vi "main.vi"() -> ()   [LabVIEW 2024]
doc: "Use this template to build a producer/consumer design pattern with events to produce queue items. Use this design pattern instead of the User Interface Event Handler pattern for user interfaces when you want to execute code asynchronously in response to an event without slowing the user interface responsiveness."
uses:
  code/controls/type.eng.settings.ctl
  code/controls/UiStepBuilder.ctl
  code/controls/type.step-builder.ctl
  code/controls/UiProcHeader.ctl
  code/controls/Ui.nrt.flow-panel.ctl
  code/controls/UiNutritionFlowElement.ctl
  code/controls/UiScheduleTimestamp.ctl
  code/controls/typeEnv.ctl
  code/controls/type.StepFunction.ctl
  code/controls/typeXyPoint.ctl
  code/controls/type.address.ctl
  code/controls/enum.io.type.ctl
  code/controls/enum.io.mode.ctl
  code/controls/IONode.ctl
  code/controls/type-io-map-do.ctl
  code/controls/type-io-map-di.ctl
  code/controls/type-io-map-ai.ctl
  code/controls/type-snapshot.ctl
  code/controls/enum-io-sort-type.ctl
  code/controls/wind-dir-view.ctl
  code/controls/windows-panel.ctl
  code/controls/irr-panel.ctl
  code/controls/pbr-func-def.ctl
  code/controls/eng-serial-log.ctl
  code/controls/cluster-com-log.ctl
  code/controls/state-engine.ctl
  code/controls/state-logger.ctl
  code/controls/enum.io-interface.ctl
  code/controls/enum-com-log.ctl
  code/controls/enum.report-filter.ctl
  code/controls/typePathSelector.ctl
  code/controls/ini-key.ctl
  code/controls/typeProcVarientName.ctl
  code/controls/UiNutritionPanel.ctl
  code/controls/enumVarCtrlIO.ctl
  code/controls/type.eng-call.proc-insert.ctl
  code/controls/type.eng.proc.isrunning.ctl
  code/controls/eng-call-do-by-name.ctl
  <vilib>/Utility/error.llb/DialogType.ctl
  <vilib>/Utility/miscctls.llb/LVPointTypeDef.ctl
  <vilib>/Utility/miscctls.llb/LVDateTimeRec.ctl
  code/controls/rio-rx-enum.ctl
  code/controls/type.eng.log-cluster.ctl
  code/controls/typeCmdPostStepFunc.ctl
  code/controls/typeEngineLogCluster.ctl
  code/VIs/Polymorphics/variantCtrlString.vi
  code/VIs/proc.util.validateParamExist.vi
  <vilib>/Utility/error.llb/Trim Whitespace.vi
  <vilib>/Utility/error.llb/Trim Whitespace One-Sided.vi
  code/globals/globals-engine.vi
  <vilib>/Utility/libraryn.llb/Create Directory Recursive.vi
  <vilib>/Utility/config.llb/Read Key (String).vi
  code/VIs/util.error.create.vi
  <vilib>/Utility/config.llb/Read Key (Double).vi
  <vilib>/Utility/config.llb/Read Key (I32).vi
  code/VIs/util-address-builder.vi
  code/VIs/util.DO.ToString.vi
  code/VIs/Polymorphics/io.command-builder.vi
  code/VIs/Polymorphics/io.command-builder.DO.vi
  code/VIs/Polymorphics/io.command-builder.AI.vi
  code/VIs/Polymorphics/io.command-builder.DI.vi
  <vilib>/Utility/config.llb/Write Key (String).vi
  <vilib>/Utility/config.llb/Write Key (Double).vi
  <vilib>/Utility/config.llb/Write Key (I32).vi
  code/controls/typeIniFileSection.ctl
  <vilib>/Utility/file.llb/Read Delimited Spreadsheet (DBL).vi
  <vilib>/Utility/config.llb/NI_LVConfig.lvlib
  <vilib>/Instr/_visa.llb/VISA Find Search Mode.ctl
  <vilib>/Utility/file.llb/Write Delimited Spreadsheet (DBL).vi
panel:
  out "clock 3":string="12:34:56"
  out "COM Size":i64 format="IOs: %d"
  out "COM FIFO":i32 format="QCom: %d"
  out "LOG FIFO 2":i32 format="QLog: %d"
  out "ENG FIFO 2":i32 format="QEng: %d"
  in  "Cluster":cluster{"MAIN":bool, "I/O":bool, "ADMIN":bool}
  out "DayNight":bool
  in  "ENG ms ctrl 28":i32=300 caption="Runtime Interval" format="Runtime:  %d [ms]"
  in  "ENG ms ctrl 15":i32=300 caption="Runtime Interval" format="Runtime:  %d [ms]"
  in  "ENG ms ctrl 14":i32=300 caption="Runtime Interval" format="Runtime:  %d [ms]"
  in  "ENG ms ctrl 13":i32=300 caption="Runtime Interval" format="Runtime:  %d [ms]"
  in  "ENG ms ctrl 12":i32=300 caption="Runtime Interval" format="Runtime:  %d [ms]"
  in  "ENG ms ctrl 11":i32=300 caption="Runtime Interval" format="Runtime:  %d [ms]"
  in  "ENG ms ctrl 10":i32=300 caption="Runtime Interval" format="Runtime:  %d [ms]"
  in  "ENG ms ctrl 9":i32=300 caption="Runtime Interval" format="Runtime:  %d [ms]"
  in  "ENG ms ctrl 8":i32=300 caption="Runtime Interval" format="Runtime:  %d [ms]"
  in  "Admin Panel":bool
  out "Waveform Chart":dbl(graph)
  out "User messages":string
  out "error out":errorcluster
  in  "Timer Reset?":bool
  out "userName":string="USER"
  out "projectName":string="NAME"
  in  "ENV":T1=enum."ENV.TEST.SINGLE-02"
  out "clock":string="12:34:56"
  in  "Enable Report":bool
  in  "Tab Control 2":T2(tab)
  in  "EngLogClear":bool
  out "Collected Reports":string
  out "Collected Reports 2":string
  in  "VISA REPORT":T4={"visa report"=[["Range", "High", "Low", "25", "FULL"], ["", "", "", "", ""], ["", "", "", "", ""], ["", "", "", "", ""], ["", "", "", "", ""], ["", "", "", "", ""], ["", "", "", "", ""], ["", "", "", "", ""], ["", "", "", "", ""]], "RIO Address"=0, "IOtype"=enum."AI", "VISA Report En"=FALSE, "Clear"=FALSE, "Only Errors?"=FALSE} {"RIO Address" min=-1 max=31 step=1 format="RIO: %02d"}
  out "SelectedPath":path
  out "case":T5
  in  "Clk Simulator":timestamp format="%<%x %.1X>T"
  in  "Simulate Clock Reset":bool
  out "Clock Simulation":bool
  in  "Time Addition":dbl
  out "AI":dbl[][](array[numeric]) format="%#.1f"
  in  "Calib?":bool
  out "Log":i32 format="%#_3p"
  out "Eng":i32 format="%#_3p"
  out "Event":i32 format="%#_3p"
  out "Com":i32 format="%.0p"
  out "Report General":T7(array[cluster]) {"clk" format="%#.1f"}
  in  "Log Clear":bool
  in  "Proc Name":string(combo)
  in  "DO Set by Addr":T9 {"ADDR" format="%04d"}
  in  "DO Set by Name":T10={"State"=FALSE, "Name"="Name...", "Timeout [s]"=8, "Send"=FALSE}
  in  "SerialPort":refnum<visa-resource-name>="COM12"
  in  "MenuRuntime":T11={"Run"=FALSE, "Step"=FALSE, "Load"=FALSE, "Status"=FALSE, "Unload"=FALSE, "Reload"=FALSE, "Stop"=FALSE, "ProcedureReload"=FALSE, "ProcedureStep"=FALSE, "ProcedureSelect"="set-dout", "ProcedureRun"=FALSE}
  out "Simulated":string[](array[string])
  in  "ProjectSettings":T12={"Project Name"="Yogiland", "Latitude"=0.0, "Longitude"=0.0, "TimeZone"=0, "userName"="Yogiland"} {"Longitude" format="%#.6g"; "Latitude" format="%#.6g"}
  out "RIO Snapshots":T13[](array[typedef]) {"Dports" format="%08x"}
  in  "Tab Main":enum32{"MAIN", "I/O", "ADMIN"}(tab)
  in  "Button":bool
  in  "Section":string(combo)
  in  "Tab NTR":T14(tab)
  in  "NTR Flowchart":T15={"WASH_IN"={"boolean"=FALSE, "Message"="25/150"}, "EC"={"boolean"=TRUE, "Message"="L Alarm"}, "PH"={"boolean"=TRUE, "Message"="Low"}, "ORP"={"boolean"=TRUE, "Message"="Range"}, "W_TEMP"={"boolean"=TRUE, "Message"="25"}, "W_LEVEL"={"boolean"=TRUE, "Message"="FULL"}, "ALFA1"={"boolean"=TRUE, "Message"="60/60"}, "BETA1"={"boolean"=TRUE, "Message"="25/60"}, "ALFA2"={"boolean"=FALSE, "Message"="0/0"}, "BETA2"={"boolean"=FALSE, "Message"="0/0"}, "ACID"={"boolean"=FALSE, "Message"="0/60"}, "BASE"={"boolean"=FALSE, "Message"="0/50"}, "WATER"={"boolean"=FALSE, "Message"="0/150"}, "WASH_OUT"={"boolean"=FALSE, "Message"="ss"}, "UNIT"={"boolean"=FALSE, "Message"="0"}, "ORPMIX"={"boolean"=FALSE, "Message"="0/150"}}
  out "ntr.status-table":string[][](table)=[["Range", "High", "Low", "25", "FULL"], ["", "", "", "", ""], ["", "", "", "", ""], ["", "", "", "", ""], ["", "", "", "", ""], ["", "", "", "", ""], ["", "", "", "", ""], ["", "", "", "", ""], ["", "", "", "", ""]]
  out "NTR Status":string="Nutrition Status: Processing Unit "
  in  "ntrGraphPeriod":T18 {"lastDays" format="Last %d Days"; "Time range"."Start" format="From: %<%d/%m/%y>T"; "Time range"."End" format="To: %<%d/%m/%y>T"}
  out "Nutrition Sensor Graph":cluster{"X":dbl[], "Y":dbl[]}(graph)
  out "EC 3":cluster{"X":dbl[], "Y":dbl[]}(graph)
  in  "ntrDosepumpSelect":string(combo)
  in  "ntrInputSelect":string(combo)
  in  "Irrigation status":string="Irrigation Status"
  out "Solar Elevation Graph":waveform(dbl)(graph)
  in  "UiProjectSettings":T19 {"Longitude" format="%#.6g"; "Latitude" format="%#.6g"}
  in  "GoToCam 2":bool
  in  "GoToCam":bool
  in  "Cluster 2":T20
  in  "camera":u16(ring) items=["Camera 1", "Camera 2"]
  in  "start":T17 caption="Open" format="%<%H:%M>T"
  out "last":T17 caption="Open" format="Last Harvest %<%H:%M:%S %d/%m/%y>T"
  in  "PRBmenu":cluster{"Harvest":bool, "SANI":bool}
  in  "PbrView 2":T21 {"Unit Storage"."col" scale=0.0..1.0; "Unit Storage"."?" scale=0.0..1.0; "Unit Storage"."?" scale=0.0..1.0; "Unit Column"."col" scale=0.0..1.0; "Unit Column"."?" scale=0.0..1.0; "Unit Column"."?" scale=0.0..1.0; "Digester"."Digester 2" scale=0.0..10.0; "Digester"."Digester 1" scale=0.0..10.0; "BIO Mass Tank" scale=0.0..100.0; "Harvest\n Tank" scale=0.0..100.0}
  in  "PBR Builder":T23(array[cluster])
  out "source":string
  in  "PBR_PLAY":cluster{"PLAY":bool, "PAUSE":bool, "STOP":bool}
  in  "PBR PROC":string(combo)
  in  "PBR":T24
  in  "Temperature Graph Panel":T25={"Time range"={"Start"=timestamp(0 s since 1904-01-01), "End"=timestamp(0 s since 1904-01-01)}, "lastDays"=3, "refresh"=FALSE} {"lastDays" min=1 max=99 step=1 format="%d Days"; "Time range"."Start" format="From: %<%d/%m/%y>T"; "Time range"."End" format="To: %<%d/%m/%y>T"}
  out "OutdoorStatus":T26
  out "indoorStatus":T27
  in  "Tab Control 3":T28(tab)
  out "Outdoor Tdry Graph":cluster{"X":dbl[], "Y":dbl[]}[](graph)
  out "RH":cluster{"X":dbl[], "Y":dbl[]}[](graph)
  out "UV Graph":cluster{"X":dbl[], "Y":dbl[]}(graph)
  in  "UVAccHistoryDays":i8=3
  out "UV_ACC":cluster{"X":dbl[], "Y":dbl[]}(graph)
  out "Waveform Chart 2":cluster{dbl, "UV Limit":dbl}(graph)
  in  "UvAccRefresh":bool
  out "UV Graph 2":cluster{"X":dbl[], "Y":dbl[]}(graph)
  out "Wind Dir Panel":T29
  out "UV Acc.":dbl format="%#_3p"
  in  "Tab Auxi":T30(tab)
  in  "IRR Params":T31={"Day Time"={"Sunset"=timestamp(0 s since 1904-01-01), "Sunrise"=timestamp(0 s since 1904-01-01)}, "timeLimits"={"Irrigation"=0.0, "Nut./Water"=0.0}, "Calculated Timing"={"Irrigation Timeout"=timestamp(0 s since 1904-01-01), "Nutrients Timeout"=timestamp(0 s since 1904-01-01)}, "Irr Dosing Time"={"Nutrients"=0, "Water"=0, "Wash"=0}, "UV Limit "=0.0, "Dose Table"=[{"Enable"=FALSE, "output"="IRR_SEC1"}, {"Enable"=FALSE, "output"="IRR_SEC2"}, {"Enable"=FALSE, "output"="IRR_SEC3"}, {"Enable"=FALSE, "output"="IRR_SEC4"}, {"Enable"=FALSE, "output"="IRR_SEC5"}, {"Enable"=FALSE, "output"="IRR_SEC6"}], "Last Iteration"=timestamp(0 s since 1904-01-01), "UV Reduction Status"=FALSE, "UV Reduction"=0} {"UV Reduction" max=99 step=1 format="%d [%%]"; "timeLimits"."Nut./Water" format="%02.2f [hr]"; "timeLimits"."Irrigation" format="%02.2f [hr]"; "Day Time"."Sunrise" format="%<%H:%M:%S>T"; "Day Time"."Sunset" format="%<%H:%M:%S>T"; "Calculated Timing"."Nutrients Timeout" format="%<%H:%M:%S>T"; "Calculated Timing"."Irrigation Timeout" format="%<%H:%M:%S>T"; "UV Limit" format="%#.1p [J/m2]"; "Irr Dosing Time"."Wash" format="%d [s]"; "Irr Dosing Time"."Water" format="%d [s]"; "Irr Dosing Time"."Nutrients" format="%d [s]"; "Last Iteration" format="%<%X %x>T"}
  in  "WinView":T32 {"EastSideView" scale=0.0..100.0; "WestSideView" scale=0.0..8.0; "EastPosition" max=12; "WestPosition" max=12}
  in  "AuxiliaryList":T33(array[cluster]) {"Period" format="Period [s]: %d"; "Pulse" format="Pulse [s]: %d"}
  out "Array 2":cluster{"name":string, "value":string}[](array[cluster])
  in  "NTR Panel":cluster{"CloseAll":bool}
  in  "RFS Enable Table":bool
  in  "RFS Enable Table":T34
  in  "RFS Cycles Set":bool
  in  "RFS Cycles":u16
  out "RFS Cycles":u16
  in  "RFS Cycles Get":bool
  out "RFS Status":string
  in  "RFS SetX1":bool
  in  "TableIndex":u8 max=7 step=1 format="Table: %d"
  in  "RFS SetX8":bool
  in  "RFS Delays":T35
  in  "RFS Address":u8 format="Address: %d"
  out "RFS Cycles Table":T36
  out "elements":cluster{"case":T5, "data":variant}[](array[cluster])
  in  "Tab IO":enum32{"Map", "Editor", "Calibration"}(tab)
  in  "Clear Virtuals":bool
  in  "IO Map Take Snapshot":bool caption="Take Snapshop"
  out "RIO List":cluster{"Address":u8, "Connected":bool}[](array[cluster]) {"Address" format="%02d"}
  in  "Show Undefined":bool
  out "IO Map AI Count":i32
  out "IO Map DI Count":i32
  out "IO Map DO Count":i32
  in  "IO Map DO":T37[](array[typedef]) caption="Digital Outputs" {"ADDR" format="%04d"}
  in  "IO Map AI":T39[](array[typedef]) caption="Analog Inputs" {"ADDR" format="%04d"}
  in  "IO Map DI":T40[](array[typedef]) caption="Digital Inputs" {"ADDR" format="%04d"}
  in  "IO Map Snapshot Enable":bool caption="Auto Snapshop Enable"
  in  "IO Search Map":T41={"By Name"="", "By Tag"="Tags...", "By Address"=0} caption="Search by Name | Tag | Address" {"By Address" min=-1 max=31 step=1 format="RIO: %02d"}
  in  "IO Search Map Refresh":bool
  in  "TimerSec":dbl=5.0 format="%#.1f"
  out "downcount[sec]":dbl format="%#.1g"
  in  "Simulators":cluster{"Input ":string, "Value":string}[](array[cluster])
  in  "IO Map VL":T42[](array[typedef]) caption="Virtual Channels" {"calibration"."Y" format="%#.3f"; "calibration"."X" format="%#.3f"; "ADDR" format="%04d"}
  out "IO Map VL Count":i32
  in  "IO Conf view":enum16{"Show All", "Search"}(ring)
  in  "IOconf Sort":T44
  in  "IO Search Conf":T45={"ADDR"=-1, "Label"="", "Type"=enum."Type", "Mode"=enum."Mode", "Tags"=""} {"ADDR" min=-1 max=99 format="RIO: %02d"}
  in  "IO Conf":T46(array[cluster]) {"calibration"."Y" format="%#.3f"; "calibration"."X" format="%#.3f"; "ADDR" format="%04d"}
  in  "IO List":cluster{"save":bool, "loadCsv":bool}
  in  "New Element":T42={"ADDR"=0, "Label"="Name", "Type"=enum."DI", "Mode"=enum."RIO", "Value"="Value", "Tags"="Tags", "calibration"=[]} {"calibration"."Y" format="%#.3f"; "calibration"."X" format="%#.3f"; "ADDR" format="%04d"}
  in  "IO Add New":bool
  out "size":i32 format="Count: %d"
  out "Value (Y)":dbl
  out "Raw (X)":dbl
  in  "IO calib save":bool
  in  "IO calib select":string(combo)
  in  "XyPairs":T43[](array[typedef]) {"Y" format="%#.3f"}
  out "error":errorcluster
  out "Chart":cluster{"unCalibrated":u16, "Value out":dbl}(graph)
  in  "Tab Control":enum32{"Settings", "Builder", "Snapshot"}(tab)
  out "App Started at":timestamp format="%<%x %.3X>T"
  out "Loaded":cluster{"Procedure":variant[]}[](array[cluster]) caption="Loaded Procedures"
  in  "ENG ms":i32=-1 caption="Interval"
  in  "Title Bar Visible":bool
  in  "ENG ms ctrl":i32=300 caption="Runtime Interval" format="Runtime:  %d [ms]"
  in  "EVENT ms":i32=100 format="%d [ms]"
  out "Type":u8 format="%.0x"
  out "Address":u8 format="%.0x"
  in  "read buffer":string
  out "Command Payload":string
  out "AI uncalib out":u16
  out "AI out":dbl
  out "Data Size":u8
  out "monitor":errorcluster[](array[cluster])
  out "record":errorcluster[](array[cluster])
  out "control":errorcluster[](array[cluster])
  in  "Template":T47
  in  "UiBuildProcHead":T48={"Procedure Name"="MyProcExample", "Running"=TRUE, "tags"="MyProcExample"}
  in  "Loaded Proc Path":string[](array[string])
  in  "UiBuildSteps":T49[](array[typedef])
  in  "File path":path
  out "UiBuildSteps 2":T49[](array[typedef])
  in  "Proc Select 2":string(combo)
  out "Serial Log Size":i32
  out "COM Snapshot":T51[](array[typedef])
  in  "Snapshot Size":i64=1000
  in  "COM":bool
  in  "filter":T52={"Status"=0, "Date"="", "Caller"="", "Type"="", "IOname"="", "Calib"="", "Uncalib"="", "Vsdt"="Vsdt", "StatusMsg"=""}
  out "Serial Record(s)":T53[](array[typedef]) {"IOnode"."calibration"."Y" format="%#.3f"; "IOnode"."calibration"."X" format="%#.3f"; "IOnode"."ADDR" format="%04d"}
  # "Outoor"
  # "Indoor"
  # "UV Accumulator"
  # "Nutrition"
  # "Nutrition History"
  # "Nursery"
  # "Camera Robot"
  # "PBR"
  # "- Fully Open"
  # "- Fully Close"
  # "W"
  # "E"
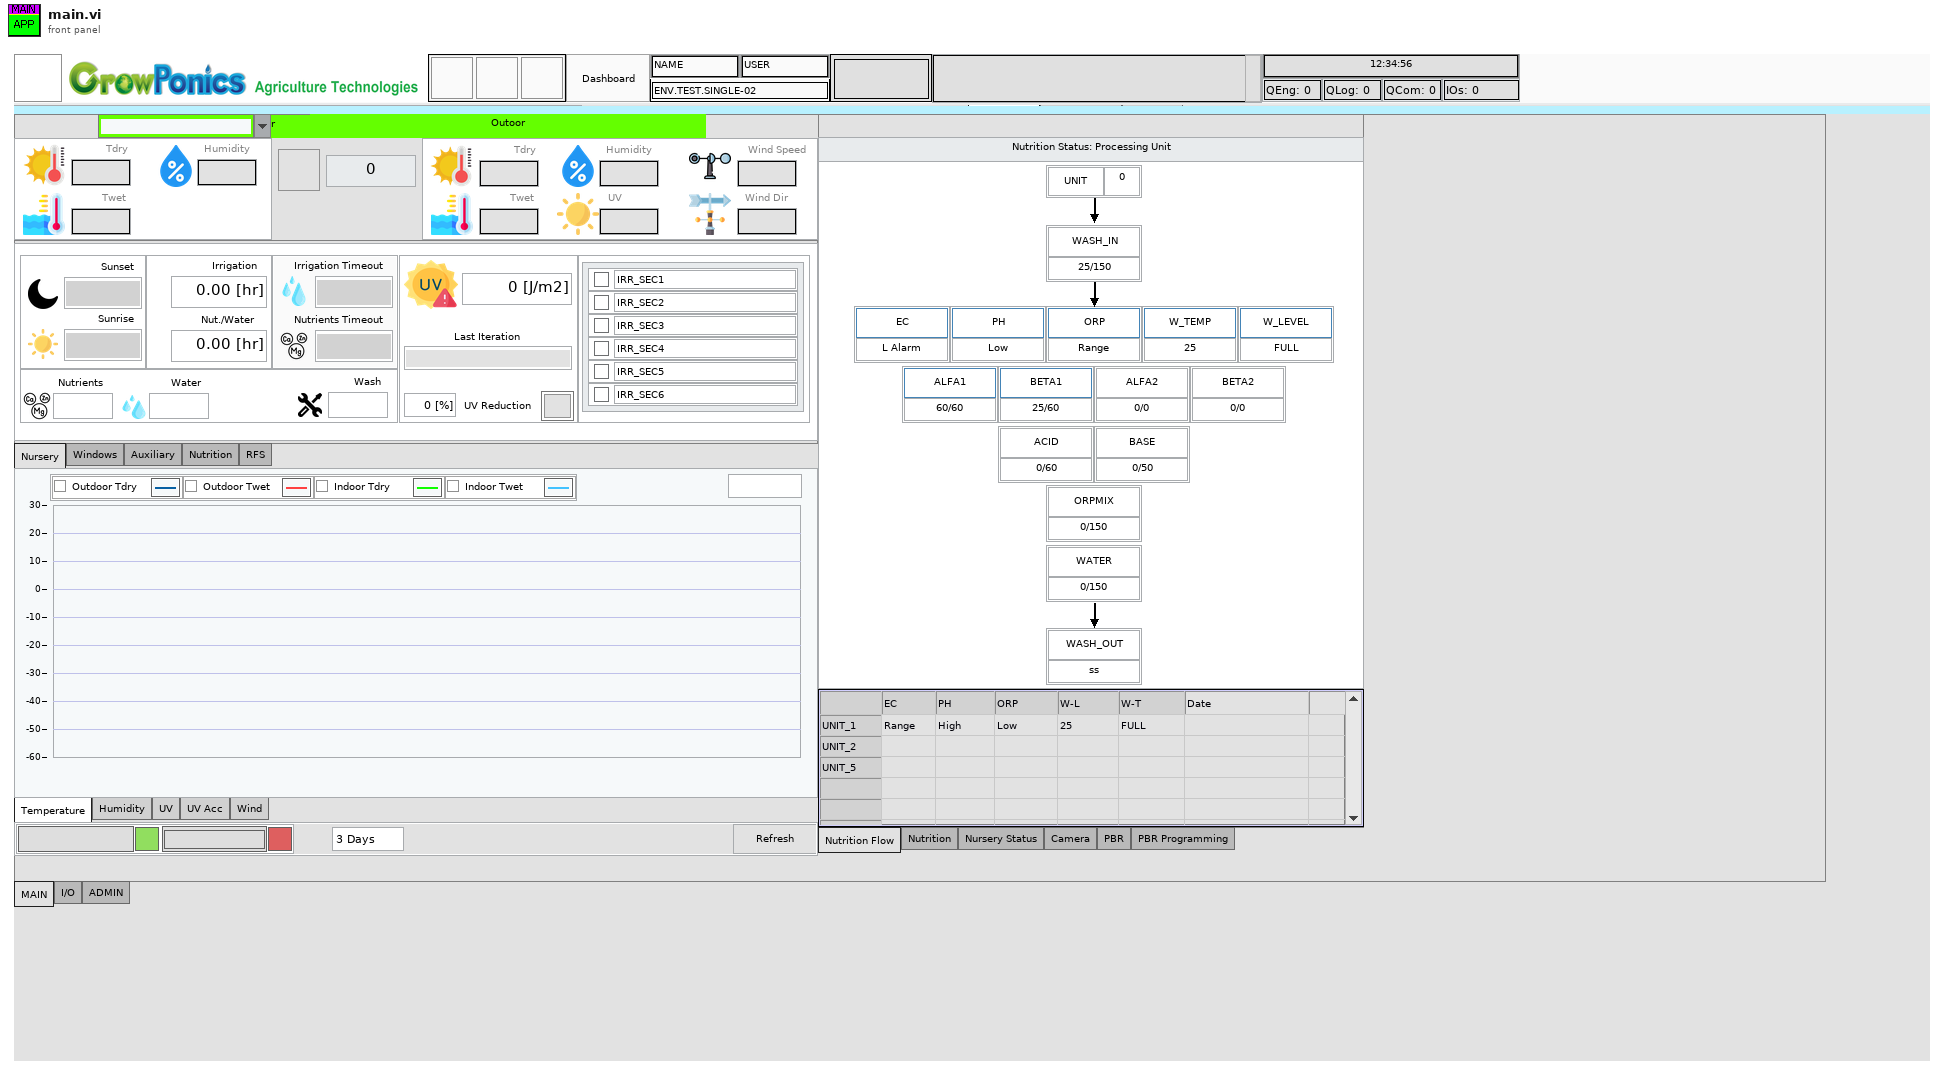
[diagram p1: front panel]
types:
  T1 = typedef "typeEnv.ctl" = enum16{"ENV.PRODUCTION", "ENV.TEST.NO-HW", "ENV.TEST.SINGLE-01", "ENV.TEST.SINGLE-02", "ENV.TEST.SINGLE-02 AI 0", "ENV.TEST.SINGLE-03"}
  T2 = enum32{"System Log", "Runtime Flow", "Iterations"}
  T3 = typedef "enum.io.type.ctl" = enum16{"Type", "DI", "DO", "AI", "AO", "VL", "BUF"}
  T4 = cluster{"visa report":string[][], "RIO Address":i32, "IOtype":T3, "VISA Report En":bool, "Clear":bool, "Only Errors?":bool}
  T5 = typedef "state-engine.ctl" = enum16{"ENG.NO-OP", "ENG.START", "ENG.STOP", "ENG.EXECUTE", "ENG.STATUS", "ENG.EXTERNAL-CALL", "ENG.INIT", "ENG.INIT.VARS", "ENG.INIT.SERIAL", "ENG.LOAD", "ENG.LOAD.SINGLE", "ENG.LOAD.MODULE", "ENG.LOAD.RELOAD", "ENG.LOAD.UNLOAD", "ENG.IO.LOAD", "ENG.IO.SAVE", "ENG.PROC.RELOAD-BY-NAME", "ENG.PROC.START", "ENG.PROC.STOP", "ENG.PROC.INSERT-STEPS", "ENG.PROC.ISRUNNING", "ENG.PROC.PRESET", "ENG.PROC.STATUS", "ENG.PRINT-USER-MSG", "ENG.RIO.SNAPSHOT", "ENG.RIO.AIN-SNAPSHOT-CALIB", "ENG.RIO.DOUT-BY-ADDR", "ENG.RIO.DOUT-BY-NAME", "ENG.RIO.RFS-DELAY-SET-X1", "ENG.RIO.RFS-DELAY-SET-X8", "ENG.RIO.RFS-CYCLES-SET", "ENG.RIO.RFS-CYCLES-GET", "ENG.RIO.RFS-ENABLE", "ENG.EXIT"}
  T6 = typedef "type.StepFunction.ctl" = enum16{"__NO-OP", "_DELAY_LOAD", "_DELAY_COMPARE", "_JUMP", "_COMPLETE", "_COMPARE", "_LOG_MESSAGE", "_LOG_LAST_REPORT", "_SCHEDULE", "_SCHED_DAILY", "CLK_COMPARE", "PROC_START", "PROC_STOP", "PROC_LOAD", "PROC_COMPLETION_CHECK", "PROC_COMPLETION_LOAD", "_IO_READ", "_IO_READ_MANY", "_IO_WRITE", "_IO_WRITE_BY_REG", "_IO_GET_OUTPUT", "_OCS_CHECK", "_OCS_RECORD", "_GET_RH", "_GET_ACC_UV", "_GET_WD", "_GET_WS", "_REC_DELETE", "_REC_MOVE", "_REC_COPY", "_IRR_CHECK", "UNIT_CHECK", "UNIT_SAMPLE", "UNIT_DOSE"}
  T7 = cluster{"ErrorFlag":bool, "idx":i32, "Step Name":string, "Step Function":T6, "Report":string, "clk":dbl, "Step Name 2":string}[]
  T8 = typedef "type.address.ctl" = u16
  T9 = cluster{"State":bool, "ADDR":T8, "Timeout [s]":u8, "Send":bool}
  T10 = cluster{"State":bool, "Name":string, "Timeout [s]":u8, "Send":bool}
  T11 = cluster{"Run":bool, "Step":bool, "Load":bool, "Status":bool, "Unload":bool, "Reload":bool, "Stop":bool, "ProcedureReload":bool, "ProcedureStep":bool, "ProcedureSelect":string, "ProcedureRun":bool}
  T12 = typedef "type.eng.settings.ctl" = cluster{"Project Name":string, "Latitude":dbl, "Longitude":dbl, "TimeZone":i32, "userName":string}
  T13 = typedef "type-snapshot.ctl" = cluster{"Address":u8, "DI":bool[], "status":errorcluster, "AI":dbl[], "Dports":u32, "AI RAW":dbl[]}
  T14 = enum32{"Nutrition Flow", "Nutrition", "Nursery Status", "Camera", "PBR", "PBR Programming"}
  T15 = typedef "Ui.nrt.flow-panel.ctl" = cluster{"WASH_IN":T16, "EC":T16, "PH":T16, "ORP":T16, "W_TEMP":T16, "W_LEVEL":T16, "ALFA1":T16, "BETA1":T16, "ALFA2":T16, "BETA2":T16, "ACID":T16, "BASE":T16, "WATER":T16, "WASH_OUT":T16, "UNIT":cluster{"boolean":bool, "Message":string}, "ORPMIX":T16}
  T16 = typedef "UiNutritionFlowElement.ctl" = cluster{"boolean":bool, "Message":string}
  T17 = typedef "UiScheduleTimestamp.ctl" = timestamp
  T18 = cluster{"Time range":cluster{"Start":T17, "End":T17}, "lastDays":dbl, "refresh":bool}
  T19 = cluster{"Latitude":dbl, "Longitude":dbl, "TimeZone":i32}
  T20 = cluster{"Next Button":bool, "Previous Button":bool, "Up Button":bool, "Down Button":bool, "Home":bool}
  T21 = cluster{"Unit Storage":cluster{dbl, dbl, "col":dbl}, "Unit Column":cluster{dbl, dbl, "col":dbl}, "Ui_TANKOUT":bool, "Column":dbl, "Ui MAIN\nUi_COLOUT\nUi_PUMP":bool, "Digester":cluster{"Digester 1":dbl, "Digester 2":dbl}, "DO 4":bool, "Flow Out DI":bool, "BIO Mass Tank":dbl, "DO Membrane":bool, "MEDIUM":bool, "WATER":bool, "Ui_TANKIN":bool, "Harvest\n Tank":dbl, "HARVEST":bool}
  T22 = typedef "pbr-func-def.ctl" = enum16{"DELAY SEC", "SENSE", "PROC START", "PROC WAIT", "SET OUTPUT", "FINISH"}
  T23 = cluster{"Operation":T22, "Param":string, "uid":string}[]
  T24 = cluster{"LOAD":bool, "SAVE":bool, "COMPILE":bool, "SAVEAS":bool}
  T25 = cluster{"Time range":cluster{"Start":T17, "End":T17}, "lastDays":i8, "refresh":bool}
  T26 = cluster{"Tdry":string, "Twet":string, "UV":string, "Humidity":string, "Wind Speed":string, "Wind Direction":string}
  T27 = cluster{"Tdry":string, "Twet":string, "Humidity":string}
  T28 = enum32{"Temperature", "Humidity", "UV", "UV Acc", "Wind"}
  T29 = typedef "wind-dir-view.ctl" = cluster{"SE":bool, "SW":bool, "NE":bool, "NW":bool, "W":bool, "E":bool, "S":bool, "N":bool}
  T30 = enum32{"Nursery", "Windows", "Auxiliary", "Nutrition", "RFS"}
  T31 = typedef "irr-panel.ctl" = cluster{"Day Time":cluster{"Sunset":timestamp, "Sunrise":timestamp}, "timeLimits":cluster{"Irrigation":dbl, "Nut./Water":dbl}, "Calculated Timing":cluster{"Irrigation Timeout":timestamp, "Nutrients Timeout":timestamp}, "Irr Dosing Time":cluster{"Nutrients":u16, "Water":u16, "Wash":u16}, "UV Limit ":dbl, "Dose Table":cluster{"Enable":bool, "output":string}[], "Last Iteration":timestamp, "UV Reduction Status":bool, "UV Reduction":u8}
  T32 = typedef "windows-panel.ctl" = cluster{"EastPosition":u16, "WestPosition":u16, "Wind Direction":string, "CloseAll":bool, "WestSideView":u16, "EastSideView":u16, "Wind Speed":string, "confs":cluster{"Full Open [sec]":u16, "Full Close [sec]":u16, "Stages":u16}}
  T33 = cluster{"Source":string, "SourceStatus":bool, "Dest":string, "DestStatus":bool, "Pulse":u16, "Period":u16, "Proc Name":string}[]
  T34 = cluster{"[0]":bool, "[1]":bool, "[2]":bool, "[3]":bool, "[4]":bool, "[5]":bool, "[6]":bool, "[7]":bool}
  T35 = cluster{"Delay Y":u8, "Delay X1":u8, "Delay X2":u8, "Delay CT":u8}
  T36 = cluster{"[0]":u16, "[1]":u16, "[2]":u16, "[3]":u16, "[4]":u16, "[5]":u16, "[6]":u16, "[7]":u16}
  T37 = typedef "type-io-map-do.ctl" = cluster{"ADDR":T8, "Label":string, "Mode":T38, "Value":string, "State":bool}
  T38 = typedef "enum.io.mode.ctl" = enum16{"Mode", "RIO", "SIM"}
  T39 = typedef "type-io-map-ai.ctl" = cluster{"ADDR":T8, "Label":string, "Mode":T38, "Value":string}
  T40 = typedef "type-io-map-di.ctl" = cluster{"ADDR":T8, "Label":string, "Mode":T38, "State":bool, "Value":string}
  T41 = cluster{"By Name":string, "By Tag":string, "By Address":i32}
  T42 = typedef "IONode.ctl" = cluster{"ADDR":T8, "Label":string, "Type":T3, "Mode":T38, "Value":string, "Tags":string, "calibration":T43[]}
  T43 = typedef "typeXyPoint.ctl" = cluster{"X":dbl, "Y":dbl}
  T44 = typedef "enum-io-sort-type.ctl" = enum16{"Sort By Address", "Sort By Name"}
  T45 = cluster{"ADDR":i8, "Label":string, "Type":T3, "Mode":T38, "Tags":string}
  T46 = cluster{"ADDR":T8, "Label":string, "Type":T3, "Mode":T38, "Value":string, "Tags":string, "calibration":T43[]}[]
  T47 = cluster{"templateSave":bool, "templateLoad":bool, "procedureLoad":bool, "procedureSaveAs":bool, "procedureSave":bool, "procedureReload":bool}
  T48 = typedef "UiProcHeader.ctl" = cluster{"Procedure Name":string, "Running":bool, "tags":string}
  T49 = typedef "UiStepBuilder.ctl" = cluster{"Step Function":T50, "ParamString":string, "Step Label":string}
  T50 = typedef "type.step-builder.ctl" = enum16{"NO_OPERATION", "DELAY-JUMP", "DELAY", "JUMP", "COMPLETE", "SCHEDULER", "IRR-CHECK", "UNIT-CHECK", "UNIT-SAMPLE", "UNIT-DOSE", "LOG-REPORT", "LOG-MESSAGE", "IO-READ", "IO-READ-MANY", "IO-WRITE", "IO-COMPARE-OUT", "IO-COMPARE-IN", "PROC-START", "PROC-STOP", "PROC-LOAD", "PROC-IS-COMPLETED", "RECORD-MOVE", "GET-RH", "GET-UV", "GET-WD", "GET-WS", "OCS-CHECK", "OCS-RECORD"}
  T51 = typedef "eng-serial-log.ctl" = cluster{"Status":u32, "Date":string, "Caller":string, "Type":string, "IOname":string, "Calib":string, "Uncalib":string, "Vsdt":string, "StatusMsg":string}
  T52 = cluster{"Status":u32, "Date":string, "Caller":string, "Type":string, "IOname":string, "Calib":string, "Uncalib":string, "Vsdt":string, "StatusMsg":string}
  T53 = typedef "cluster-com-log.ctl" = cluster{"Caller":string, "IOnode":T42, "error":errorcluster, "dports":bool[], "AIN (calib)":dbl, "AIN (raw)":u16, "Times Stamp":timestamp, "Record File Path":path, "Visa Data":string}
  T54 = typedef "enum-com-log.ctl" = enum16{"REC.NO_OP", "REC.INIT", "REC.EXIT", "REC.SERIAL", "REC.IO", "REC.FETCH", "REC.OPEN-FILE", "REC.REOPEN-FILE"}
  T55 = typedef "enum.io-interface.ctl" = enum16{"IO_VISA_WR-RD", "IO_VISA_OPEN", "IO_VISA_CLOSE", "IO_VISA_CLEAR"}
  T56 = typedef "state-logger.ctl" = enum16{"LOG.NO_OP", "LOG.INIT", "LOG.INIT.NTR-FLOW", "LOG.EXIT", "LOG.CATCH", "LOG.PARSE.OCS", "LOG.UPDATE.SELECTORS", "LOG.UPDATE.IRR", "LOG.SNAPSHOT.PROC", "LOG.SNAPSHOT"}
  T57 = enum32{"Invalid", "Standard", "Closed", "Hidden", "Minimized", "Maximized"}
  T58 = typedef "ini-key.ctl" = enum16{"INI.PROJECT_NAME", "INI.ENV", "INI.ENG.SERIAL", "INI.ENG.INTERVAL_MS", "INI.LOCAL.LONGITUDE", "INI.LOCAL.LATITUDE", "INI.LOCAL.TIMEZONE"}
  T59 = typedef "typePathSelector.ctl" = enum16{"DIR_PROCS", "DIR_CONFIG", "DIR_TEMPLATE", "DIR_IO_FILE", "DIR_RECORD", "DIR_LOG", "DIR_RUNTIME", "DIR_PRESET", "DIR_INI"}
  T60 = typedef "enum.report-filter.ctl" = enum16{"Read ALL", "Read Errors", "Collect", "ClearAll"}
  T61 = typedef "typeINIKey.ctl" = string
  T62 = typedef "typeIniFileSection.ctl" = string
  T63 = typedef "NI_LVConfig.lvlib/Config Data RefNum.ctl" = refnum<k1>
  T64 = typedef "UiNutritionPanel.ctl" = cluster{"Main":cluster{"Enable":bool, "WashTimes":cluster{"In":dbl, "Out":dbl}, "DailyActivityHours":cluster{"Begin Time":T17, "End Time":T17}[]}, "Water Dosing":cluster{"Water Dose":dbl, "Water Limit":dbl}, "EC Ranges":cluster{"H Alarm":dbl, "L Alarm":dbl, "Low":dbl}, "EC Dosing":cluster{"ALFA1 Dose":dbl, "ALFA1 Limit":dbl, "BETA1 Dose":dbl, "BETA1 Limit":dbl, "ALFA2 Dose":dbl, "ALFA2 Limit":dbl, "BETA2 Dose":dbl, "BETA2 Limit":dbl}, "PH Ranges":cluster{"H Alarm":dbl, "L Alarm":dbl, "High":dbl, "Low":dbl}, "PH Dosing":cluster{"ACID Dose":dbl, "ACID Limit":dbl, "BASE Dose":dbl, "BASE Limit":dbl}, "ORP Ranges":cluster{"H Alarm":dbl, "L Alarm":dbl, "Low":dbl}, "ORP Dosing":cluster{"MIX Dose":dbl, "MIX Limit":dbl}}
  T65 = enum16{"Always On", "Always Off", "Off While Running"}
  T66 = typedef "LVPointTypeDef.ctl" = cluster{"Horizontal":i16, "Vertical":i16}
  T67 = enum32{"Nutrition Flow", "Nutrition", "Nursery Status", "Camera", "PBR"}
  T68 = typedef "enumVarCtrlIO.ctl" = enum16{"IO Get By Key", "IO List Configs", "IO Add By Key", "IO Modify Value By Key", "IO Modify Calib By Key", "IO Modify ADDR By Key", "IO Modify Mode By Key", "IO Modify Type By Key", "IO Modify Name By Key", "IO Remove By Key", "IO Remove All"}
  T69 = cluster{"Device":i8, "Label":string, "Type":T3, "Mode":T38, "Tags":string}
  T70 = cluster{"State":bool, "Timeout":u16, "Name":string}
  T71 = enum8{"Enabled", "Disabled", "Disabled and Grayed Out"}
  T72 = cluster{"ADDR":u8, "Label":string, "Type":T3, "Mode":T38, "Tags":string}
  T73 = typedef "LVDateTimeRec.ctl" = cluster{"fractional second":dbl, "second":i32, "minute":i32, "hour":i32, "day of month":i32, "month":i32, "year":i32, "day of week":i32, "day of year":i32, "DST":i32}
  T74 = typedef "DialogType.ctl" = u16
  T75 = cluster{"ADDR":bool, "Label":bool, "Mode":bool, "Value":bool, "State":bool}[]
  T76 = cluster{"ADDR":bool, "Label":bool, "Mode":bool, "Value":bool, "State":bool}
  T77 = typedef "UiCompactReport.ctl" = cluster{"ErrorFlag":bool, "idx":i32, "Step Name":string, "Step Function":T6, "Report":string, "clk":dbl, "Proc":string}
  T78 = enum16{"Left Button", "Center Button", "Right Button", "Window Close"}
  T79 = typedef "rio-rx-enum.ctl" = u16
  T80 = enum32{"Bad", "Idle", "Run top level", "Running"}
  T81 = cluster{"Q-Log":refnum<queue>, "procQ":cluster{"data":variant, "Enum":T56}}
  T82 = typedef "type.eng.log-cluster.ctl" = cluster{"Procedure(post)":variant[], "Procedure(pre)":variant[], "Next State ":cluster{"CMD":T83, "data":variant}, "IsRunning":bool, "error in":errorcluster}
  T83 = typedef "typeCmdPostStepFunc.ctl" = enum16{"NEXT", "PREV", "JUMP", "STAY", "COMPLETE", "ENGCALL.PROC.START", "ENGCALL.PROC.STOP", "ENGCALL.PROC.COMPLETION-CHECK", "ENGCALL.PROC.INIT", "ERROR"}
  T84 = typedef "typeEngineLogCluster.ctl" = cluster{"Proc Name":string, "ProcPath":string, "Step Name":string, "Step Function":T6, "Step Index":i32, "Report":string, "clk":dbl, "error in":errorcluster, "Log Message":string, "Proc Module":string}
  T85 = typedef "typeProcVarientName.ctl" = enum16{"procNameID", "procModuleID", "procPath", "procIsRunning", "procIndex", "procModule", "procRegisterNumeric", "procRegisterString", "procReport", "procReportPrev", "procCLK", "procStepPointer", "procType"}
  T86 = typedef "wind-directions.ctl" = enum16{"N", "NE", "E", "SE", "S", "SW", "W", "NW"}
  T87 = cluster{"Irrigation Timeout":timestamp, "Fertiliztion Timeout":timestamp}
  T88 = enum16{"open", "replace", "create", "open or create", "replace or create", "replace or create with confirmation"}
  T89 = typedef "type.eng-call.proc-insert.ctl" = cluster{"ProcName":string, "instructions":variant[]}
  T90 = typedef "type.eng.proc.isrunning.ctl" = cluster{"callerProc":string, "procPointer":string}
  T91 = cluster{"operation":enum16{"START", "STOP"}, "procName":string}
  T92 = typedef "eng-call-do-by-name.ctl" = cluster{"State":bool, "Timeout":u16, "Name":string}
  T93 = cluster{"DataSize":u8, "Address":u8, "CMD":u8, "Table Index":u8, "Delay Y":u8, "Delay X1":u8, "Delay X2":u8, "Delay CT":u8}
  T94 = cluster{"DataSize":u8, "Address":u8, "CMD":u8, "Enable":u8}
  T95 = cluster{"DataSize":u8, "Address":u8, "CMD":u8, "Cycles":u16}
  T96 = cluster{cluster{"Procedure":variant[]}, "error":errorcluster}[]
  T97 = typedef "type.aux.ctl" = cluster{"Source":string, "SourceStatus":bool, "Dest":string, "DestStatus":bool, "Pulse":u16, "Period":u16, "Proc Name":string}
  T98 = typedef "VISA Find Search Mode.ctl" = u32
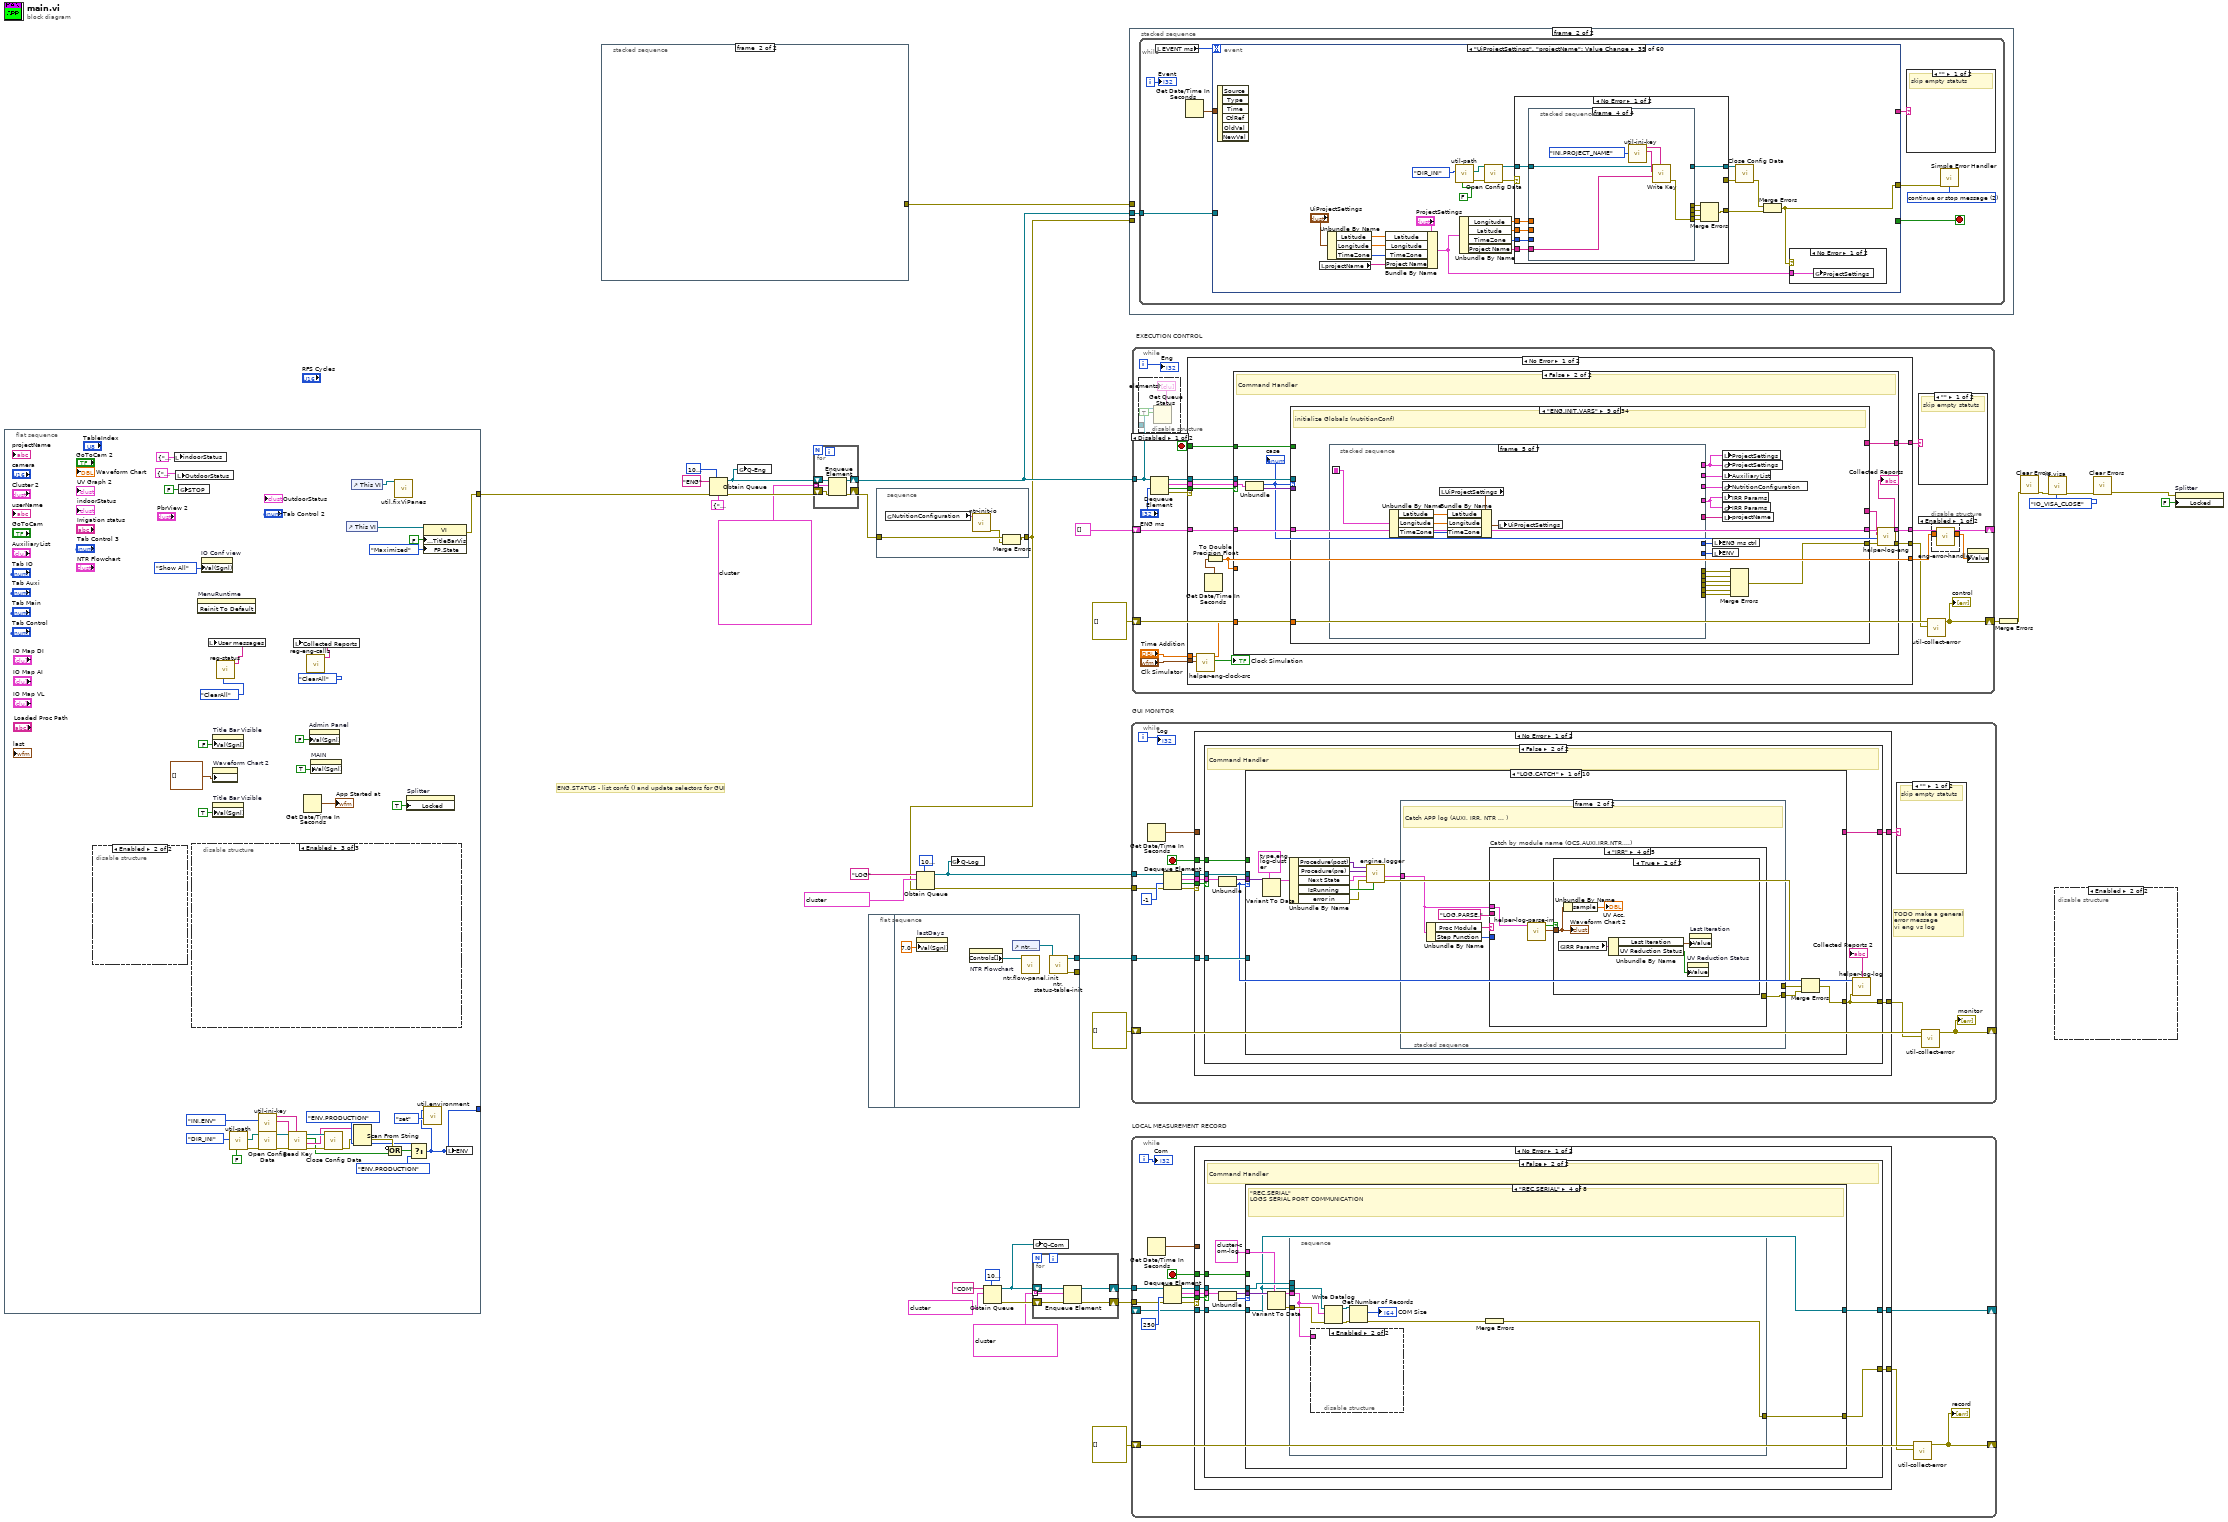
[diagram p0: block diagram]
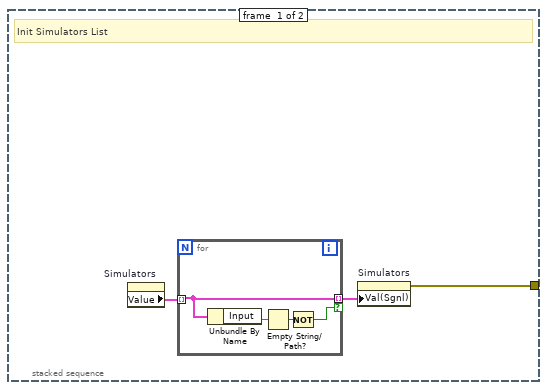
[diagram p2: hidden frame]
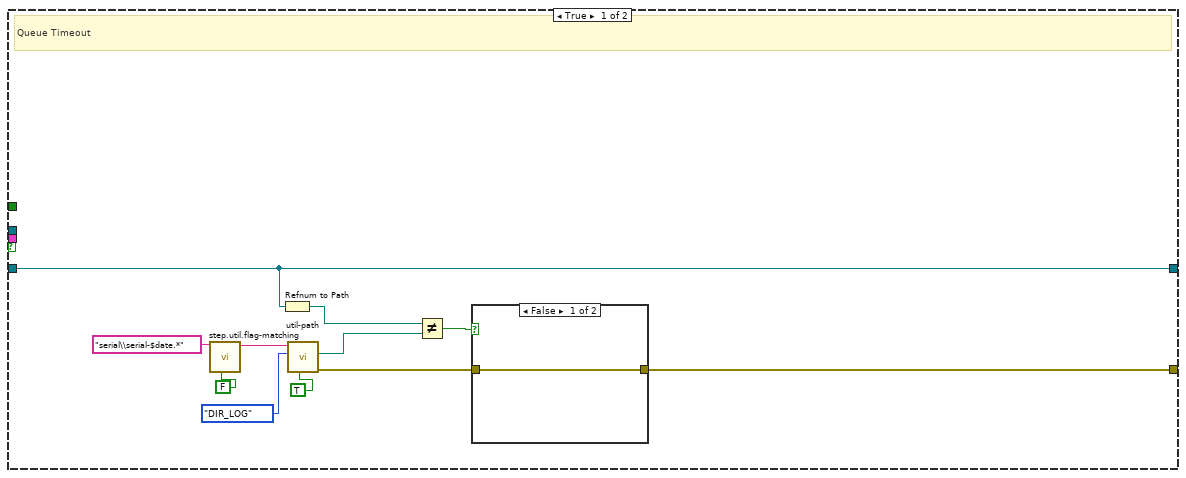
[diagram p3: hidden frame]
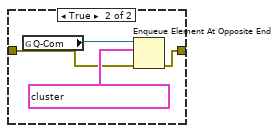
[diagram p4: hidden frame]
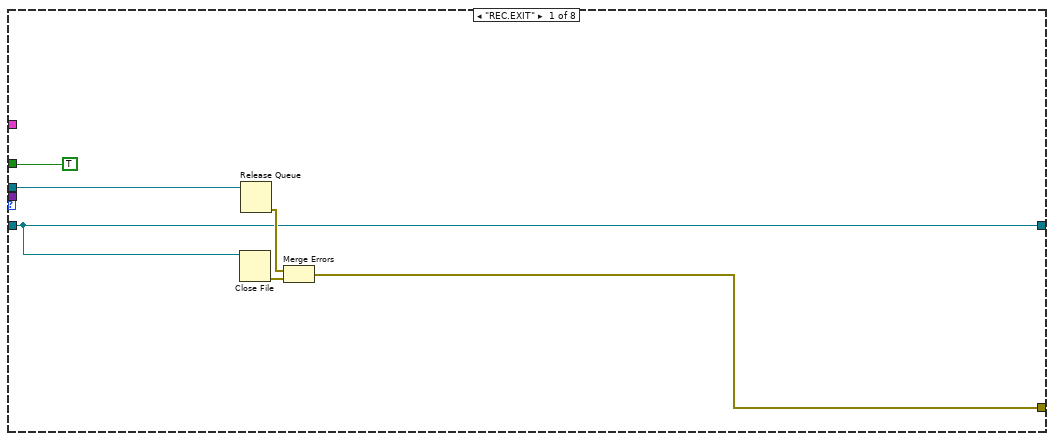
[diagram p5: hidden frame]
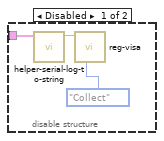
[diagram p8: hidden frame]
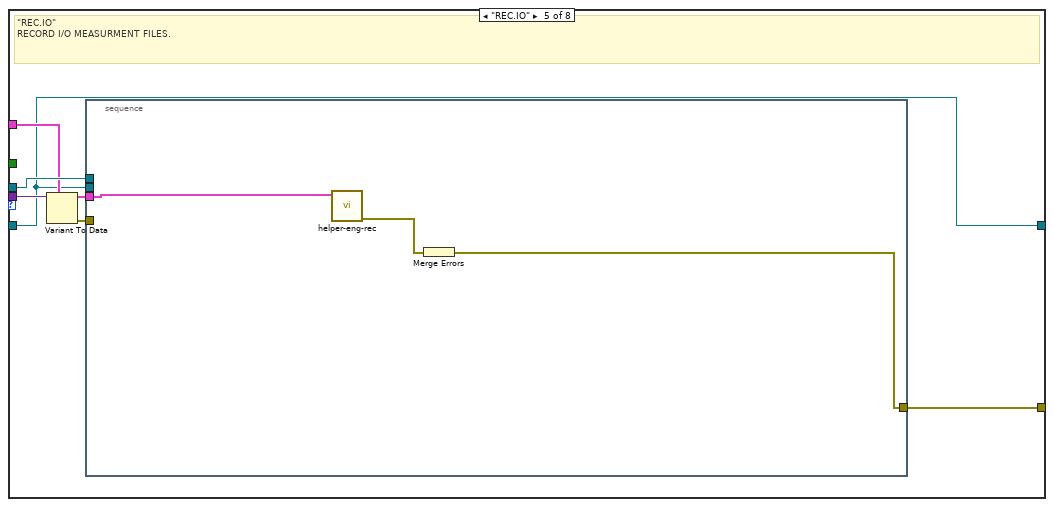
[diagram p9: hidden frame]
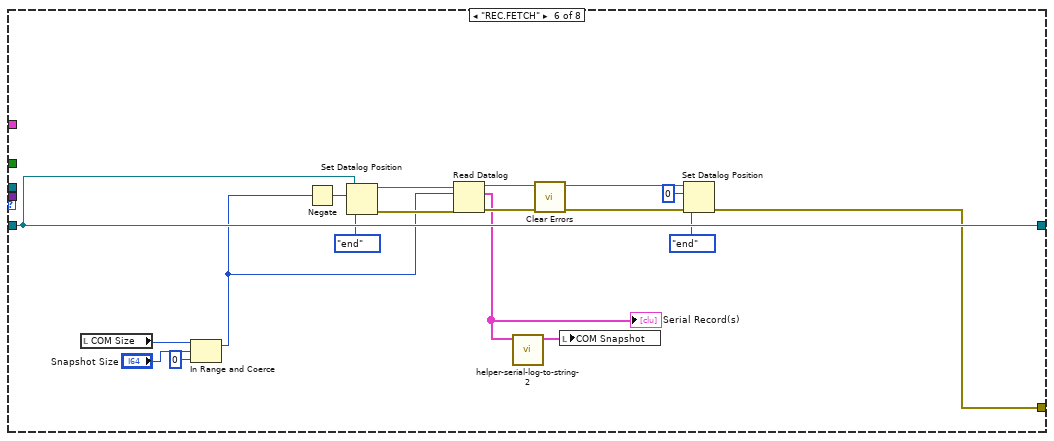
[diagram p10: hidden frame]
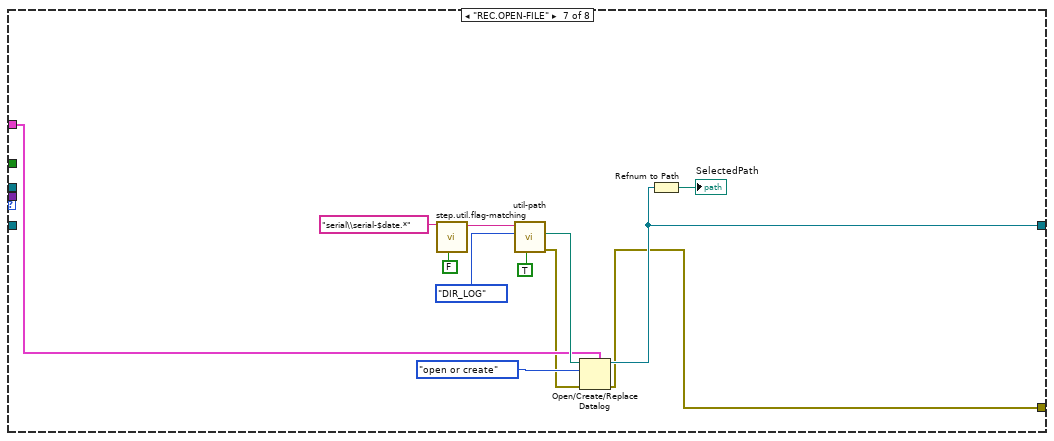
[diagram p11: hidden frame]
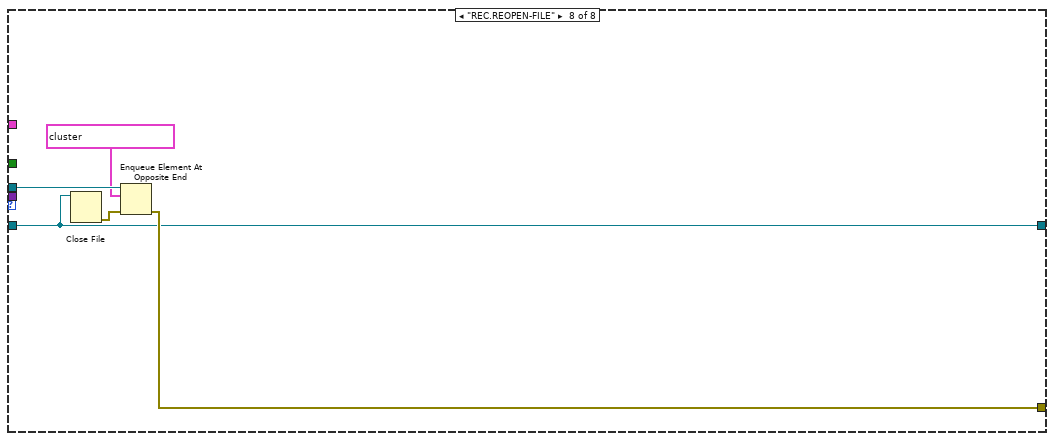
[diagram p12: hidden frame]
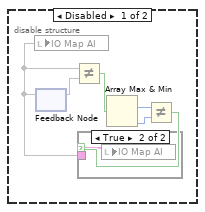
[diagram p14: hidden frame]
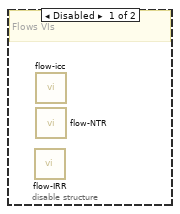
[diagram p16: hidden frame]
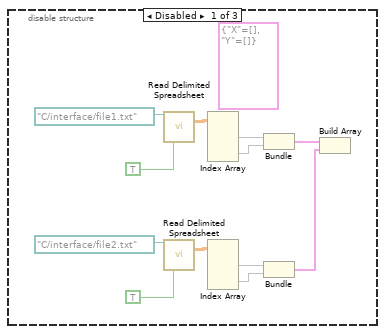
[diagram p17: hidden frame]
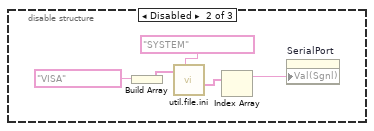
[diagram p18: hidden frame]
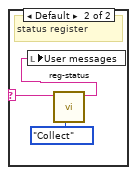
[diagram p19: hidden frame]
diagram:
  # "ENG.STATUS - list confs () and update selectors for GUI"
  n1 = flat-sequence {
    tunnel: [w50] -> _
    tunnel: [w37] -> w7
    frame #0 {
      n2 = disable-structure shown="Enabled" {
        frame Disabled {
          # "Flows VIs"
          n3 = call "flow-IRR.vi"() -> ()  [unwired: 10 in, 2 out]
          n4 = call "flow-icc.vi"() -> ()  [unwired: 11 in, 1 out]
          n5 = call "flow-NTR.vi"() -> ()  [unwired: 11 in, 1 out]
        }
        frame Enabled {
        }
      }
      n6 = local write "indoorStatus"(T27 {"Tdry"="", "Twet"="", "Humidity"=""} ("indoorStatus")) -> ()
      n7 = local write "OutdoorStatus"(T26 {"Tdry"="", "Twet"="", "UV"="", "Humidity"="", "Wind Speed"="", "Wind Direction"=""} ("OutdoorStatus")) -> ()
      n8 = global write "globals-engine.vi" "STOP"(FALSE ("STOP")) -> ()
      n9 = disable-structure shown="Enabled" {
        frame Disabled {
          (unwired) cluster{"X":dbl[], "Y":dbl[]} {"X"=[], "Y"=[]} ("cluster")
          n10 = call-poly <vilib>:"Read Delimited Spreadsheet.vi"("file path (dialog if empty)"=path "C:/interface/file1.txt", "transpose? (F)"=TRUE) -> ("all rows"=w85:dbl[][])  [unwired: 8 in, 5 out]
          n11 = call-poly <vilib>:"Read Delimited Spreadsheet.vi"("file path (dialog if empty)"=path "C:/interface/file2.txt", "transpose? (F)"=TRUE) -> ("all rows"=w82:dbl[][])  [unwired: 8 in, 5 out]
          n12 = Index Array(array=w85) -> (element #1=w80:dbl[], element #2=w79:dbl[])  [unwired: 4 in]
          n13 = Index Array(array=w82) -> (element #1=w83:dbl[], element #2=w78:dbl[])  [unwired: 4 in]
          n14 = Bundle("all rows"=w80, "all rows"=w79) -> (w84:cluster{"all rows":dbl[], "all rows":dbl[]})  [unwired: 1 in]
          n15 = Bundle("all rows"=w83, "all rows"=w78) -> (w81:cluster{"all rows":dbl[], "all rows":dbl[]})  [unwired: 1 in]
          n16 = Build Array(w84, w81) -> ()  [unwired: 1 out]
        }
        frame Disabled {
          n17 = Build Array(T61 "VISA" ("section")) -> (w94:T61[])
          n18 = call "util.file.ini.vi"("Section"=T62 "SYSTEM" ("section"), "keys"=w94) -> ("values"=w93:string[])  [unwired: 7 in, 2 out]
          n19 = Index Array(array=w93) -> (element=w92:string)  [unwired: 1 in]
          n20 = property on="SerialPort" class="VISAName"("Val(Sgnl)"=w92) -> ()  [unwired: 2 in, 2 out]
        }
        frame Enabled {
        }
      }
      n21 = invoke on="MenuRuntime" class="Clust (strict)" method="Reinit To Default"() -> ()  [unwired: 3 in, 3 out]
      n22 = property on="IO Conf view" class="Enum (strict)"("Val(Sgnl)"=enum16{"Show All", "Search"}."Show All" ("Value (Signaling)")) -> ()  [unwired: 2 in, 2 out]
      n23 = property on="Title Bar Visible" class="Bool (strict)"("Val(Sgnl)"=FALSE ("Value (Signaling)")) -> ()  [unwired: 2 in, 2 out]
      n24 = property on="Waveform Chart 2" class="WFChart (strict)"("History Data"=cluster{"result string":dbl, "UV Limit":dbl}[] []) -> ()  [unwired: 2 in, 2 out]
      n25 = property on="Title Bar Visible" class="Bool (strict)"("Val(Sgnl)"=TRUE ("Value (Signaling)")) -> ()  [unwired: 2 in, 2 out]
      n26 = call "reg-status.vi"("Operation(Read)"=enum.report-filter."ClearAll") -> ("Collected Reports"=w73:string)  [unwired: 9 in, 1 out]
      n27 = local write "User messages"(w73) -> ()
      n28 = call "util-path.vi"("Create Folders?(F)"=FALSE, "Selected Folder (PROCS)"=typePathSelector."DIR_INI" ("Selected Folder (PROCEDURE_DIR)")) -> ("error out"=w59:errorcluster, "SelectedPath"=w61:path)  [unwired: 5 in, 3 out]
      n29 = call "util-ini-key.vi"("key"=ini-key."INI.ENV" ("input 1")) -> ("key"=w65:string, "section"=w66:string)  [unwired: 9 in]
      n30 = call <vilib>:"Open Config Data.vi"("error in (no error)"=w59, "configuration file path"=w61) -> ("error out"=w60:errorcluster, "refnum"=w62:T63)  [unwired: 7 in, 1 out]
      n31 = call-poly <vilib>:"Read Key.vi"("section"=w66, "error in (no error)"=w60, "key"=w65, "refnum"=w62) -> ("error out"=w63:errorcluster, "value"=w57:string, "found?"=w56:bool, "refnum out"=w64:T63)  [unwired: 4 in]
      n32 = Get Date/Time In Seconds() -> (seconds since 1Jan1904=→"App Started at":timestamp)
      n33 = call "reg-eng-calls.vi"("Operation(Read)"=enum.report-filter."ClearAll") -> ("Collected Reports"=w71:string)  [unwired: 9 in, 1 out]
      n34 = local write "Collected Reports"(w71) -> ()
      n35 = property on="Admin Panel" class="Bool (strict)"("Val(Sgnl)"=FALSE ("Value (Signaling)")) -> ()  [unwired: 2 in, 2 out]
      n36 = property on="MAIN" class="Bool (strict)"("Val(Sgnl)"=TRUE ("Value (Signaling)")) -> ()  [unwired: 2 in, 2 out]
      n37 = call <vilib>:"Close Config Data.vi"("error in (no error)"=w63, "refnum"=w64) -> ("error out"=w51:errorcluster)  [unwired: 8 in, 1 out]
      n38 = control-ref of="This VI"() -> (w46:refnum<vi>)
      n39 = control-ref of="This VI"() -> (w75:refnum<vi>)
      n40 = Scan From String(input string=w57, error in=w51, default 1=typeEnv."ENV.PRODUCTION" ("ENV in")) -> (error out=w55:errorcluster, output 1=w53:T1)  [unwired: 2 in, 2 out]
      n41 = Compound Arithmetic op=OR(invert w55, w56) -> (w54:bool)
      n42 = call "util.fixViPanes.vi"("VI in"=w75) -> ()  [unwired: 11 in]
      n43 = property on="Splitter" class="Splitter"("Locked"=TRUE ("Splitter Position Locked")) -> ()  [unwired: 2 in, 2 out]
      n44 = Select(t=w53, s=w54, f=typeEnv."ENV.PRODUCTION") -> (s? t:f=w50:T1)
      n45 = property class="VI"(reference=w46, "Front Panel.TitleBarVis"=FALSE ("Front Panel Window:Title Bar Visible"), "FP.State"=T57."Maximized" ("Front Panel Window:State")) -> (error out=w37:errorcluster)  [unwired: 1 in, 1 out]
      n46 = call "util.environment.vi"("Operation (Get)"=enum16{"get", "set"}."set", "ENV in"=w50) -> ()  [unwired: 8 in, 2 out]
      n47 = local write "ENV"(w50) -> ()
    }
  }
  n48 = stacked-sequence {
    tunnel: [w97 _] -> w18
    frame #0 {
      # "Init Simulators List"
      n49 = property on="Simulators" class="Arr (strict)"() -> ("Value"=w96:cluster{"Input ":string, "Value":string}[])  [unwired: 2 in, 2 out]
      n50 = for {
        tunnel: w96 -> [w101] mode=indexing
        tunnel: [w101] -> w95 mode=indexing if=w98
        n51 = Unbundle By Name(w101) -> ("Input"=w100:string)
        n52 = Empty String/Path?(string/path=w100) -> (empty?=w99:bool)
        n53 = Not(x=w99) -> (.not. x?=w98:bool)
      }
      n54 = property on="Simulators" class="Arr (strict)"("Val(Sgnl)"=w95) -> (error out=w97:errorcluster)  [unwired: 2 in, 1 out]
    }
    frame #1 {
    }
  }
  n55 = Obtain Queue(max queue size (-1, unlimited)=1000000, name (unnamed)="ENG", element data type=cluster{"case":T5, "data":variant} {"case"=enum."ENG.NO-OP", "data"=variant} ("procQ"), error in (no error)=w7) -> (queue out=w32:refnum<queue>, error out=w36:errorcluster)  [unwired: 1 in, 1 out]
  n56 = global write "globals-engine.vi" "Q-Eng"(w32) -> ()
  n57 = for {
    tunnel: cluster{"cmd":T5, "data":variant}[] [{"cmd"=enum."ENG.STOP", "data"=variant}, {"cmd"=enum."ENG.INIT", "data"=variant}, {"cmd"=enum."ENG.IO.LOAD", "data"=variant}, {"cmd"=enum."ENG.LOAD", "data"=variant}, {"cmd"=enum."ENG.STATUS", "data"=variant}, {"cmd"=enum."ENG.START", "data"=variant}] ("typedefElement") -> [w102] mode=indexing
    shift-right: [w103] -> w2
    shift-left: w36 -> [w105]
    shift-right: [w104] -> w20
    shift-left: w32 -> [w106]
    n58 = Enqueue Element(queue=w106, element=w102, error in (no error)=w105) -> (queue out=w104:refnum<queue>, error out=w103:errorcluster)  [unwired: 1 in, 1 out]
  }
  n59 = flat-sequence {
    tunnel: [w110] -> _
    tunnel: [w109] -> w25
    frame #0 {
    }
    frame #1 {
      n60 = property on="lastDays" class="DigNum (strict)"("Val(Sgnl)"=7.0 ("Value (Signaling)")) -> ()  [unwired: 2 in, 2 out]
      n61 = property on="NTR Flowchart" class="Clust (strict)"() -> ("Controls[]"=w108:refnum<vi>[])  [unwired: 2 in, 2 out]
      n62 = control-ref of="ntr.status-table"() -> (w111:refnum<vi>)
      n63 = call "ntr.flow-panel.init.vi"("Controls in"=w108) -> ()  [unwired: 8 in, 3 out]
      n64 = call "ntr.status-table-init.vi"("Table in"=w111) -> ("error out"=w110:errorcluster, "Table out"=w109:refnum<vi>)  [unwired: 9 in]
    }
  }
  n65 = stacked-sequence {
    tunnel: [w113] -> w1
    tunnel: w2 -> [w114]
    frame #0 {
      n66 = global read "globals-engine.vi" "NutritionConfiguration"() -> (w115:T64[])
      n67 = call "ntr-init-io.vi"("NutritionConfiguration"=w115) -> ("error out"=w112:errorcluster)  [unwired: 10 in]
      n68 = Merge Errors(w114, w112) -> (w113:errorcluster)
    }
  }
  n69 = Obtain Queue(max queue size (-1, unlimited)=1000000, name (unnamed)="LOG", element data type=cluster{"data":variant, "Enum":T56} {"data"=variant, "Enum"=enum."LOG.NO_OP"} ("procQ"), error in (no error)=w1) -> (queue out=w21:refnum<queue>, error out=w24:errorcluster)  [unwired: 1 in, 1 out]
  n70 = global write "globals-engine.vi" "Q-Log"(w21) -> ()
  n71 = Obtain Queue(max queue size (-1, unlimited)=1000000, name (unnamed)="COM", element data type=cluster{"data":variant, "Enum":T54} {"data"=variant, "Enum"=enum."REC.NO_OP"} ("procQ")) -> (queue out=w8:refnum<queue>, error out=w14:errorcluster)  [unwired: 2 in, 1 out]
  n72 = for {
    tunnel: cluster{"data":variant, "Enum":T54}[] [{"data"=variant, "Enum"=enum."REC.OPEN-FILE"}] ("procQ") -> [w120] mode=indexing
    shift-right: [w118] -> w10
    shift-left: w8 -> [w119]
    shift-right: [w117] -> w9
    shift-left: w14 -> [w116]
    n73 = Enqueue Element(queue=w119, element=w120, error in (no error)=w116) -> (queue out=w118:refnum<queue>, error out=w117:errorcluster)  [unwired: 1 in, 1 out]
  }
  n74 = global write "globals-engine.vi" "Q-Com"(w8) -> ()
  n75 = stacked-sequence {
    tunnel: w20 -> [_ w123]
    tunnel: w1 -> [_ _]
    tunnel: w18 -> [_ _]
    frame #0 {
      n76 = To Time Stamp(1:0) -> (0:w121:timestamp)
      n77 = property on="start" class="AbsTime (strict)"("Value"=w121) -> ()  [unwired: 2 in, 2 out]
    }
    frame #1 {
      n78 = while {
        tunnel: w123 -> [w131]
        i -> [w128]
        stop <- w129 stop-if-true
        w127 = T74 2 items=["no dialog", "OK message", "continue or stop message", "OK message + warnings", "continue/stop + warnings"] ("type of dialog (OK msg:1)")
        n79 = local read "EVENT ms"() -> (w125:i32)
        n80 = Get Date/Time In Seconds() -> (seconds since 1Jan1904=w124:timestamp)
        n81 = event shown="[38] \"UiProjectSettings\", \"projectName\": Value Change" {
          selector: _ -> [_ _ _ _ _ _ _ _ _ _ _ _ _ _ _ _ _ _ _ _ _ _ _ _ _ _ _ _ _ _ _ _ _ _ _ _ _ _ _ _ _ _ _ _ _ _ _ _ _ _ _ _ _ _ _ _ _ _ _ _]
          dyn-events: _ -> [_ _ _ _ _ _ _ _ _ _ _ _ _ _ _ _ _ _ _ _ _ _ _ _ _ _ _ _ _ _ _ _ _ _ _ _ _ _ _ _ _ _ _ _ _ _ _ _ _ _ _ _ _ _ _ _ _ _ _ _]
          timeout: w125 -> [_ _ _ _ _ _ _ _ _ _ _ _ _ _ _ _ _ _ _ _ _ _ _ _ _ _ _ _ _ _ _ _ _ _ _ _ _ _ _ _ _ _ _ _ _ _ _ _ _ _ _ _ _ _ _ _ _ _ _ _]
          tunnel: w131 -> [_ _ _ _ _ _ _ _ _ _ _ _ _ _ w286 _ _ w309 _ _ _ _ _ _ _ _ _ w536 _ _ _ _ _ _ _ _ _ _ _ _ _ _ _ _ _ _ _ _ _ _ _ w1170 _ _ _ _ _ _ _ _]
          tunnel: [_ _ w147 _ w173 w177 w206 _ _ _ _ _ w263 w273 w278 _ w294 w308 w328 _ _ _ _ _ _ _ w431 _ w540 _ w567 _ _ _ w577 w663 w708 w726 w734 _ _ w936 _ _ w947 _ w990 w1036 _ _ w1147 w1169 w1319 w1404 w1411 w1414 w1417 w1420 w1423 w1426] -> w130
          tunnel: [_ _ _ _ _ _ _ _ _ _ _ _ _ _ _ _ _ _ _ _ _ _ _ _ _ _ _ w539 _ _ _ _ _ _ _ _ _ _ _ _ _ _ _ _ _ _ _ _ _ _ _ _ _ _ _ _ _ _ _ _] -> w129
          tunnel: [_ _ _ _ _ _ _ _ _ _ _ _ _ _ _ _ w297 _ _ _ _ _ _ _ _ _ _ _ _ _ _ _ _ _ _ _ _ _ _ _ _ _ _ _ _ _ _ _ _ _ _ _ _ _ _ _ _ _ _ _] -> w126
          tunnel: w124 -> [_ _ _ _ _ _ _ _ _ _ _ _ _ _ _ _ _ _ _ _ _ _ _ _ _ _ _ _ _ _ _ _ _ _ _ _ w706 _ _ _ _ _ _ _ _ _ _ _ _ _ _ _ w1318 _ _ _ _ _ _ _]
          event "Admin Panel": Value Change {
            n82 = event-data() -> ("NewVal"=w140:bool)  [unwired: 1 in]
            n83 = Select(t=310 ("Splitter Position"), s=w140, f=52 ("Splitter Position")) -> (s? t:f=w141:i32)
            n84 = property on="Splitter" class="Splitter"("Position"=w141) -> ()  [unwired: 2 in, 2 out]
            n85 = Select(t=T65."Always On" ("Vertical Scrollbar Visibility"), s="Admin Panel", f=T65."Always Off" ("Vertical Scrollbar Visibility")) -> (s? t:f=w135:T65)
            n86 = property on="VISA Report En" class="Bool (strict)"("Value"="Admin Panel") -> ()  [unwired: 2 in, 2 out]
            n87 = property on="Pane 2" class="Pane"("VertScrollbarVisibility"=w135) -> ()  [unwired: 2 in, 2 out]
            n88 = property on="Pane 2" class="Pane"("Origin"=T66 {"Horizontal"=0, "Vertical"=0}) -> ()  [unwired: 2 in, 2 out]
          }
          event "Button": Value Change {
            n89 = event-data() -> ()  [unwired: 1 in, 1 out]
            n90 = local write "Tab Control 3"(T28."UV" ("Tab Control 3")) -> ()
            n91 = local write "Tab Auxi"(enum32{"Nursery", "Windows", "Auxiliary"}."Nursery" ("Tab Auxi")) -> ()
            n92 = local write "Tab NTR"(T67."Nursery Status" ("Tab NTR")) -> ()
          }
          event "Clear Virtuals": Value Change {
            n93 = event-data() -> ()  [unwired: 1 in, 1 out]
            n94 = disable-structure shown="Enabled" {
              disable-tunnel: [w148 _] -> w147
              frame Enabled {
                n95 = call "variantCtrlIo.vi"("menu (Get Param)"=enumVarCtrlIO."IO List Configs") -> ("IO Configs List"=w150:T42[])  [unwired: 6 in, 4 out]
                n96 = call "util-io-filter.vi"("IO Search Conf"=T69 {"Device"=-1, "Label"="", "Type"=enum."VL", "Mode"=enum."Mode", "Tags"=""} ("IO Search Conf 2"), "IO Configs List"=w150) -> ("Search Results"=w149:T42[])  [unwired: 9 in]
                n97 = for {
                  tunnel: w149 -> [w156] mode=indexing
                  tunnel: [w153] -> w148
                  n98 = Bundle By Name(cluster=w156, "Value"="") -> (w155:T42)
                  n99 = call "variantCtrlIo.vi"("menu (Get Param)"=enumVarCtrlIO."IO Modify Value By Key", "IOnode in"=w155) -> ("error out"=w153:errorcluster)  [unwired: 5 in, 4 out]
                }
              }
              frame Disabled {
              }
            }
          }
          event "Cluster.MAIN", "Cluster.I/O", "Cluster.ADMIN": Value Change {
            n100 = event-data() -> ("CtlRef"=w160:refnum<vi>)  [unwired: 1 in]
            n101 = property class="Bool (strict)"(reference=w160) -> ("Label.Text"=w158:string)  [unwired: 1 in, 2 out]
            n102 = property on="Tab Main" class="TabCtl (strict)"() -> ("Pages"=w162:refnum<vi>[])  [unwired: 2 in, 2 out]
            n103 = property on="Cluster" class="Clust (strict)"() -> ("Controls[]"=w159:refnum<vi>[])  [unwired: 2 in, 2 out]
            n104 = for {
              tunnel: w162 -> [w172] mode=indexing
              tunnel: w158 -> [w170]
              tunnel: [w169] -> w161 if=w168
              i -> [w169]
              n105 = property class="Page"(reference=w172) -> ("PageLabel"=w171:string)  [unwired: 1 in, 2 out]
              n106 = Equal?(x=w171, y=w170) -> (x = y?=w168:bool)
            }
            n107 = for {
              tunnel: w159 -> [w167] mode=indexing
              tunnel: w158 -> [w165]
              n108 = property class="Ctl"(reference=w167) -> (reference out=w164:refnum<vi>, "Label.Text"=w166:string)  [unwired: 1 in, 1 out]
              n109 = Equal?(x=w166, y=w165) -> (x = y?=w163:bool)
              n110 = property class="Ctl"(reference=w164, "Value"=w163) -> ()  [unwired: 1 in, 2 out]
            }
            n111 = local write "Tab Main"(w161) -> ()
          }
          event "COM": Value Change {
            n112 = event-data() -> ()  [unwired: 1 in, 1 out]
            n113 = global read "globals-engine.vi" "Q-Com"() -> (w175:refnum<queue>)
            n114 = Enqueue Element At Opposite End(queue=w175, element=cluster{"data":variant, "Enum":T54} {"data"=variant, "Enum"=enum."REC.FETCH"}) -> (error out=w173:errorcluster)  [unwired: 2 in, 2 out]
          }
          event "DO Set by Addr.Send": Value Change {
            (unwired) TRUE ("Timer Enable")
            n115 = event-data() -> ()  [unwired: 1 in, 6 out]
            n116 = property on="Send" class="Bool (strict)"("Value"=FALSE ("State")) -> ()  [unwired: 2 in, 2 out]
            n117 = Unbundle By Name("DO Set by Addr") -> ("State"=w185:bool, "ADDR"=w180:T8, "Timeout [s]"=w184:u8)
            n118 = Bundle By Name(cluster=cluster{"State":bool, "ADDR":T8, "Timeout":u8} {"State"=FALSE, "ADDR"=8, "Timeout"=8} ("digitalPort"), "State"=w185, "ADDR"=w180, "Timeout"=w184) -> (w183:cluster{"State":bool, "ADDR":T8, "Timeout":u8})
            n119 = global read "globals-engine.vi" "Q-Eng"() -> (w176:refnum<queue>)
            n120 = Bundle By Name(cluster=cluster{"case":T5, "data":variant} {"case"=enum."ENG.RIO.DOUT-BY-ADDR", "data"=variant} ("element"), "data"=w183) -> (w187:cluster{"case":T5, "data":variant})
            n121 = Enqueue Element At Opposite End(queue=w176, element=w187) -> (queue out=w179:refnum<queue>, error out=w178:errorcluster)  [unwired: 2 in, 1 out]
            n122 = disable-structure shown="Enabled" {
              disable-tunnel: w180 -> [w194 w197 _]
              disable-tunnel: w179 -> [w191 _ _]
              disable-tunnel: w178 -> [w190 w200 w201]
              disable-tunnel: [w189 w200 w201] -> w177
              frame Disabled {
                n123 = call "util-address-parser.vi"("ADDR 2"=w194) -> ("Address"=w193:u8)  [unwired: 9 in, 1 out]
                n124 = Build Array(w193) -> (w192:u8[])
                n125 = Bundle By Name(cluster=cluster{"case":T5, "data":variant} {"case"=enum."ENG.RIO.SNAPSHOT", "data"=variant} ("element"), "data"=w192) -> (w196:cluster{"case":T5, "data":variant})
                n126 = Enqueue Element(queue=w191, element=w196, error in (no error)=w190) -> (error out=w189:errorcluster)  [unwired: 1 in, 2 out]
              }
              frame Disabled {
                n127 = call "util-address-parser.vi"("ADDR 2"=w197) -> ("Address"=w198:u8)  [unwired: 9 in, 1 out]
                n128 = Format Into String(format string="Event Set DO by address %02d", w198) -> ()  [unwired: 2 in, 2 out]
              }
              frame Enabled {
              }
            }
          }
          event "DO Set by Name.Send": Value Change {
            (unwired) TRUE ("Timer Enable")
            n129 = event-data() -> ()  [unwired: 1 in, 2 out]
            n130 = property on="Send" class="Bool (strict)"("Value"=FALSE ("State")) -> ()  [unwired: 2 in, 2 out]
            n131 = Unbundle By Name("DO Set by Name") -> ("State"=w213:bool, "Name"=w205:string, "Timeout [s]"=w212:u8)
            n132 = Bundle By Name(cluster=T70 {"State"=FALSE, "Timeout"=0, "Name"=""} ("Cluster"), "State"=w213, "Name"=w205, "Timeout"=w212) -> (w211:T70)
            n133 = call "variantCtrlIo.vi"("menu (Get Param)"=enumVarCtrlIO."IO Get By Key", "Key (use IOnode Label if empty )"=w205) -> ("IOnode out"=w204:T42)  [unwired: 5 in, 4 out]
            n134 = Unbundle By Name(w204) -> ("ADDR"=w202:T8)
            n135 = global read "globals-engine.vi" "Q-Eng"() -> (w209:refnum<queue>)
            n136 = Bundle By Name(cluster=cluster{"case":T5, "data":variant} {"case"=enum."ENG.RIO.DOUT-BY-NAME", "data"=variant} ("element"), "data"=w211) -> (w216:cluster{"case":T5, "data":variant})
            n137 = Enqueue Element At Opposite End(queue=w209, element=w216) -> (queue out=w208:refnum<queue>, error out=w207:errorcluster)  [unwired: 2 in, 1 out]
            n138 = disable-structure shown="Enabled" {
              disable-tunnel: w208 -> [w222 _]
              disable-tunnel: w207 -> [w221 w227]
              disable-tunnel: [w220 w227] -> w206
              disable-tunnel: _ -> [w219 _]
              disable-tunnel: w202 -> [w218 _]
              frame Disabled {
                n139 = call "util-address-parser.vi"("ADDR 2"=w218) -> ("Address"=w224:u8)  [unwired: 9 in, 1 out]
                n140 = Build Array(w224) -> (w223:u8[])
                n141 = Bundle By Name(cluster=cluster{"case":T5, "data":variant} {"case"=enum."ENG.RIO.SNAPSHOT", "data"=variant} ("element"), "data"=w223) -> (w226:cluster{"case":T5, "data":variant})
                n142 = Enqueue Element(queue=w222, element=w226, error in (no error)=w221) -> (error out=w220:errorcluster)  [unwired: 1 in, 2 out]
              }
              frame Enabled {
              }
            }
          }
          event "ENG ms ctrl": Value Change {
            n143 = event-data() -> ()  [unwired: 1 in, 1 out]
          }
          event Value Change {
            n144 = event-data() -> ("NewVal"=w228:T1)  [unwired: 1 in]
            n145 = call "util.environment.vi"("Operation (Get)"=enum16{"get", "set"}."set" ("Operation"), "ENV in"=w228) -> ("error out"=w232:errorcluster)  [unwired: 8 in, 1 out]
            n146 = disable-structure shown="Disabled" {
              disable-tunnel: w228 -> [w247 _]
              frame Disabled {
                # "display tab pages if debugging"
                n147 = Not Equal?(x=typeEnv."ENV.PRODUCTION", y=w247) -> (x != y?=w245:bool)
                n148 = property on="Tab Main" class="TabCtl (strict)"("Tabs Visible?"=w245) -> ()  [unwired: 2 in, 2 out]
              }
              frame Enabled {
              }
            }
            n149 = Format Into String(w228) -> (resulting string=w233:string)  [unwired: 3 in, 1 out]
            n150 = call "util-ini-key.vi"("key"=ini-key."INI.ENV" ("input 1")) -> ("key"=w229:string, "section"=w230:string)  [unwired: 9 in]
            n151 = call "util-path.vi"("Create Folders?(F)"=FALSE, "error in"=w232, "Selected Folder (PROCS)"=typePathSelector."DIR_INI" ("Selected Folder (PROCEDURE_DIR)")) -> ("error out"=w242:errorcluster, "SelectedPath"=w240:path)  [unwired: 4 in, 3 out]
            n152 = call <vilib>:"Open Config Data.vi"("error in (no error)"=w242, "configuration file path"=w240) -> ("error out"=w241:errorcluster, "refnum"=w239:T63)  [unwired: 7 in, 1 out]
            n153 = call-poly <vilib>:"Write Key.vi"("write raw string? (F)"=TRUE, "section"=w230, "error in (no error)"=w241, "value"=w233, "key"=w229, "refnum"=w239) -> ("error out"=w238:errorcluster, "refnum out"=w237:T63)  [unwired: 3 in, 1 out]
            n154 = call <vilib>:"Close Config Data.vi"("error in (no error)"=w238, "refnum"=w237) -> ("error out"=→"error out":errorcluster)  [unwired: 8 in, 1 out]
          }
          event "EVENT ms": Value Change {
            n155 = event-data() -> ()  [unwired: 1 in, 1 out]
          }
          event "File path": Value Change {
            n156 = event-data() -> ("NewVal"=w248:path)  [unwired: 1 in]
            n157 = call "util.file.vars.file-operations.vi"("selected path"=w248) -> ("error out"=w252:errorcluster, "Procedure"=w251:variant[])  [unwired: 8 in, 1 out]
            n158 = call "build.proc.parse.vi"("error"=w252, "Array in"=w251) -> ("Flow Steps"=w249:T49[], "Proc Head"=w250:T48)  [unwired: 7 in, 1 out]
            n159 = local write "UiBuildSteps"(w249) -> ()
            n160 = local write "UiBuildProcHead"(w250) -> ()
          }
          event "filter": Value Change {
            n161 = event-data() -> ()  [unwired: 1 in, 1 out]
            n162 = local read "Serial Record(s)"() -> (w256:T53[])
            n163 = call "helper-serial-log-to-string-2.vi"("filter"="filter", "Array in"=w256) -> ("Array out"=w253:T51[])  [unwired: 9 in]
            "COM Snapshot" <- w253
            n164 = Array Size(array=w253) -> (size(s)=→"Serial Log Size":i32)
            n165 = local write "COM Snapshot"(w253) -> ()
          }
          event "IO Add New": Value Change {
            n166 = event-data() -> ()  [unwired: 1 in, 1 out]
            n167 = Bundle By Name(cluster="New Element", "Mode"=enum.io.mode."RIO") -> (w259:T42)
            n168 = call "variantCtrlIo.vi"("menu (Get Param)"=enumVarCtrlIO."IO Add By Key", "IOnode in"=w259) -> ("error out"=w258:errorcluster)  [unwired: 5 in, 4 out]
            n169 = local write "New Element"(T42 {"ADDR"=0, "Label"="", "Type"=enum."Type", "Mode"=enum."RIO", "Value"="", "Tags"="", "calibration"=[]} ("New Element")) -> ()
            n170 = global read "globals-engine.vi" "Q-Log"() -> (w264:refnum<queue>)
            n171 = Enqueue Element(queue=w264, element=cluster{"data":variant, "Enum":T56} {"data"=variant, "Enum"=enum."LOG.UPDATE.SELECTORS"}, error in (no error)=w258) -> (error out=w263:errorcluster)  [unwired: 1 in, 2 out]
          }
          event "IO calib save": Value Change {
            n172 = event-data() -> ()  [unwired: 1 in, 1 out]
            n173 = local read "IO calib select"() -> (w275:string)
            n174 = call "variantCtrlIo.vi"("menu (Get Param)"=enumVarCtrlIO."IO Get By Key", "Key (use IOnode Label if empty )"=w275) -> ("error out"=w267:errorcluster, "IOnode out"=w274:T42)  [unwired: 5 in, 3 out]
            n175 = local write "IO calib save"(FALSE ("calib save")) -> ()
            n176 = in-place {
              n177 = in-place-cluster #1(w274) -> ()  [unwired: 1 out]
              n178 = in-place-cluster #1("calibration"="XyPairs") -> (w270:T42)
            }
            n179 = global read "globals-engine.vi" "Q-Eng"() -> (w266:refnum<queue>)
            n180 = call "variantCtrlIo.vi"("menu (Get Param)"=enumVarCtrlIO."IO Modify Calib By Key", "error in"=w267, "IOnode in"=w270) -> ("error out"=w268:errorcluster)  [unwired: 4 in, 4 out]
            n181 = Enqueue Element(queue=w266, element=cluster{"cmd":T5, "data":variant} {"cmd"=enum."ENG.IO.SAVE", "data"=variant} ("typedefElement"), error in (no error)=w268) -> (error out=w273:errorcluster)  [unwired: 1 in, 2 out]
          }
          event "IO calib select": Value Change {
            n182 = event-data() -> ("NewVal"=w282:string)  [unwired: 1 in]
            n183 = call "variantCtrlIo.vi"("menu (Get Param)"=enumVarCtrlIO."IO Get By Key", "Key (use IOnode Label if empty )"=w282) -> ("error out"=w279:errorcluster, "IOnode out"=w281:T42)  [unwired: 5 in, 3 out]
            n184 = property on="Chart" class="WFChart (strict)"("History Data"=cluster{"X":dbl, "Y":dbl}[] []) -> ()  [unwired: 2 in, 2 out]
            n185 = Unbundle By Name(w281) -> ("calibration"=w280:T43[])
            n186 = local write "XyPairs"(w280) -> ()
            n187 = Enqueue Element(queue=w286, element=cluster{"cmd":T5, "data":variant} {"cmd"=enum."ENG.RIO.AIN-SNAPSHOT-CALIB", "data"=variant} ("typedefElement"), error in (no error)=w279) -> (error out=w285:errorcluster)  [unwired: 1 in, 2 out]
            n188 = call <vilib>:"Clear Errors.vi"("error in (no error)"=w285) -> ("error out"=w278:errorcluster)  [unwired: 5 in, 1 out]
          }
          event "IO Conf view": Value Change {
            n189 = event-data() -> ("NewVal"=w290:enum16{"Show All", "Search"})  [unwired: 1 in]
            n190 = case shown="\"Show All\"" w290 {
              tunnel: [T71."Disabled and Grayed Out" ("Disabled") T71."Enabled" ("Disabled")] -> w289
              frame "Show All" {
              }
              frame "Search" {
              }
            }
            n191 = property on="IO Search Conf" class="Clust (strict)"("DisabledEnum"=w289, "Value"=T45 {"ADDR"=-1, "Label"="", "Type"=enum."Type", "Mode"=enum."Mode", "Tags"=""} ("IO Search Conf")) -> ()  [unwired: 2 in, 2 out]
          }
          event "IO Conf": Value Change {
            # "IO Conf not allows adding (or removing) elements using right-click menu. new elements added by seperate ui object and the IO conf only allow to edit elements and delete by renaming to empty name"
            n192 = event-data() -> ("OldVal"=w301:T46, "NewVal"=w300:T46)  [unwired: 1 in]
            n193 = call "helper-io-edit.vi"("NewVal"=w300, "OldVal"=w301) -> ("error out"=w295:errorcluster, "IO changed?"=w296:bool)  [unwired: 7 in, 1 out]
            n194 = Select(t="Edit I/O Configuration" ("string"), s=w296, f="") -> (s? t:f=w297:string)
            n195 = case shown="True" w296 {
              tunnel: w295 -> [w302 w304]
              tunnel: [w302 w303] -> w294
              frame False {
              }
              frame True {
                n196 = global read "globals-engine.vi" "Q-Eng"() -> (w306:refnum<queue>)
                n197 = Enqueue Element(queue=w306, element=cluster{"cmd":T5, "data":variant} {"cmd"=enum."ENG.STATUS", "data"=variant} ("typedefElement"), error in (no error)=w304) -> (error out=w303:errorcluster)  [unwired: 1 in, 2 out]
              }
            }
            n198 = local read "IO Search Conf"() -> (w293:T45)
            n199 = property on="IO Search Conf" class="Clust (strict)"("Val(Sgnl)"=w293) -> ()  [unwired: 2 in, 2 out]
          }
          event "IO List.save", "IO List.loadCsv": Value Change {
            n200 = event-data() -> ("CtlRef"=w311:refnum<vi>)  [unwired: 1 in]
            n201 = property class="Bool (strict)"(reference=w311) -> ("Label.Text"=w310:string)  [unwired: 1 in, 2 out]
            n202 = local write "IO List"(cluster{"save":bool, "loadCsv":bool} {"save"=FALSE, "loadCsv"=FALSE} ("StorageMenu")) -> ()
            n203 = case shown="\"save\"" w310 {
              tunnel: [w313 w319 errorcluster {"status"=TRUE, "code"=-564498, "source"="Case Error for UiMenuIoBuilder"} ("error out")] -> w308
              tunnel: w309 -> [w314 w316 _]
              frame "save" {
                # "save to IO directory"
                n204 = Enqueue Element At Opposite End(queue=w314, element=cluster{"cmd":T5, "data":variant} {"cmd"=enum."ENG.IO.SAVE", "data"=variant} ("typedefElement")) -> (error out=w313:errorcluster)  [unwired: 2 in, 2 out]
              }
              frame "loadCsv" {
                n205 = call "util-io-csv-load.vi"("file path (dialog if empty)"=path "") -> ("error out"=w317:errorcluster, "Array"=w318:T42[])  [unwired: 9 in]
                n206 = case shown="No Error" w317 {
                  selector: w317 -> [_ w326]
                  tunnel: [w325 w326] -> w319
                  tunnel: w318 -> [w320 _]
                  tunnel: w316 -> [w324 _]
                  frame No Error {
                    n207 = Bundle By Name(cluster=cluster{"cmd":T5, "data":variant} {"cmd"=enum."ENG.IO.LOAD", "data"=variant} ("typedefElement"), "data"=w320, "cmd"=state-engine."ENG.IO.LOAD") -> (w322:cluster{"cmd":T5, "data":variant})
                    n208 = Enqueue Element(queue=w324, element=w322) -> (error out=w325:errorcluster)  [unwired: 2 in, 2 out]
                  }
                  frame Error {
                  }
                }
              }
              frame Default {
              }
            }
          }
          event "IO Map DO": Value Change {
            n209 = event-data() -> ("OldVal"=w330:T37[], "NewVal"=w336:T37[])  [unwired: 1 in]
            n210 = Not Equal?(x=w330, y=w336) -> (x != y?=w338:T75)
            n211 = Array Max & Min(array=w338) -> (max index (indices)=w331:i32)  [unwired: 3 out]
            n212 = Index Array(array=w338, index=w331) -> (element=w337:T76)
            n213 = Index Array(array=w336, index=w331) -> (element=w335:T37)
            n214 = Unbundle By Name(w335) -> ("ADDR"=w329:T8, "Label"=w334:string, "State"=w333:bool)
            n215 = Unbundle By Name(w337) -> ("State"=w332:bool)
            n216 = case shown="True" w332 {
              tunnel: w334 -> [_ w340]
              tunnel: w333 -> [_ w344]
              tunnel: w329 -> [_ w343]
              tunnel: [_ w339] -> w328
              frame False {
              }
              frame True {
                n217 = property on="Timeout [s]" class="DigNum (strict)"() -> ("Value"=w341:u8)  [unwired: 2 in, 2 out]
                n218 = call "helper-do-active-verif.vi"("name"=w340, "Value"=w341, "State"=w344, "ADDR"=w343) -> ("digitalPort"=w345:cluster{"State":bool, "ADDR":T8, "Timeout":u8}, "T button?"=w342:bool)  [unwired: 6 in]
                n219 = case shown="True" w342 {
                  tunnel: w345 -> [w349 _]
                  tunnel: [w346 _] -> w339
                  frame True {
                    w348 = cluster{"cmd":T5, "data":variant} {"cmd"=enum."ENG.RIO.SNAPSHOT", "data"=variant}  # snapshot all
                    n220 = global read "globals-engine.vi" "Q-Eng"() -> (w351:refnum<queue>)
                    n221 = Bundle By Name(cluster=cluster{"case":T5, "data":variant} {"case"=enum."ENG.RIO.DOUT-BY-ADDR", "data"=variant} ("element"), "data"=w349) -> (w352:cluster{"case":T5, "data":variant})
                    n222 = Enqueue Element At Opposite End(queue=w351, element=w352) -> (queue out=w347:refnum<queue>)  [unwired: 2 in, 2 out]
                    n223 = Enqueue Element(queue=w347, element=w348) -> (error out=w346:errorcluster)  [unwired: 2 in, 2 out]
                  }
                  frame False {
                    w354 = cluster{"cmd":T5, "data":variant} {"cmd"=enum."ENG.RIO.SNAPSHOT", "data"=variant}  # snapshot all
                    n224 = global read "globals-engine.vi" "Q-Eng"() -> (w353:refnum<queue>)
                    n225 = Enqueue Element(queue=w353, element=w354) -> ()  [unwired: 2 in, 3 out]
                  }
                }
              }
            }
          }
          event "IO Map Take Snapshot": Value Change {
            w355 = cluster{"cmd":T5, "data":variant} {"cmd"=enum."ENG.RIO.SNAPSHOT", "data"=variant}  # snapshot all
            n226 = event-data() -> ()  [unwired: 1 in, 1 out]
            n227 = local write "IO Map Take Snapshot"(FALSE ("IO Map Take Snapshot")) -> ()
            n228 = global read "globals-engine.vi" "Q-Eng"() -> (w357:refnum<queue>)
            n229 = property on="State" class="Bool (strict)"("DisabledEnum"=T71."Disabled" ("Disabled")) -> ()  [unwired: 2 in, 2 out]
            n230 = Enqueue Element(queue=w357, element=w355) -> ()  [unwired: 2 in, 3 out]
          }
          event "IO Search Conf": Value Change {
            n231 = event-data() -> ()  [unwired: 1 in, 6 out]
            n232 = call "variantCtrlIo.vi"("menu (Get Param)"=enumVarCtrlIO."IO List Configs") -> ("IO Configs List"=w365:T42[])  [unwired: 6 in, 4 out]
            n233 = call "util-io-filter.vi"("IO Search Conf"="IO Search Conf", "IO Configs List"=w365) -> ("Search Results"=w362:T42[])  [unwired: 9 in]
            n234 = local read "IOconf Sort"() -> (w360:T44)
            n235 = call "util-io-sort.vi"(10:w360, "IO Configs List"=w362) -> ("Result"=w361:T42[])  [unwired: 9 in]
            n236 = Array Size(array=w361) -> (size(s)=→"size":i32)
            n237 = local write "IO Conf"(w361) -> ()
          }
          event "IO Search Map Refresh": Value Change {
            n238 = event-data() -> ()  [unwired: 1 in, 1 out]
            n239 = local write "IO Search Map Refresh"(FALSE ("IO Search Refresh")) -> ()
            n240 = property on="IO Search Map" class="Clust (strict)"("Val(Sgnl)"=T41 {"By Name"="", "By Tag"="", "By Address"=-1} ("Value (Signaling)")) -> ()  [unwired: 2 in, 2 out]
          }
          event "IO Search Map": Value Change {
            n241 = event-data() -> ()  [unwired: 1 in, 1 out]
            n242 = Unbundle By Name("IO Search Map") -> ("By Address"=w375:i32, "By Name"=w385:string, "By Tag"=w384:string)
            n243 = call "variantCtrlIo.vi"("menu (Get Param)"=enumVarCtrlIO."IO List Configs") -> ("IO Configs List"=w377:T42[])  [unwired: 6 in, 4 out]
            n244 = call "util-address-range.vi"("ADDR"=w375) -> ("x .and. y?"=w370:bool)  [unwired: 10 in]
            n245 = Select(t=T71."Enabled" ("Disabled"), s=w370, f=T71."Disabled and Grayed Out" ("Disabled")) -> (s? t:f=w371:T71)
            n246 = case shown="False" w370 {
              selector: w370 -> [w408 _]
              tunnel: [w408 w409] -> w369
              frame False {
              }
              frame True {
                n247 = local read "Show Undefined"() -> (w409:bool)
              }
            }
            n248 = And(x=w370, y=w369) -> (x .and. y?=w374:bool)
            n249 = case shown="False" w374 {
              tunnel: w377 -> [w410 w413]
              tunnel: [w410 w412] -> w376
              tunnel: w375 -> [_ w411]
              frame False {
              }
              frame True {
                n250 = call "helper-snapshot-list.vi"("ADDR"=w411, "IOnodes in"=w413) -> ("IOcon snapshot list out"=w412:T42[])  [unwired: 9 in]
              }
            }
            n251 = property on="Show Undefined" class="Bool (strict)"("DisabledEnum"=w371) -> ()  [unwired: 2 in, 2 out]
            n252 = Bundle By Name(cluster=T72 {"ADDR"=0, "Label"="", "Type"=enum."Type", "Mode"=enum."Mode", "Tags"=""} ("IO Search Conf"), "ADDR"=w375, "Label"=w385, "Tags"=w384) -> (w383:T72)
            n253 = call "util-io-filter.vi"("IO Search Conf"=w383, "IO Configs List"=w376) -> ("Search Results"=w368:T42[])  [unwired: 9 in]
            n254 = call "helper-io-set-tables.vi"("IOnodes"=w368) -> ("VL"=w379:T42[], "IO Map AI"=w380:T39[], "IO Map DO"=w381:T37[], "IO Map DI"=w382:T40[])  [unwired: 7 in]
            n255 = disable-structure shown="Enabled" {
              disable-tunnel: w382 -> [w403 w407]
              disable-tunnel: w381 -> [w402 w406]
              disable-tunnel: w380 -> [w401 w405]
              disable-tunnel: w379 -> [w400 w404]
              disable-tunnel: u32[] [0] ("Index Values") -> [w399 _]
              frame Disabled {
                n256 = property on="IO Map DI" class="Arr (strict)"("Value"=w403, "Index Values"=w399) -> ()  [unwired: 2 in, 2 out]
                n257 = property on="IO Map DO" class="Arr (strict)"("Value"=w402, "Index Values"=w399) -> ()  [unwired: 2 in, 2 out]
                n258 = property on="IO Map AI" class="Arr (strict)"("Value"=w401, "Index Values"=w399) -> ()  [unwired: 2 in, 2 out]
                n259 = property on="IO Map VL" class="Arr (strict)"("Value"=w400, "Index Values"=w399) -> ()  [unwired: 2 in, 2 out]
              }
              frame Enabled {
                n260 = property on="IO Map DI" class="Arr (strict)"("Value"=w407) -> ()  [unwired: 2 in, 2 out]
                n261 = property on="IO Map DO" class="Arr (strict)"("Value"=w406) -> ()  [unwired: 2 in, 2 out]
                n262 = property on="IO Map AI" class="Arr (strict)"("Value"=w405) -> ()  [unwired: 2 in, 2 out]
                n263 = property on="IO Map VL" class="Arr (strict)"("Value"=w404) -> ()  [unwired: 2 in, 2 out]
              }
            }
            n264 = flat-sequence {
              tunnel: w382 -> [w398]
              tunnel: w381 -> [w396]
              tunnel: w380 -> [w392]
              tunnel: w379 -> [w391]
              frame #0 {
                w389 = cluster{"cmd":T5, "data":variant} {"cmd"=enum."ENG.RIO.SNAPSHOT", "data"=variant}  # snapshot all
                n265 = Array Size(array=w396) -> (size(s)=→"IO Map DO Count":i32)
                n266 = Array Size(array=w391) -> (size(s)=→"IO Map VL Count":i32)
                n267 = Array Size(array=w392) -> (size(s)=→"IO Map AI Count":i32)
                n268 = Array Size(array=w398) -> (size(s)=→"IO Map DI Count":i32)
                n269 = global read "globals-engine.vi" "Q-Eng"() -> (w390:refnum<queue>)
                n270 = Enqueue Element(queue=w390, element=w389) -> ()  [unwired: 2 in, 3 out]
              }
            }
          }
          event Value Change {
            n271 = event-data() -> ()  [unwired: 1 in, 1 out]
            n272 = local read "IO Search Conf"() -> (w414:T45)
            n273 = property on="IO Search Conf" class="Clust (strict)"("Val(Sgnl)"=w414) -> ()  [unwired: 2 in, 2 out]
          }
          event Value Change {
            n274 = event-data() -> ()  [unwired: 1 in, 1 out]
            n275 = disable-structure shown="Enabled" {
              disable-tunnel: "IRR Params" -> [w416]
              frame Enabled {
                n276 = global write "globals-engine.vi" "IRR Params"(w416) -> ()
                n277 = To Variant(anything=w416) -> (Variant=w424:variant)
                n278 = Build Array(w424) -> (w423:variant[])
                n279 = call "util.file.vars.vi"("Operation(Read)"=enum16{"Read File", "Write File"}."Write File", "Directory (DIR_PROC)"=typePathSelector."DIR_CONFIG" ("Directory (PROCEDURE_DIR)"), "Proc Name(open dialog if empty)"="IRR_CONF" ("Proc Name"), "Vars[] in"=w423) -> ("error out"=w422:errorcluster)  [unwired: 3 in, 4 out]
                n280 = case shown="No Error" w422 {
                  selector: w422 -> [_ w426]
                  tunnel: [_ w426] -> w421
                  frame No Error {
                  }
                  frame Error {
                  }
                }
                n281 = global read "globals-engine.vi" "Q-Log"() -> (w425:refnum<queue>)
                n282 = Enqueue Element(queue=w425, element=cluster{"data":variant, "Enum":T56} {"data"=variant, "Enum"=enum."LOG.UPDATE.IRR"} ("procQ"), error in (no error)=w421) -> ()  [unwired: 1 in, 3 out]
              }
            }
          }
          event "Log Clear": Value Change {
            n283 = event-data() -> ()  [unwired: 1 in, 1 out]
            n284 = call "reg-log-general.vi"("Operation(Read)"=enum.report-filter."ClearAll") -> ("compact report"=w429:T77[])  [unwired: 8 in, 2 out]
            n285 = local write "Report General"(w429) -> ()
            n286 = local write "Proc Name"("" ("Proc Name")) -> ()
          }
          event "MenuRuntime.Run", "MenuRuntime.Step", "MenuRuntime.Load", "MenuRuntime.Status", "MenuRuntime.ProcedureRun", "MenuRuntime.ProcedureStep", "MenuRuntime.ProcedureReload", "MenuRuntime.Unload", "MenuRuntime.Reload": Value Change {
            n287 = event-data() -> ("CtlRef"=w436:refnum<vi>)  [unwired: 1 in]
            n288 = property class="Bool (strict)"(reference=w436) -> (reference out=w435:refnum<vi>, "Value"=w434:bool, "Label.Text"=w432:string)  [unwired: 1 in, 1 out]
            n289 = global read "globals-engine.vi" "Q-Eng"() -> (w430:refnum<queue>)
            n290 = case shown="\"Step\"" w432 {
              tunnel: w430 -> [w439 w441 w444 w485 w496 w505 w510 _ w517 w520 w525 _]
              tunnel: w434 -> [_ _ _ _ _ w506 _ w515 _ w521 _ _]
              tunnel: [_ _ _ _ _ w506 _ w515 _ w521 _ FALSE] -> w433
              tunnel: [w438 w440 w443 w486 w497 w504 w509 w514 w516 w519 w524 errorcluster {"status"=TRUE, "code"=-1, "source"="Missing menu in UiRuntimeMenu"} ("error out")] -> w431
              frame "Init" {
                n291 = Enqueue Element(queue=w439, element=cluster{"cmd":T5, "data":variant} {"cmd"=enum."ENG.INIT", "data"=variant} ("typedefElement")) -> (error out=w438:errorcluster)  [unwired: 2 in, 2 out]
              }
              frame "InitGlobals" {
                n292 = Enqueue Element(queue=w441, element=cluster{"cmd":T5, "data":variant} {"cmd"=enum."ENG.INIT.VARS", "data"=variant} ("typedefElement")) -> (error out=w440:errorcluster)  [unwired: 2 in, 2 out]
              }
              frame "Load" {
                # "LOAD FOR PRODUCTION"
                n293 = call <vilib>:"Three Button Dialog.vi"("Right Button Text (\"Cancel\")"="All" ("Left Button Text (\"Yes\")"), "Center Button Text (\"No\")"="Folder" ("Left Button Text (\"Yes\")"), "Left Button Text (\"Yes\")"="File" ("Left Button Text (\"Yes\")"), "message"="Load ...") -> ("Which Button?"=w449:T78)  [unwired: 7 in]
                n294 = case shown="\"Left Button\"" w449 {
                  tunnel: w444 -> [_ w453 w466 w479]
                  tunnel: [_ w452 w465 w478] -> w443
                  frame "Window Close", Default {
                  }
                  frame "Left Button" {
                    w450 = 43  # canceled?
                    # "Load Single"
                    n295 = call "util.file.vars.path-parser.vi"("allowDialogs?(False)"=TRUE) -> ("error out"=w455:errorcluster, "cancelled"=w456:bool, "selected path"=w457:path)  [unwired: 8 in]
                    n296 = call <vilib>:"Clear Errors.vi"("error in (no error)"=w455, "specific error code to clear (0: all)"=w450) -> ("error out"=w451:errorcluster)  [unwired: 4 in, 1 out]
                    n297 = case shown="False" w456 {
                      tunnel: w457 -> [w463 _]
                      tunnel: w453 -> [w462 _]
                      tunnel: [w459 w464] -> w452
                      tunnel: w451 -> [w458 w464]
                      frame False {
                        n298 = Bundle By Name(cluster=cluster{"cmd":T5, "data":variant} {"cmd"=enum."ENG.LOAD.SINGLE", "data"=variant} ("typedefElement"), "data"=w463) -> (w461:cluster{"cmd":T5, "data":variant})
                        n299 = Enqueue Element(queue=w462, element=w461, error in (no error)=w458) -> (error out=w459:errorcluster)  [unwired: 1 in, 2 out]
                      }
                      frame True {
                      }
                    }
                  }
                  frame "Center Button" {
                    # "Load Module"
                    n300 = call "util.file.vars.path-parser.vi"("allowDialogs?(False)"=TRUE) -> ("error out"=w468:errorcluster, "cancelled"=w469:bool, "selected path"=w470:path)  [unwired: 8 in]
                    n301 = case shown="False" w469 {
                      tunnel: w470 -> [w476 _]
                      tunnel: w466 -> [w475 _]
                      tunnel: [w472 w477] -> w465
                      tunnel: w468 -> [w471 w477]
                      frame False {
                        n302 = Bundle By Name(cluster=cluster{"cmd":T5, "data":variant} {"cmd"=enum."ENG.LOAD.MODULE", "data"=variant} ("typedefElement"), "data"=w476) -> (w474:cluster{"cmd":T5, "data":variant})
                        n303 = Enqueue Element(queue=w475, element=w474, error in (no error)=w471) -> (error out=w472:errorcluster)  [unwired: 1 in, 2 out]
                      }
                      frame True {
                      }
                    }
                  }
                  frame "Right Button" {
                    # "Load All"
                    n304 = Enqueue Element(queue=w479, element=cluster{"cmd":T5, "data":variant} {"cmd"=enum."ENG.LOAD", "data"=variant} ("typedefElement")) -> (error out=w478:errorcluster)  [unwired: 2 in, 2 out]
                  }
                }
              }
              frame "ProcedureRun" {
                # "\"ProcedureRun\", \"Run\" \nset timeout interval to call eng execution periodically"
                n305 = property on="ProcedureSelect" class="CmbBox"() -> ("Value"=w483:string)  [unwired: 2 in, 2 out]
                n306 = Format Into String(format string="Run %s?", w483) -> (resulting string=w482:string)  [unwired: 2 in, 1 out]
                n307 = Two Button Dialog(message=w482) -> (T button?=w481:bool)  [unwired: 2 in]
                n308 = case shown="True" w481 {
                  tunnel: [_ w489] -> w486
                  tunnel: w485 -> [_ w488]
                  tunnel: w483 -> [_ w487]
                  frame False {
                  }
                  frame True {
                    n309 = Bundle By Name(cluster=cluster{"cmd":T5, "data":variant} {"cmd"=enum."ENG.PROC.START", "data"=variant} ("typedefElement"), "data"=w487) -> (w491:cluster{"cmd":T5, "data":variant})
                    n310 = Enqueue Element(queue=w488, element=w491) -> (error out=w489:errorcluster)  [unwired: 2 in, 2 out]
                  }
                }
              }
              frame "ProcedureLoad" {
                # "\"ProcedureRun\", \"Run\" \nset timeout interval to call eng execution periodically"
                n311 = property on="ProcedureSelect" class="CmbBox"() -> ("Value"=w494:string)  [unwired: 2 in, 2 out]
                n312 = Format Into String(format string="Reload %s?", w494) -> (resulting string=w493:string)  [unwired: 2 in, 1 out]
                n313 = Two Button Dialog(message=w493) -> (T button?=w492:bool)  [unwired: 2 in]
                n314 = case shown="True" w492 {
                  tunnel: [_ w500] -> w497
                  tunnel: w496 -> [_ w499]
                  tunnel: w494 -> [_ w498]
                  frame False {
                  }
                  frame True {
                    n315 = Bundle By Name(cluster=cluster{"cmd":T5, "data":variant} {"cmd"=enum."ENG.PROC.RELOAD-BY-NAME", "data"=variant} ("typedefElement"), "data"=w498) -> (w502:cluster{"cmd":T5, "data":variant})
                    n316 = Enqueue Element(queue=w499, element=w502) -> (error out=w500:errorcluster)  [unwired: 2 in, 2 out]
                  }
                }
              }
              frame "ProcedureStep" {
                n317 = property on="ProcedureSelect" class="CmbBox"() -> ("Value"=w503:string)  [unwired: 2 in, 2 out]
                n318 = call "eng-call-execute.vi"("Proc Name to Execute (empty: Execute All)"=w503, "Queue in"=w505) -> ("error out"=w504:errorcluster)  [unwired: 9 in]
              }
              frame "Reload" {
                n319 = Two Button Dialog(message="Reload All Procedures?") -> (T button?=w507:bool)  [unwired: 2 in]
                n320 = case shown="True" w507 {
                  tunnel: w510 -> [_ w513]
                  tunnel: [_ w512] -> w509
                  frame False {
                  }
                  frame True {
                    n321 = Enqueue Element(queue=w513, element=cluster{"cmd":T5, "data":variant} {"cmd"=enum."ENG.LOAD.RELOAD", "data"=variant} ("typedefElement")) -> (error out=w512:errorcluster)  [unwired: 2 in, 2 out]
                  }
                }
              }
              frame "Run" {
                # "\"ProcedureRun\", \"Run\" \nset timeout interval to call eng execution periodically"
                n322 = call "eng-call-start.vi"("Start(T)/Stop(F)"=w515) -> ("error out"=w514:errorcluster)  [unwired: 10 in]
              }
              frame "Status" {
                n323 = Enqueue Element(queue=w517, element=cluster{"cmd":T5, "data":variant} {"cmd"=enum."ENG.STATUS", "data"=variant} ("typedefElement")) -> (error out=w516:errorcluster)  [unwired: 2 in, 2 out]
              }
              frame "Step" {
                # "\"Step\" \ncall eng execution (once)"
                n324 = call "eng-call-execute.vi"("Queue in"=w520) -> ("error out"=w519:errorcluster)  [unwired: 10 in]
              }
              frame "Unload" {
                n325 = Two Button Dialog(message="Unload All Procedures?") -> (T button?=w522:bool)  [unwired: 2 in]
                n326 = case shown="True" w522 {
                  tunnel: w525 -> [_ w528]
                  tunnel: [_ w527] -> w524
                  frame False {
                  }
                  frame True {
                    n327 = for {
                      tunnel: w528 -> [w531]
                      tunnel: [w530] -> w527
                      tunnel: cluster{"cmd":T5, "data":variant}[] [{"cmd"=enum."ENG.LOAD.UNLOAD", "data"=variant}, {"cmd"=enum."ENG.STATUS", "data"=variant}] ("typedefElement") -> [w529] mode=indexing
                      n328 = Enqueue Element(queue=w531, element=w529) -> (error out=w530:errorcluster)  [unwired: 2 in, 2 out]
                    }
                  }
                }
              }
              frame Default {
              }
            }
            n329 = property class="Bool (strict)"(reference=w435, "Value"=w433) -> ()  [unwired: 1 in, 2 out]
          }
          event "MenuRuntime.Stop": Value Change {
            n330 = event-data() -> ("NewVal"=w539:bool)  [unwired: 1 in]
            n331 = Bundle By Name(cluster=cluster{"cmd":T5, "data":variant} {"cmd"=enum."ENG.EXIT", "data"=variant} ("typedefElement"), "data"=variant) -> (w537:cluster{"cmd":T5, "data":variant})
            n332 = global write "globals-engine.vi" "STOP"(TRUE ("STOP")) -> ()
            n333 = Enqueue Element At Opposite End(queue=w536, element=w537) -> ()  [unwired: 2 in, 3 out]
          }
          event "NTR Panel.CloseAll": Value Change {
            n334 = event-data() -> ("CtlRef"=w543:refnum<vi>)  [unwired: 1 in]
            n335 = property class="Bool (strict)"(reference=w543) -> ("Label.Text"=w542:string, "BoolText.Text"=w541:string)  [unwired: 1 in, 2 out]
            n336 = case shown="\"CloseAll\"" w542 {
              tunnel: w541 -> [_ w548]
              tunnel: [_ w544] -> w540
              frame "False", Default {
              }
              frame "CloseAll" {
                n337 = Concatenate Strings(w548, "?" ("string")) -> (w547:string)
                n338 = Two Button Dialog(message=w547) -> (T button?=w545:bool)  [unwired: 2 in]
                n339 = case shown="True" w545 {
                  tunnel: [_ w549] -> w544
                  frame False {
                  }
                  frame True {
                    n340 = global read "globals-engine.vi" "NutritionConfiguration"() -> (w550:T64[])
                    n341 = call "ntr-init-io.vi"("NutritionConfiguration"=w550) -> ("error out"=w549:errorcluster)  [unwired: 10 in]
                  }
                }
              }
            }
          }
          event "ntrGraphPeriod.lastDays": Value Change {
            n342 = event-data() -> ("NewVal"=w553:dbl)  [unwired: 1 in]
            n343 = Get Date/Time In Seconds() -> (seconds since 1Jan1904=w561:timestamp)
            n344 = invoke on="End" class="AbsTime (strict)" method="Reinit To Default"() -> (error out=w562:errorcluster)  [unwired: 3 in, 2 out]
            n345 = expression code="x*24*60*60"(w553) -> (w552:dbl)
            n346 = Subtract(x=w561, y=w552) -> (x-y=w554:timestamp)
            n347 = Seconds To Date/Time(time stamp (now)=w554) -> (date time rec=w558:T73)  [unwired: 1 in]
            n348 = Unbundle By Name(w558) -> ("year"=w557:i32, "month"=w556:i32, "day of month"=w555:i32)
            n349 = Bundle By Name(cluster=T73 {"fractional second"=0.0, "second"=0, "minute"=0, "hour"=0, "day of month"=0, "month"=0, "year"=0, "day of week"=0, "day of year"=0, "DST"=0} ("date time rec"), "year"=w557, "month"=w556, "day of month"=w555) -> (w559:T73)
            n350 = Date/Time To Seconds(2:w559) -> (0:w551:timestamp)  [unwired: 1 in]
            n351 = property on="Start" class="AbsTime (strict)"(error in=w562, "Val(Sgnl)"=w551) -> ()  [unwired: 1 in, 2 out]
          }
          event "ntrGraphPeriod.refresh": Value Change {
            n352 = event-data() -> ()  [unwired: 1 in, 3 out]
            n353 = property on="refresh" class="Bool (strict)"("Value"=FALSE) -> ()  [unwired: 2 in, 2 out]
            n354 = property on="ntrDosepumpSelect" class="CmbBox"() -> ("Value"=w565:string)  [unwired: 2 in, 2 out]
            n355 = property on="ntrInputSelect" class="CmbBox"() -> ("Value"=w563:string)  [unwired: 2 in, 2 out]
            n356 = call "util.ntr.dose-path.vi"("ntrGraphPeriod"="ntrGraphPeriod", "Dosepump"=w563) -> ("error out"=w567:errorcluster, "Graph"=→"Nutrition Sensor Graph":cluster{"X":dbl[], "Y":dbl[]})  [unwired: 7 in, 1 out]
            n357 = call "util.ntr.dose-path.vi"("ntrGraphPeriod"="ntrGraphPeriod", "Dosepump"=w565) -> ("Graph"=→"EC 3":cluster{"X":dbl[], "Y":dbl[]})  [unwired: 7 in, 2 out]
          }
          event "ntrInputSelect", "ntrGraphPeriod.Time range", "ntrDosepumpSelect": Value Change {
            n358 = event-data() -> ()  [unwired: 1 in, 1 out]
            n359 = property on="refresh" class="Bool (strict)"("Val(Sgnl)"=TRUE ("Value (Signaling)")) -> ()  [unwired: 2 in, 2 out]
          }
          event "PBR Builder": Value Change {
            n360 = event-data() -> ()  [unwired: 1 in, 1 out]
            n361 = property on="COMPILE" class="Bool (strict)"("Val(Sgnl)"=TRUE ("Value (Signaling)")) -> ()  [unwired: 2 in, 2 out]
          }
          event "PBR PROC": Value Change {
            n362 = event-data() -> ()  [unwired: 1 in, 1 out]
            n363 = property on="LOAD" class="Bool (strict)"("Val(Sgnl)"=TRUE ("Value (Signaling)")) -> ()  [unwired: 2 in, 2 out]
          }
          event "PBR.COMPILE", "PBR.SAVE", "PBR.LOAD", "PBR.SAVEAS": Value Change {
            # "templateSave (save as text file)\ntemplateLoad (load from text file)\nprocedureSave(build flow and save as varient file)\nprocedureLoad(load from varient file and parse to flow)"
            n364 = event-data() -> ("CtlRef"=w578:refnum<vi>)  [unwired: 1 in]
            n365 = property class="Bool (strict)"(reference=w578, "Value"=FALSE) -> ("Label.Text"=w580:string)  [unwired: 1 in, 2 out]
            n366 = local read "PBR PROC"() -> (w573:string)
            n367 = feedback #2() -> (w574:variant[])  [unwired: 1 in]
            n368 = case shown="\"SAVE\"" w580 {
              tunnel: [_ w601 w623 w642] -> w579
              tunnel: [w590 w595 w617 w637] -> w575
              tunnel: w574 -> [_ w595 w617 w636]
              tunnel: w573 -> [_ w599 _ w638]
              frame "COMPILE", Default {
                # "(2)"
                # "(1)"
                # "(1)  Build PBR_BUILDER to FLOW  \n(2)  Build FLOW to procedure (2.1) Save procedure (DIR_PROC)"
                n369 = local read "PBR Builder"() -> (w583:T23)
                n370 = call "pbr-builder.vi"("PBR FLOW in"=w583) -> ("s? t:f"=w586:errorcluster, "FLOW out"=w581:T49[])  [unwired: 8 in, 1 out]
                n371 = call "build.proc.vi"("error in"=w586, "Flow"=w581, "Proc Head"=T48 {"Procedure Name"="", "Running"=FALSE, "tags"=""}) -> ("error out"=w589:errorcluster, "Instructions"=w590:variant[])  [unwired: 7 in]
                n372 = Select(t=u32 16711680 ("Text.Text Colors:Text Color"), s=w589, f=u32 0 ("Text.Text Colors:Text Color")) -> (s? t:f=w592:u32)
                n373 = Select(t=w589, s=w589, f=errorcluster {"status"=FALSE, "code"=0, "source"="Compiled Successfully"} ("error constant")) -> (s? t:f=w587:errorcluster)
                n374 = call <vilib>:"Space Constant.vi"() -> ()  [unwired: 1 out]
                n375 = property on="source" class="Str"("Text.TextColor"=w592) -> ()  [unwired: 2 in, 2 out]
                n376 = Get Date/Time String(want seconds? (F)=TRUE) -> ()  [unwired: 2 in, 2 out]
                n377 = Unbundle By Name(w587) -> ("source"=w585:string)
                n378 = Concatenate Strings(w585) -> (→"source":string)
              }
              frame "SAVE" {
                # "(3)  Save PBR_BUILDER as CONFIG"
                n379 = Format Into String(format string="Save %s?", w599) -> (resulting string=w597:string)  [unwired: 2 in, 1 out]
                n380 = global read "globals-engine.vi" "Q-Eng"() -> (w596:refnum<queue>)
                n381 = Two Button Dialog(message=w597) -> (T button?=w600:bool)  [unwired: 2 in]
                n382 = case shown="True" w600 {
                  tunnel: [_ w607] -> w601
                  tunnel: w599 -> [_ w604]
                  tunnel: w595 -> [_ w611]
                  tunnel: w596 -> [_ w606]
                  frame False {
                  }
                  frame True {
                    n383 = call "util.file.vars.vi"("Operation(Read)"=enum16{"Read File", "Write File"}."Write File", "Proc Name(open dialog if empty)"=w604, "Vars[] in"=w611) -> ("error out"=w610:errorcluster)  [unwired: 4 in, 4 out]
                    n384 = Bundle By Name(cluster=cluster{"cmd":T5, "data":variant} {"cmd"=enum."ENG.PROC.STOP", "data"=variant} ("typedefElement"), "data"=w604) -> (w602:cluster{"cmd":T5, "data":variant})
                    n385 = Bundle By Name(cluster=cluster{"cmd":T5, "data":variant} {"cmd"=enum."ENG.PROC.RELOAD-BY-NAME", "data"=variant} ("typedefElement"), "data"=w604) -> (w609:cluster{"cmd":T5, "data":variant})
                    n386 = Build Array(w602, w609) -> (w603:cluster{"cmd":T5, "data":variant}[])
                    n387 = for {
                      tunnel: w606 -> [w614]
                      tunnel: w603 -> [w613] mode=indexing
                      shift-right: [w615] -> w607
                      shift-left: w610 -> [w616]
                      n388 = Enqueue Element(queue=w614, element=w613, error in (no error)=w616) -> (error out=w615:errorcluster)  [unwired: 1 in, 2 out]
                    }
                    n389 = invoke on="PBR_PLAY" class="Clust (strict)" method="Reinit To Default"() -> ()  [unwired: 3 in, 3 out]
                  }
                }
              }
              frame "SAVEAS" {
                n390 = call "ui-form-text-line.vi"("User Prompt in"="Insert Procedure Name (ie. HARVEST1)") -> ("Cancelled?"=w621:bool, "text out"=w620:string)  [unwired: 9 in]
                n391 = Concatenate Strings("PBR\\" ("string"), w620) -> (w618:string)
                n392 = case shown="False" w621 {
                  tunnel: [w624 _] -> w623
                  tunnel: w618 -> [w631 _]
                  tunnel: w617 -> [w634 _]
                  frame False {
                    n393 = call "util.file.vars.vi"("Operation(Read)"=enum16{"Read File", "Write File"}."Write File", "Proc Name(open dialog if empty)"=w631, "Vars[] in"=w634) -> ("error out"=w630:errorcluster, "File path"=w626:path)  [unwired: 4 in, 3 out]
                    n394 = call "pbr-get-procs-names.vi"("error in"=w630) -> ("error out"=w632:errorcluster, "Array"=w633:string[])  [unwired: 9 in]
                    n395 = global read "globals-engine.vi" "Q-Eng"() -> (w627:refnum<queue>)
                    n396 = property on="PBR PROC" class="CmbBox"(error in=w632, "Strings[]"=w633, "Value"=w631) -> (error out=w625:errorcluster)  [unwired: 1 in, 1 out]
                    n397 = Bundle By Name(cluster=cluster{"cmd":T5, "data":variant} {"cmd"=enum."ENG.LOAD.SINGLE", "data"=variant} ("typedefElement"), "data"=w626) -> (w629:cluster{"cmd":T5, "data":variant})
                    n398 = Enqueue Element(queue=w627, element=w629, error in (no error)=w625) -> (error out=w624:errorcluster)  [unwired: 1 in, 2 out]
                  }
                  frame True {
                  }
                }
              }
              frame "LOAD" {
                n399 = local read "PBR Builder"() -> (w640:T23)
                n400 = Empty Array?(array=w640) -> (empty?=w639:bool)
                n401 = case shown="False" w639 {
                  selector: w639 -> [_ w647]
                  tunnel: [w646 w647] -> w641
                  tunnel: w638 -> [w643 _]
                  frame False {
                    n402 = Format Into String(format string="Load %s?", w643) -> (resulting string=w644:string)  [unwired: 2 in, 1 out]
                    n403 = Two Button Dialog(message=w644) -> (T button?=w646:bool)  [unwired: 2 in]
                  }
                  frame True {
                  }
                }
                n404 = case shown="True" w641 {
                  tunnel: [_ w651] -> w642
                  tunnel: w638 -> [_ w650]
                  tunnel: [w648 w649] -> w637
                  tunnel: w636 -> [w648 _]
                  frame False {
                    # "Cancelled"
                  }
                  frame True {
                    # "Continue"
                    n405 = call "util.file.vars.vi"("Operation(Read)"=enum16{"Read File", "Write File"}."Read File", "Directory (DIR_PROC)"=typePathSelector."DIR_PROCS", "Proc Name(open dialog if empty)"=w650) -> ("error out"=w654:errorcluster, "Vars[] out"=w649:variant[])  [unwired: 4 in, 3 out]
                    n406 = call "build.proc.parse.vi"("error"=w654, "Array in"=w649) -> ("error out"=w652:errorcluster, "Flow Steps"=w656:T49[])  [unwired: 7 in, 1 out]
                    n407 = call "pbr-builder.vi"("FLOW in"=w656) -> ("PBR FLOW OUT"=w655:T23)  [unwired: 8 in, 2 out]
                    n408 = local write "PBR Builder"(w655) -> ()
                    n409 = invoke on="PBR_PLAY" class="Clust (strict)" method="Reinit To Default"() -> ()  [unwired: 3 in, 3 out]
                    n410 = property on="COMPILE" class="Bool (strict)"(error in=w652, "Val(Sgnl)"=TRUE ("Value (Signaling)")) -> (error out=w651:errorcluster)  [unwired: 1 in, 1 out]
                  }
                }
              }
            }
            n411 = feedback-in #2(w575) -> ()
            n412 = call <vilib>:"Clear Errors.vi"("error in (no error)"=w579) -> ("error out"=w577:errorcluster)  [unwired: 5 in, 1 out]
          }
          event "PBR_PLAY.PLAY", "PBR_PLAY.PAUSE", "PBR_PLAY.STOP": Value Change {
            n413 = event-data() -> ("CtlRef"=w665:refnum<vi>)  [unwired: 1 in]
            n414 = property class="Bool (strict)"(reference=w665) -> (reference out=w662:refnum<vi>, "Label.Text"=w664:string, "Value"=w660:bool)  [unwired: 1 in, 1 out]
            n415 = case shown="True" w660 {
              tunnel: w664 -> [_ w671]
              tunnel: [_ w670] -> w663
              tunnel: [TRUE ("T button?") w668] -> w661
              frame False {
              }
              frame True {
                n416 = global read "globals-engine.vi" "Q-Eng"() -> (w669:refnum<queue>)
                n417 = local read "PBR PROC"() -> (w667:string)
                n418 = case shown="\"STOP\"" w671 {
                  tunnel: [_ w677 w688 w699] -> w670
                  tunnel: w667 -> [_ w673 w684 w695]
                  tunnel: w669 -> [_ w676 w687 w698]
                  tunnel: [_ w675 w686 w697] -> w668
                  frame "False", Default {
                  }
                  frame "PLAY" {
                    n419 = Format Into String(format string="Start %s?", w673) -> (resulting string=w672:string)  [unwired: 2 in, 1 out]
                    n420 = Two Button Dialog(message=w672) -> (T button?=w675:bool)  [unwired: 2 in]
                    n421 = case shown="True" w675 {
                      tunnel: [_ w681] -> w677
                      tunnel: w673 -> [_ w678]
                      tunnel: w676 -> [_ w679]
                      frame False {
                      }
                      frame True {
                        n422 = Bundle By Name(cluster=cluster{"cmd":T5, "data":variant} {"cmd"=enum."ENG.PROC.START", "data"=variant} ("typedefElement"), "data"=w678) -> (w682:cluster{"cmd":T5, "data":variant})
                        n423 = Enqueue Element(queue=w679, element=w682) -> (error out=w681:errorcluster)  [unwired: 2 in, 2 out]
                      }
                    }
                  }
                  frame "PAUSE" {
                    n424 = Format Into String(format string="Pause %s?", w684) -> (resulting string=w683:string)  [unwired: 2 in, 1 out]
                    n425 = Two Button Dialog(message=w683) -> (T button?=w686:bool)  [unwired: 2 in]
                    n426 = case shown="True" w686 {
                      tunnel: [_ w692] -> w688
                      tunnel: w684 -> [_ w690]
                      tunnel: w687 -> [_ w689]
                      frame False {
                      }
                      frame True {
                        n427 = Bundle By Name(cluster=cluster{"cmd":T5, "data":variant} {"cmd"=enum."ENG.PROC.STOP", "data"=variant} ("typedefElement"), "data"=w690) -> (w693:cluster{"cmd":T5, "data":variant})
                        n428 = Enqueue Element(queue=w689, element=w693) -> (error out=w692:errorcluster)  [unwired: 2 in, 2 out]
                      }
                    }
                  }
                  frame "STOP" {
                    n429 = Format Into String(format string="Stop %s?", w695) -> (resulting string=w694:string)  [unwired: 2 in, 1 out]
                    n430 = Two Button Dialog(message=w694) -> (T button?=w697:bool)  [unwired: 2 in]
                    n431 = case shown="True" w697 {
                      tunnel: [_ w703] -> w699
                      tunnel: w695 -> [_ w701]
                      tunnel: w698 -> [_ w700]
                      frame False {
                      }
                      frame True {
                        n432 = Bundle By Name(cluster=cluster{"cmd":T5, "data":variant} {"cmd"=enum."ENG.PROC.RELOAD-BY-NAME", "data"=variant} ("typedefElement"), "data"=w701) -> (w704:cluster{"cmd":T5, "data":variant})
                        n433 = Enqueue Element(queue=w700, element=w704) -> (error out=w703:errorcluster)  [unwired: 2 in, 2 out]
                      }
                    }
                  }
                }
              }
            }
            n434 = case shown="True" w661 {
              selector: w661 -> [_ w705]
              tunnel: [_ w705] -> w659
              frame False {
              }
              frame True {
                n435 = invoke on="PBR_PLAY" class="Clust (strict)" method="Reinit To Default"() -> ()  [unwired: 3 in, 3 out]
              }
            }
            n436 = property class="Bool (strict)"(reference=w662, "Value"=w659) -> ()  [unwired: 1 in, 2 out]
          }
          event "PRBmenu.Harvest", "PRBmenu.SANI": Value Change {
            n437 = event-data() -> ("CtlRef"=w710:refnum<vi>)  [unwired: 1 in]
            n438 = property class="Bool (strict)"(reference=w710, "Value"=FALSE) -> ("Label.Text"=w709:string)  [unwired: 1 in, 2 out]
            n439 = case shown="\"False\", Default" w709 {
              tunnel: [_ w714 w720] -> w708
              tunnel: w706 -> [_ w711 _]
              frame "False", Default {
              }
              frame "Harvest" {
                n440 = local write "last"(w711) -> ()
                n441 = global read "globals-engine.vi" "Q-Eng"() -> (w717:refnum<queue>)
                n442 = Bundle By Name(cluster=cluster{"case":T5, "data":variant} {"case"=enum."ENG.PROC.START", "data"=variant} ("element"), "case"=state-engine."ENG.PROC.START", "data"="PBR\\HARVEST1") -> (w715:cluster{"case":T5, "data":variant})
                n443 = Enqueue Element(queue=w717, element=w715) -> (error out=w714:errorcluster)  [unwired: 2 in, 2 out]
              }
              frame "SANI" {
                n444 = global read "globals-engine.vi" "Q-Eng"() -> (w723:refnum<queue>)
                n445 = Bundle By Name(cluster=cluster{"case":T5, "data":variant} {"case"=enum."ENG.PROC.START", "data"=variant} ("element"), "case"=state-engine."ENG.PROC.START", "data"="PBR\\SANI") -> (w721:cluster{"case":T5, "data":variant})
                n446 = Enqueue Element(queue=w723, element=w721) -> (error out=w720:errorcluster)  [unwired: 2 in, 2 out]
              }
            }
          }
          event "Proc Select 2": Value Change {
            n447 = event-data() -> ()  [unwired: 1 in, 1 out]
            n448 = global read "globals-engine.vi" "Q-Eng"() -> (w725:refnum<queue>)
            n449 = Enqueue Element(queue=w725, element=cluster{"case":T5, "data":variant} {"case"=enum."ENG.PROC.STATUS", "data"=variant}) -> (error out=w726:errorcluster)  [unwired: 2 in, 2 out]
          }
          event "UiProjectSettings", "projectName": Value Change {
            n450 = event-data() -> ()  [unwired: 1 in, 6 out]
            n451 = local read "projectName"() -> (w727:string)
            n452 = Unbundle By Name("UiProjectSettings") -> ("Latitude"=w730:dbl, "Longitude"=w729:dbl, "TimeZone"=w728:i32)
            n453 = Bundle By Name(cluster="ProjectSettings", "Latitude"=w730, "Longitude"=w729, "TimeZone"=w728, "Project Name"=w727) -> (w731:T12)
            n454 = call "util-path.vi"("Create Folders?(F)"=FALSE, "Selected Folder (PROCS)"=typePathSelector."DIR_INI" ("Selected Folder (PROCEDURE_DIR)")) -> ("error out"=w747:errorcluster, "SelectedPath"=w748:path)  [unwired: 5 in, 3 out]
            n455 = Unbundle By Name(w731) -> ("Longitude"=w741:dbl, "Latitude"=w740:dbl, "TimeZone"=w739:i32, "Project Name"=w738:string)
            n456 = call <vilib>:"Open Config Data.vi"("error in (no error)"=w747, "configuration file path"=w748) -> ("error out"=w737:errorcluster, "refnum"=w744:T63)  [unwired: 7 in, 1 out]
            n457 = case shown="No Error" w737 {
              selector: w737 -> [_ w907]
              tunnel: w744 -> [w760 w906]
              tunnel: [_ w907] -> w743
              tunnel: [w759 w906] -> w742
              tunnel: w741 -> [w755 _]
              tunnel: w740 -> [w754 _]
              tunnel: w739 -> [w753 _]
              tunnel: w738 -> [w752 _]
              tunnel: [w750 _] -> w736
              frame No Error {
                n458 = stacked-sequence {
                  tunnel: [_ w800 _ _] -> w757
                  tunnel: w760 -> [w764 w799 w836 w872]
                  tunnel: [w763 _ _ _] -> w758
                  tunnel: [w762 _ _ _] -> w759
                  tunnel: [_ _ w835 _] -> w756
                  tunnel: w755 -> [w761 _ _ _]
                  tunnel: w754 -> [_ w798 _ _]
                  tunnel: w753 -> [_ _ w834 _]
                  tunnel: w752 -> [_ _ _ w871]
                  tunnel: [_ _ _ w870] -> w751
                  frame #0 {
                    w772 = 500  # timeout ms default
                    w787 = 500  # timeout ms default
                    n459 = call "util-path.vi"("Create Folders?(F)"=FALSE, "Selected Folder (PROCS)"=typePathSelector."DIR_INI" ("Selected Folder (PROCEDURE_DIR)")) -> ("error out"=w797:errorcluster, "SelectedPath"=w795:path)  [unwired: 5 in, 3 out]
                    n460 = call <vilib>:"Open Config Data.vi"("error in (no error)"=w797, "configuration file path"=w795) -> ("error out"=w796:errorcluster, "refnum"=w794:T63)  [unwired: 7 in, 1 out]
                    n461 = call "util-ini-key.vi"("key"=ini-key."INI.ENG.INTERVAL_MS" ("input 1")) -> ("key"=w791:string, "section"=w783:string)  [unwired: 9 in]
                    n462 = call-poly <vilib>:"Read Key.vi"("section"=w783, "error in (no error)"=w796, "key"=w791, "refnum"=w794) -> ("error out"=w793:errorcluster, "value"=w784:i32, "found?"=w786:bool, "refnum out"=w792:T63)  [unwired: 4 in]
                    n463 = call <vilib>:"Close Config Data.vi"("error in (no error)"=w793, "refnum"=w792) -> ()  [unwired: 8 in, 2 out]
                    n464 = call "util-path.vi"("Create Folders?(F)"=FALSE, "Selected Folder (PROCS)"=typePathSelector."DIR_INI" ("Selected Folder (PROCEDURE_DIR)")) -> ("error out"=w782:errorcluster, "SelectedPath"=w780:path)  [unwired: 5 in, 3 out]
                    n465 = Select(t=w784, s=w786, f=w787) -> (s? t:f=w785:i32)
                    n466 = call <vilib>:"Open Config Data.vi"("error in (no error)"=w782, "configuration file path"=w780) -> ("error out"=w781:errorcluster, "refnum"=w779:T63)  [unwired: 7 in, 1 out]
                    n467 = call "util-ini-key.vi"("key"=ini-key."INI.ENG.INTERVAL_MS" ("input 1")) -> ("key"=w776:string, "section"=w768:string)  [unwired: 9 in]
                    n468 = local write "ENG ms ctrl 9"(w785) -> ()
                    n469 = call "util-ini-key.vi"("key"=ini-key."INI.LOCAL.LONGITUDE" ("input 1")) -> ("key"=w767:string, "section"=w765:string)  [unwired: 9 in]
                    n470 = call-poly <vilib>:"Read Key.vi"("section"=w768, "error in (no error)"=w781, "key"=w776, "refnum"=w779) -> ("error out"=w778:errorcluster, "value"=w769:i32, "found?"=w771:bool, "refnum out"=w777:T63)  [unwired: 4 in]
                    n471 = call-poly <vilib>:"Write Key.vi"("section"=w765, "value"=w761, "key"=w767, "refnum"=w764) -> ("error out"=w763:errorcluster, "refnum out"=w762:T63)  [unwired: 5 in, 1 out]
                    n472 = call <vilib>:"Close Config Data.vi"("error in (no error)"=w778, "refnum"=w777) -> ()  [unwired: 8 in, 2 out]
                    n473 = Select(t=w769, s=w771, f=w772) -> (s? t:f=w770:i32)
                    n474 = local write "ENG ms ctrl 8"(w770) -> ()
                  }
                  frame #1 {
                    w808 = 500  # timeout ms default
                    w823 = 500  # timeout ms default
                    n475 = call "util-path.vi"("Create Folders?(F)"=FALSE, "Selected Folder (PROCS)"=typePathSelector."DIR_INI" ("Selected Folder (PROCEDURE_DIR)")) -> ("error out"=w833:errorcluster, "SelectedPath"=w831:path)  [unwired: 5 in, 3 out]
                    n476 = call <vilib>:"Open Config Data.vi"("error in (no error)"=w833, "configuration file path"=w831) -> ("error out"=w832:errorcluster, "refnum"=w830:T63)  [unwired: 7 in, 1 out]
                    n477 = call "util-ini-key.vi"("key"=ini-key."INI.ENG.INTERVAL_MS" ("input 1")) -> ("key"=w827:string, "section"=w819:string)  [unwired: 9 in]
                    n478 = call-poly <vilib>:"Read Key.vi"("section"=w819, "error in (no error)"=w832, "key"=w827, "refnum"=w830) -> ("error out"=w829:errorcluster, "value"=w820:i32, "found?"=w822:bool, "refnum out"=w828:T63)  [unwired: 4 in]
                    n479 = call <vilib>:"Close Config Data.vi"("error in (no error)"=w829, "refnum"=w828) -> ()  [unwired: 8 in, 2 out]
                    n480 = call "util-path.vi"("Create Folders?(F)"=FALSE, "Selected Folder (PROCS)"=typePathSelector."DIR_INI" ("Selected Folder (PROCEDURE_DIR)")) -> ("error out"=w818:errorcluster, "SelectedPath"=w816:path)  [unwired: 5 in, 3 out]
                    n481 = Select(t=w820, s=w822, f=w823) -> (s? t:f=w821:i32)
                    n482 = call <vilib>:"Open Config Data.vi"("error in (no error)"=w818, "configuration file path"=w816) -> ("error out"=w817:errorcluster, "refnum"=w815:T63)  [unwired: 7 in, 1 out]
                    n483 = call "util-ini-key.vi"("key"=ini-key."INI.ENG.INTERVAL_MS" ("input 1")) -> ("key"=w812:string, "section"=w804:string)  [unwired: 9 in]
                    n484 = call "util-ini-key.vi"("key"=ini-key."INI.LOCAL.LATITUDE" ("input 1")) -> ("key"=w803:string, "section"=w801:string)  [unwired: 9 in]
                    n485 = local write "ENG ms ctrl 11"(w821) -> ()
                    n486 = call-poly <vilib>:"Read Key.vi"("section"=w804, "error in (no error)"=w817, "key"=w812, "refnum"=w815) -> ("error out"=w814:errorcluster, "value"=w805:i32, "found?"=w807:bool, "refnum out"=w813:T63)  [unwired: 4 in]
                    n487 = call-poly <vilib>:"Write Key.vi"("section"=w801, "value"=w798, "key"=w803, "refnum"=w799) -> ("error out"=w800:errorcluster)  [unwired: 5 in, 2 out]
                    n488 = call <vilib>:"Close Config Data.vi"("error in (no error)"=w814, "refnum"=w813) -> ()  [unwired: 8 in, 2 out]
                    n489 = Select(t=w805, s=w807, f=w808) -> (s? t:f=w806:i32)
                    n490 = local write "ENG ms ctrl 10"(w806) -> ()
                  }
                  frame #2 {
                    w844 = 500  # timeout ms default
                    w859 = 500  # timeout ms default
                    n491 = call "util-path.vi"("Create Folders?(F)"=FALSE, "Selected Folder (PROCS)"=typePathSelector."DIR_INI" ("Selected Folder (PROCEDURE_DIR)")) -> ("error out"=w869:errorcluster, "SelectedPath"=w867:path)  [unwired: 5 in, 3 out]
                    n492 = call <vilib>:"Open Config Data.vi"("error in (no error)"=w869, "configuration file path"=w867) -> ("error out"=w868:errorcluster, "refnum"=w866:T63)  [unwired: 7 in, 1 out]
                    n493 = call "util-ini-key.vi"("key"=ini-key."INI.ENG.INTERVAL_MS" ("input 1")) -> ("key"=w863:string, "section"=w855:string)  [unwired: 9 in]
                    n494 = call-poly <vilib>:"Read Key.vi"("section"=w855, "error in (no error)"=w868, "key"=w863, "refnum"=w866) -> ("error out"=w865:errorcluster, "value"=w856:i32, "found?"=w858:bool, "refnum out"=w864:T63)  [unwired: 4 in]
                    n495 = call <vilib>:"Close Config Data.vi"("error in (no error)"=w865, "refnum"=w864) -> ()  [unwired: 8 in, 2 out]
                    n496 = call "util-path.vi"("Create Folders?(F)"=FALSE, "Selected Folder (PROCS)"=typePathSelector."DIR_INI" ("Selected Folder (PROCEDURE_DIR)")) -> ("error out"=w854:errorcluster, "SelectedPath"=w852:path)  [unwired: 5 in, 3 out]
                    n497 = Select(t=w856, s=w858, f=w859) -> (s? t:f=w857:i32)
                    n498 = call <vilib>:"Open Config Data.vi"("error in (no error)"=w854, "configuration file path"=w852) -> ("error out"=w853:errorcluster, "refnum"=w851:T63)  [unwired: 7 in, 1 out]
                    n499 = call "util-ini-key.vi"("key"=ini-key."INI.ENG.INTERVAL_MS" ("input 1")) -> ("key"=w848:string, "section"=w840:string)  [unwired: 9 in]
                    n500 = local write "ENG ms ctrl 13"(w857) -> ()
                    n501 = call "util-ini-key.vi"("key"=ini-key."INI.LOCAL.TIMEZONE" ("input 1")) -> ("key"=w839:string, "section"=w837:string)  [unwired: 9 in]
                    n502 = call-poly <vilib>:"Read Key.vi"("section"=w840, "error in (no error)"=w853, "key"=w848, "refnum"=w851) -> ("error out"=w850:errorcluster, "value"=w841:i32, "found?"=w843:bool, "refnum out"=w849:T63)  [unwired: 4 in]
                    n503 = call-poly <vilib>:"Write Key.vi"("section"=w837, "value"=w834, "key"=w839, "refnum"=w836) -> ("error out"=w835:errorcluster)  [unwired: 5 in, 2 out]
                    n504 = call <vilib>:"Close Config Data.vi"("error in (no error)"=w850, "refnum"=w849) -> ()  [unwired: 8 in, 2 out]
                    n505 = Select(t=w841, s=w843, f=w844) -> (s? t:f=w842:i32)
                    n506 = local write "ENG ms ctrl 12"(w842) -> ()
                  }
                  frame #3 {
                    w880 = 500  # timeout ms default
                    w895 = 500  # timeout ms default
                    n507 = call "util-path.vi"("Create Folders?(F)"=FALSE, "Selected Folder (PROCS)"=typePathSelector."DIR_INI" ("Selected Folder (PROCEDURE_DIR)")) -> ("error out"=w905:errorcluster, "SelectedPath"=w903:path)  [unwired: 5 in, 3 out]
                    n508 = call <vilib>:"Open Config Data.vi"("error in (no error)"=w905, "configuration file path"=w903) -> ("error out"=w904:errorcluster, "refnum"=w902:T63)  [unwired: 7 in, 1 out]
                    n509 = call "util-ini-key.vi"("key"=ini-key."INI.ENG.INTERVAL_MS" ("input 1")) -> ("key"=w899:string, "section"=w891:string)  [unwired: 9 in]
                    n510 = call-poly <vilib>:"Read Key.vi"("section"=w891, "error in (no error)"=w904, "key"=w899, "refnum"=w902) -> ("error out"=w901:errorcluster, "value"=w892:i32, "found?"=w894:bool, "refnum out"=w900:T63)  [unwired: 4 in]
                    n511 = call <vilib>:"Close Config Data.vi"("error in (no error)"=w901, "refnum"=w900) -> ()  [unwired: 8 in, 2 out]
                    n512 = call "util-path.vi"("Create Folders?(F)"=FALSE, "Selected Folder (PROCS)"=typePathSelector."DIR_INI" ("Selected Folder (PROCEDURE_DIR)")) -> ("error out"=w890:errorcluster, "SelectedPath"=w888:path)  [unwired: 5 in, 3 out]
                    n513 = Select(t=w892, s=w894, f=w895) -> (s? t:f=w893:i32)
                    n514 = call <vilib>:"Open Config Data.vi"("error in (no error)"=w890, "configuration file path"=w888) -> ("error out"=w889:errorcluster, "refnum"=w887:T63)  [unwired: 7 in, 1 out]
                    n515 = call "util-ini-key.vi"("key"=ini-key."INI.ENG.INTERVAL_MS" ("input 1")) -> ("key"=w884:string, "section"=w876:string)  [unwired: 9 in]
                    n516 = local write "ENG ms ctrl 15"(w893) -> ()
                    n517 = call "util-ini-key.vi"("key"=ini-key."INI.PROJECT_NAME" ("input 1")) -> ("key"=w875:string, "section"=w873:string)  [unwired: 9 in]
                    n518 = call-poly <vilib>:"Read Key.vi"("section"=w876, "error in (no error)"=w889, "key"=w884, "refnum"=w887) -> ("error out"=w886:errorcluster, "value"=w877:i32, "found?"=w879:bool, "refnum out"=w885:T63)  [unwired: 4 in]
                    n519 = call-poly <vilib>:"Write Key.vi"("section"=w873, "value"=w871, "key"=w875, "refnum"=w872) -> ("error out"=w870:errorcluster)  [unwired: 5 in, 2 out]
                    n520 = call <vilib>:"Close Config Data.vi"("error in (no error)"=w886, "refnum"=w885) -> ()  [unwired: 8 in, 2 out]
                    n521 = Select(t=w877, s=w879, f=w880) -> (s? t:f=w878:i32)
                    n522 = local write "ENG ms ctrl 14"(w878) -> ()
                  }
                }
                n523 = Merge Errors(w758, w757, w756, w751) -> (w750:errorcluster)
              }
              frame Error {
              }
            }
            n524 = call <vilib>:"Close Config Data.vi"("error in (no error)"=w743, "refnum"=w742) -> ("error out"=w735:errorcluster)  [unwired: 8 in, 1 out]
            n525 = Merge Errors(w735, w736) -> (w734:errorcluster)
            n526 = case shown="No Error" w734 {
              tunnel: w731 -> [w749 _]
              frame No Error {
                n527 = global write "globals-engine.vi" "ProjectSettings"(w749) -> ()
              }
              frame Error {
              }
            }
          }
          event "read buffer": Value Change {
            w911 = T79 4 items=["(0) RxStart", "(1) XOR", "(2) DataSize", "(3) Address", "(4) Type"] ("Enum")
            w912 = T79 3 items=["(0) RxStart", "(1) XOR", "(2) DataSize", "(3) Address", "(4) Type"] ("Enum")
            w913 = T79 2 items=["(0) RxStart", "(1) XOR", "(2) DataSize", "(3) Address", "(4) Type"] ("Enum")
            w908 = T42 {"ADDR"=0, "Label"="Name", "Type"=enum."DI", "Mode"=enum."RIO", "Value"="Value", "Tags"="Tags", "calibration"=[]} ("IoConf in")
            n528 = event-data() -> ()  [unwired: 1 in, 1 out]
            n529 = Unbundle By Name(w908) -> ("Type"=w921:T3)
            n530 = String To Byte Array(string="read buffer") -> (unsigned byte array=w915:u8[])
            n531 = call "io.responseValidator.vi"("ResponsToValidate in"="read buffer", "IoConf in 2"=w908) -> ("error out"=w919:errorcluster, "Data out"=w920:string)  [unwired: 8 in]
            "Command Payload" <- w920
            n532 = Index Array(array=w915, index #1=w913, index #2=w912, index #3=w911) -> (element #1=→"Data Size":u8, element #2=→"Address":u8, element #3=→"Type":u8)  [unwired: 3 in, 3 out]
            n533 = case "parse response" shown="\"DI\"" w921 {
              tunnel: w920 -> [_ w924 w934]
              tunnel: [w922 w928 w933] -> _
              tunnel: [_ w927 w932] -> w918
              tunnel: w908 -> [_ w923 w931]
              tunnel: [_ _ w930] -> w917
              tunnel: [_ w926 _] -> _
              tunnel: w919 -> [w922 w925 w929]
              frame Default {
              }
              frame "DI" {
                n534 = call "io.command-parser.DI.vi"("error in (no error)"=w925, "Reponse in"=w924, "IoConf out"=w923) -> ("error out"=w928:errorcluster, "dports"=w926:bool[], "DI out"=w927:dbl)  [unwired: 6 in]
              }
              frame "AI" {
                # "Parse Analog In responses,  (1) filter min/max and \n(2) average the rest"
                n535 = call "io.command-parser.AI.vi"("error in"=w929, "Reponse in"=w934, "IoConf in"=w931) -> ("error out"=w933:errorcluster, "AI uncalib out"=w930:u16, "AI out"=w932:dbl)  [unwired: 6 in]
              }
            }
            "AI out" <- w918
            "AI uncalib out" <- w917
          }
          event "Section": Value Change {
            n536 = event-data() -> ()  [unwired: 1 in, 1 out]
            n537 = local write "indoorStatus"(T27 {"Tdry"="", "Twet"="", "Humidity"=""} ("OutdoorStatus 3")) -> ()
          }
          event "SerialPort": Value Change {
            n538 = event-data() -> ("OldVal"=w938:refnum<visa-resource-name>, "NewVal"=w937:refnum<visa-resource-name>)  [unwired: 1 in]
            n539 = call "util-serial-init.vi"("NewVal"=w937, "Port"=w938) -> ("error out"=w936:errorcluster)  [unwired: 9 in]
          }
          event "Show Undefined": Value Change {
            w939 = "" ("By Tag")
            n540 = event-data() -> ()  [unwired: 1 in, 1 out]
            n541 = local read "IO Search Map"() -> (w941:T41)
            n542 = Bundle By Name(cluster=w941, "By Name"=w939, "By Tag"=w939) -> (w940:T41)
            n543 = property on="IO Search Map" class="Clust (strict)"("Val(Sgnl)"=w940) -> ()  [unwired: 2 in, 2 out]
            n544 = disable-structure shown="Disabled" {
              frame Disabled {
                n545 = local read "IO Search Conf"() -> (w942:T45)
                n546 = property on="IO Search Conf" class="Clust (strict)"("Val(Sgnl)"=w942) -> ()  [unwired: 2 in, 2 out]
              }
              frame Enabled {
              }
            }
          }
          event "Simulate Clock Reset": Value Change {
            n547 = event-data() -> ()  [unwired: 1 in, 1 out]
            n548 = local write "Clk Simulator"(timestamp(0 s since 1904-01-01) ("Time Stamp")) -> ()
          }
          event "Simulators": Value Change {
            n549 = event-data() -> ("OldVal"=w945:cluster{"Input ":string, "Value":string}[], "NewVal"=w944:cluster{"Input ":string, "Value":string}[])  [unwired: 1 in, 1 out]
            n550 = Not Equal?(x=w945, y=w944) -> (x != y?=w946:cluster{"Input ":bool, "Value":bool}[])
            n551 = disable-structure shown="Enabled" {
              disable-tunnel: w946 -> [w954 _]
              disable-tunnel: w944 -> [w949 _]
              frame Disabled {
                n552 = Array Max & Min(array=w954) -> (max index (indices)=w953:i32)  [unwired: 3 out]
                n553 = Index Array(array=w954, index=w953) -> ()  [unwired: 1 out]
                n554 = Index Array(array=w949, index=w953) -> (element=w951:cluster{"Input ":string, "Value":string})
                n555 = Unbundle By Name(w951) -> ("Input"=w950:string)  [unwired: 1 out]
                n556 = call "variantCtrlIo.vi"("isRequired (T)"=FALSE, "menu (Get Param)"=enumVarCtrlIO."IO Get By Key" ("menu (get)"), "Key (use IOnode Label if empty )"=w950) -> ()  [unwired: 4 in, 5 out]
              }
              frame Enabled {
              }
            }
            n557 = for {
              tunnel: [w956] -> w947 if=w955
              tunnel: w944 -> [w959] mode=indexing
              n558 = Unbundle By Name(w959) -> ("Input"=w957:string, "Value"=w958:string)
              n559 = case shown="Default" w957 {
                selector: w957 -> [_ w964]
                tunnel: [_ w962] -> w956
                tunnel: w958 -> [_ w966]
                frame "" {
                  # "empty input when input is cleared - ignore it"
                }
                frame Default {
                  # "Access HW if Empty"
                  # "validate input name is not empty"
                  n560 = call "variantCtrlIo.vi"("menu (Get Param)"=enumVarCtrlIO."IO Get By Key", "Key (use IOnode Label if empty )"=w964) -> ("error out"=w973:errorcluster, "IOnode out"=w970:T42)  [unwired: 5 in, 3 out]
                  n561 = Empty String/Path?(string/path=w966) -> (empty?=w971:bool)
                  n562 = Select(t=enum.io.mode."RIO", s=w971, f=enum.io.mode."SIM" ("Mode")) -> (s? t:f=w972:T38)
                  n563 = Bundle By Name(cluster=w970, "Value"=w966, "Mode"=w972) -> (w960:T42)
                  n564 = call "variantCtrlIo.vi"("menu (Get Param)"=enumVarCtrlIO."IO Modify Value By Key" ("menu (get)"), "error in"=w973, "IOnode in"=w960) -> ("error out"=w963:errorcluster)  [unwired: 4 in, 4 out]
                  n565 = call "variantCtrlIo.vi"("menu (Get Param)"=enumVarCtrlIO."IO Modify Mode By Key" ("menu (get)"), "error in"=w963, "IOnode in"=w960) -> ("error out"=w962:errorcluster)  [unwired: 4 in, 4 out]
                }
              }
              n566 = Unbundle By Name(w956) -> ("status"=w955:bool)
            }
          }
          event "Tab NTR": Value Change {
            n567 = event-data() -> ()  [unwired: 1 in, 1 out]
            n568 = case shown="\"Nutrition\"" "Tab NTR" {
              frame "Nutrition Flow", Default {
              }
              frame "Nutrition" {
                n569 = call "util.ntr.dose-aux.vi"() -> ("DO Dose pumps"=w979:string[])  [unwired: 7 in, 4 out]
                n570 = call "util-path.vi"("Selected Folder (PROCS)"=typePathSelector."DIR_RECORD", "append path (ie. folder\\filename.*)"="NTR\\NUTRITION" ("append path (ie. folder\\filename.*)")) -> ("SelectedPath"=w976:path)  [unwired: 5 in, 4 out]
                n571 = List Folder(path=w976) -> (folder names=w975:string[])  [unwired: 3 in, 3 out]
                n572 = Index Array(array=w975) -> (element=w980:string)  [unwired: 1 in]
                n573 = property on="ntrInputSelect" class="CmbBox"("Strings[]"=w975, "Value"=w980) -> ()  [unwired: 2 in, 2 out]
                n574 = Index Array(array=w979) -> (element=w981:string)  [unwired: 1 in]
                n575 = property on="ntrDosepumpSelect" class="CmbBox"("Strings[]"=w979, "Value"=w981) -> ()  [unwired: 2 in, 2 out]
              }
            }
          }
          event "Temperature Graph Panel": Value Change {
            n576 = event-data() -> ("NewVal"=w994:T25)  [unwired: 1 in]
            n577 = local read "Section"() -> (w988:string)
            n578 = property on="refresh" class="Bool (strict)"("Value"=FALSE) -> ()  [unwired: 2 in, 2 out]
            n579 = Unbundle By Name(w994) -> ("lastDays"=w983:i8)
            n580 = stacked-sequence {
              tunnel: w994 -> [_ _ _ _ _]
              tunnel: [w998 _ _ _ _] -> w993
              tunnel: [w996 _ _ _ _] -> w992
              tunnel: [_ _ w1015 _ _] -> w984
              tunnel: [_ w1001 _ _ _] -> w991
              tunnel: [_ _ w1011 _ _] -> w989
              tunnel: w988 -> [_ _ w1010 w1027 _]
              tunnel: [_ _ _ w1026 _] -> w982
              tunnel: [_ _ _ w1025 _] -> w987
              tunnel: w983 -> [w995 w999 w1009 w1021 _]
              frame #0 {
                n581 = call "helper-build-graph.vi"("filename.*"="_H0_UV_*.rec", "lastDays"=w995) -> ("error out"=w998:errorcluster, "Multiple Plots (X Array and Y Array)"=w996:cluster{"X":dbl[], "Y":dbl[]})  [unwired: 7 in, 1 out]
              }
              frame #1 {
                w1000 = "_H0" ("string")
                n582 = Concatenate Strings(w1000, "_TDRY_*.rec" ("filename.*")) -> (w1005:string)
                n583 = Concatenate Strings(w1000, "_TWET_*.rec" ("filename.*")) -> (w1004:string)
                n584 = call "helper-build-graph.vi"("filename.*"=w1005, "lastDays"=w999) -> ("Multiple Plots (X Array and Y Array)"=w1007:cluster{"X":dbl[], "Y":dbl[]})  [unwired: 7 in, 2 out]
                n585 = call "helper-build-graph.vi"("filename.*"=w1004, "lastDays"=w999) -> ("Multiple Plots (X Array and Y Array)"=w1002:cluster{"X":dbl[], "Y":dbl[]})  [unwired: 7 in, 2 out]
                n586 = Build Array(w1007, w1002) -> (w1001:cluster{"X":dbl[], "Y":dbl[]}[])
              }
              frame #2 {
                w1008 = "_" ("string")
                n587 = Concatenate Strings(w1008, w1010, "_TDRY_*.rec" ("filename.*")) -> (w1018:string)
                n588 = Concatenate Strings(w1008, w1010, "_TWET_*.rec" ("filename.*")) -> (w1017:string)
                n589 = call "helper-build-graph.vi"("filename.*"=w1018, "lastDays"=w1009) -> ("error out"=w1013:errorcluster, "Multiple Plots (X Array and Y Array)"=w1020:cluster{"X":dbl[], "Y":dbl[]})  [unwired: 7 in, 1 out]
                n590 = call "helper-build-graph.vi"("filename.*"=w1017, "lastDays"=w1009) -> ("error out"=w1012:errorcluster, "Multiple Plots (X Array and Y Array)"=w1014:cluster{"X":dbl[], "Y":dbl[]})  [unwired: 7 in, 1 out]
                n591 = Build Array(w1020, w1014) -> (w1015:cluster{"X":dbl[], "Y":dbl[]}[])
                n592 = Merge Errors(w1013, w1012) -> (w1011:errorcluster)
              }
              frame #3 {
                n593 = Concatenate Strings("_" ("string"), w1027, "_RH_*.rec" ("filename.*")) -> (w1029:string)
                n594 = call "helper-build-graph.vi"("filename.*"="_H0_RH_*.rec", "lastDays"=w1021) -> ("error out"=w1031:errorcluster, "Multiple Plots (X Array and Y Array)"=w1032:cluster{"X":dbl[], "Y":dbl[]})  [unwired: 7 in, 1 out]
                n595 = call "helper-build-graph.vi"("filename.*"=w1029, "lastDays"=w1021) -> ("error out"=w1023:errorcluster, "Multiple Plots (X Array and Y Array)"=w1022:cluster{"X":dbl[], "Y":dbl[]})  [unwired: 7 in, 1 out]
                n596 = Build Array(w1032, w1022) -> (w1025:cluster{"X":dbl[], "Y":dbl[]}[])
                n597 = Merge Errors(w1031, w1023) -> (w1026:errorcluster)
              }
              frame #4 {
              }
            }
            "RH" <- w987
            "UV Graph" <- w992
            n598 = Build Array (concatenate)(w991, w984) -> (→"Outdoor Tdry Graph":cluster{"X":dbl[], "Y":dbl[]}[])
            n599 = Merge Errors(w993, w989, w982) -> (w990:errorcluster)
          }
          event "Template.templateSave", "Template.templateLoad", "Template.procedureLoad", "Template.procedureSaveAs", "Template.procedureSave", "Template.procedureReload": Value Change {
            w1039 = TRUE  # allowDialogs?(False)
            # "templateSave (save as text file)\ntemplateLoad (load from text file)\nprocedureSave(build flow and save as varient file)\nprocedureLoad(load from varient file and parse to flow)"
            n600 = event-data() -> ("CtlRef"=w1038:refnum<vi>)  [unwired: 1 in]
            n601 = property class="Bool (strict)"(reference=w1038, "Value"=FALSE) -> ("Label.Text"=w1044:string)  [unwired: 1 in, 2 out]
            n602 = Unbundle By Name("UiBuildProcHead") -> ("Procedure Name"=w1042:string)
            n603 = local read "File path"() -> (w1034:path)
            n604 = call "util-path-to-proc-name.vi"("File path"=w1034) -> ("String"=w1033:string)  [unwired: 10 in]
            n605 = case shown="\"procedureSave\"" w1044 {
              tunnel: "UiBuildProcHead" -> [w1050 w1069 _ _ _ _ _]
              tunnel: "UiBuildSteps" -> [w1049 w1068 _ _ w1111 w1121 _]
              tunnel: [w1048 w1067 w1084 w1095 w1110 w1119 errorcluster {"status"=TRUE, "code"=-564498, "source"="Case Error in gui.builder.vi's event"} ("error out")] -> w1040
              tunnel: w1042 -> [w1046 _ _ _ _ w1120 _]
              tunnel: w1039 -> [w1047 w1066 w1083 w1093 _ _ _]
              tunnel: w1033 -> [_ w1062 w1079 _ _ _ _]
              frame "procedureSaveAs" {
                # "procedureSave: build flow and save as varient file"
                n606 = disable-structure shown="Disabled" {
                  disable-tunnel: w1046 -> [w1051 _]
                  frame Disabled {
                    n607 = Format Into String(format string="Save Procedure as: %s?", w1051) -> (resulting string=w1053:string)  [unwired: 2 in, 1 out]
                    n608 = Two Button Dialog(message=w1053) -> ()  [unwired: 2 in, 1 out]
                  }
                  frame Enabled {
                  }
                }
                n609 = case shown="True" TRUE {
                  tunnel: w1050 -> [_ w1061]
                  tunnel: w1049 -> [_ w1060]
                  tunnel: [_ w1057] -> w1048
                  tunnel: w1047 -> [_ w1054]
                  frame False {
                    # "Cancelled"
                  }
                  frame True {
                    # "Continue"
                    n610 = call "build.proc.vi"("Flow"=w1060, "Proc Head"=w1061) -> ("error out"=w1056:errorcluster, "Instructions"=w1059:variant[])  [unwired: 8 in]
                    n611 = call "util.file.vars.vi"("Operation(Read)"=enum16{"Read File", "Write File"}."Write File", "allowDialogs?(False)"=w1054, "error in"=w1056, "Directory (DIR_PROC)"=typePathSelector."DIR_PROCS" ("location (PROCEDURE_DIR)"), "Vars[] in"=w1059) -> ("error out"=w1057:errorcluster)  [unwired: 2 in, 4 out]
                  }
                }
              }
              frame "procedureSave" {
                # "procedureSave: build flow and save as varient file"
                n612 = Format Into String(format string="Save Procedure as %s?", w1062) -> (resulting string=w1065:string)  [unwired: 2 in, 1 out]
                n613 = Two Button Dialog(message=w1065) -> (T button?=w1063:bool)  [unwired: 2 in]
                n614 = case shown="True" w1063 {
                  tunnel: w1069 -> [_ w1078]
                  tunnel: w1068 -> [_ w1077]
                  tunnel: [_ w1074] -> w1067
                  tunnel: w1066 -> [_ w1071]
                  tunnel: w1062 -> [_ w1070]
                  frame False {
                    # "Cancelled"
                  }
                  frame True {
                    # "Continue"
                    n615 = call "build.proc.vi"("Flow"=w1077, "Proc Head"=w1078) -> ("error out"=w1073:errorcluster, "Instructions"=w1076:variant[])  [unwired: 8 in]
                    n616 = call "util.file.vars.vi"("Operation(Read)"=enum16{"Read File", "Write File"}."Write File", "allowDialogs?(False)"=w1071, "error in"=w1073, "Directory (DIR_PROC)"=typePathSelector."DIR_PROCS" ("location (PROCEDURE_DIR)"), "Proc Name(open dialog if empty)"=w1070, "Vars[] in"=w1076) -> ("error out"=w1074:errorcluster)  [unwired: 1 in, 4 out]
                  }
                }
              }
              frame "procedureReload" {
                # "procedureSave: build flow and save as varient file"
                n617 = Format Into String(format string="Reload %s?", w1079) -> (resulting string=w1082:string)  [unwired: 2 in, 1 out]
                n618 = Two Button Dialog(message=w1082) -> (T button?=w1080:bool)  [unwired: 2 in]
                n619 = case shown="True" w1080 {
                  tunnel: [_ w1086] -> w1084
                  tunnel: w1083 -> [_ _]
                  tunnel: w1079 -> [_ w1087]
                  frame False {
                    # "Cancelled"
                  }
                  frame True {
                    # "Continue"
                    n620 = Bundle By Name(cluster=cluster{"cmd":T5, "data":variant} {"cmd"=enum."ENG.PROC.RELOAD-BY-NAME", "data"=variant} ("typedefElement"), "data"=w1087) -> (w1085:cluster{"cmd":T5, "data":variant})
                    n621 = global read "globals-engine.vi" "Q-Eng"() -> (w1089:refnum<queue>)
                    n622 = Enqueue Element(queue=w1089, element=w1085) -> (error out=w1086:errorcluster)  [unwired: 2 in, 2 out]
                  }
                }
              }
              frame "procedureLoad" {
                n623 = call "util.file.vars.vi"("allowDialogs?(False)"=w1093, "Directory (DIR_PROC)"=typePathSelector."DIR_PROCS" ("location (PROCEDURE_DIR)")) -> ("error out"=w1094:errorcluster, "cancelled?"=w1092:bool, "Vars[] out"=w1096:variant[], "File path"=w1090:path)  [unwired: 5 in, 1 out]
                n624 = case shown="False" w1092 {
                  tunnel: w1096 -> [w1102 _]
                  tunnel: [w1100 w1103] -> w1095
                  tunnel: w1094 -> [w1099 w1103]
                  tunnel: w1090 -> [w1097 _]
                  frame False {
                    # "not cancelled"
                    n625 = call "build.proc.parse.vi"("error"=w1099, "Array in"=w1102) -> ("error out"=w1100:errorcluster, "Flow Steps"=w1098:T49[], "Proc Head"=w1101:T48)  [unwired: 7 in]
                    n626 = local write "File path"(w1097) -> ()
                    n627 = local write "UiBuildSteps"(w1098) -> ()
                    n628 = local write "UiBuildProcHead"(w1101) -> ()
                  }
                  frame True {
                    # "cancelled"
                  }
                }
              }
              frame "templateLoad" {
                n629 = call "util.file.vars.path-parser.vi"("allowDialogs?(False)"=TRUE, "location (PROCEDURE_DIR)"=typePathSelector."DIR_TEMPLATE") -> ("error out"=w1106:errorcluster, "cancelled"=w1104:bool, "selected path"=w1108:path)  [unwired: 7 in]
                n630 = case shown="False" w1104 {
                  tunnel: w1111 -> [w1117 _]
                  tunnel: [w1116 w1118] -> w1110
                  tunnel: enum16{"Read", "Write"}."Read" ("Enum") -> [w1115 _]
                  tunnel: w1108 -> [w1114 _]
                  tunnel: w1106 -> [w1113 w1118]
                  frame False {
                    # "Not cancelled"
                    n631 = call "util.file.template.vi"("error in (no error)"=w1113, "Enum"=w1115, "sensor_flow"=w1117, "file path (dialog if empty)"=w1114) -> ("error out"=w1116:errorcluster, "Array"=w1112:T49[])  [unwired: 5 in, 1 out]
                    n632 = local write "UiBuildSteps"(w1112) -> ()
                  }
                  frame True {
                  }
                }
              }
              frame "templateSave" {
                n633 = stacked-sequence {
                  tunnel: w1121 -> [w1126]
                  tunnel: w1120 -> [_]
                  tunnel: [w1125] -> w1119
                  frame #0 {
                    n634 = call "ui-form-text-line.vi"("User Prompt in"="Enter template name.") -> ("Cancelled?"=w1122:bool, "text out"=w1123:string)  [unwired: 9 in]
                    n635 = case shown="False" w1122 {
                      tunnel: w1126 -> [w1137 _]
                      tunnel: [w1129 _] -> w1125
                      tunnel: w1123 -> [w1127 _]
                      frame False {
                        # "Not Cancelled"
                        n636 = call "util.file.vars.path-parser.vi"("allowDialogs?(False)"=TRUE, "location (PROCEDURE_DIR)"=typePathSelector."DIR_TEMPLATE", "Proc name"=w1127) -> ("selected path"=w1133:path)  [unwired: 6 in, 2 out]
                        n637 = call "util.file.template.vi"("Enum"=enum16{"Read", "Write"}."Write", "sensor_flow"=w1137, "file path (dialog if empty)"=w1133) -> ("error out"=w1130:errorcluster)  [unwired: 6 in, 2 out]
                        n638 = Format Into String(format string="%s saved as template.", initial string="", error in=w1130, w1127) -> (resulting string=w1131:string, error out=w1129:errorcluster)
                        n639 = One Button Dialog(message=w1131) -> ()  [unwired: 1 in, 1 out]
                      }
                      frame True {
                      }
                    }
                  }
                }
              }
              frame Default {
              }
            }
            n640 = call <vilib>:"Clear Errors.vi"("error in (no error)"=w1040, "specific error code to clear (0: all)"=43) -> ("error out"=w1036:errorcluster)  [unwired: 4 in, 1 out]
          }
          event "Title Bar Visible": Value Change {
            n641 = event-data() -> ()  [unwired: 1 in, 1 out]
            n642 = control-ref of="This VI"() -> (w1141:refnum<vi>)
            n643 = property class="VI"(reference=w1141, "Front Panel.TitleBarVis"="Title Bar Visible", "FP.State"=T57."Maximized" ("Front Panel Window:State")) -> ()  [unwired: 1 in, 2 out]
          }
          event "VISA REPORT.Clear": Value Change {
            n644 = event-data() -> ()  [unwired: 1 in, 1 out]
            n645 = call "reg-visa.vi"("Operation(Read)"=enum.report-filter."ClearAll") -> ()  [unwired: 9 in, 2 out]
          }
          event Value Change {
            n646 = event-data() -> ("CtlRef"=w1145:refnum<vi>, "NewVal"=w1148:variant, "OldVal"=w1149:variant)  [unwired: 1 in]
            n647 = property class="Ctl"(reference=w1145) -> (reference out=w1144:refnum<vi>, "Label.Text"=w1146:string)  [unwired: 1 in, 1 out]
            n648 = case shown="\"EastPosition\", \"WestPosition\"" w1146 {
              selector: w1146 -> [_ w1153 _]
              tunnel: w1149 -> [_ w1155 _]
              tunnel: w1148 -> [_ w1158 w1166]
              tunnel: [_ w1157 _] -> w1147
              tunnel: w1144 -> [_ w1156 _]
              tunnel: "WinView" -> [_ w1150 _]
              frame Default {
              }
              frame "EastPosition", "WestPosition" {
                n649 = call "helper-windows-control.vi"("Windows Panel"=w1150, "OldVal"=w1155, "NewVal"=w1158, "Label.Text"=w1153) -> ("error out"=w1157:errorcluster, "oldVal"=w1151:i32, "newVal"=w1152:i32, "canceled?"=w1154:bool)  [unwired: 4 in]
                n650 = case "Operation Canceled?" shown="False" w1154 {
                  tunnel: w1156 -> [_ w1164]
                  tunnel: w1151 -> [_ w1163]
                  tunnel: w1153 -> [w1160 _]
                  tunnel: w1152 -> [w1159 _]
                  frame False {
                    n651 = case "Update Views" shown="\"EastPosition\"" w1160 {
                      tunnel: w1159 -> [_ w1161 w1162]
                      frame Default {
                      }
                      frame "EastPosition" {
                        n652 = property on="EastSideView" class="Slide (strict)"("Value"=w1161) -> ()  [unwired: 2 in, 2 out]
                      }
                      frame "WestPosition" {
                        n653 = property on="WestSideView" class="Slide (strict)"("Value"=w1162) -> ()  [unwired: 2 in, 2 out]
                      }
                    }
                  }
                  frame True {
                    n654 = property class="Ctl"(reference=w1164, "Value"=w1163) -> ()  [unwired: 1 in, 2 out]
                  }
                }
              }
              frame "Stages" {
                (unwired) 0.0 ("Scale.Range:Minimum")
                n655 = Variant To Data(type=0, Variant=w1166) -> (data=w1165:i32)  [unwired: 1 in, 1 out]
                n656 = property on="EastSideView" class="Slide (strict)"("Scale.Maximum"=w1165) -> ()  [unwired: 2 in, 2 out]
                n657 = property on="WestSideView" class="Slide (strict)"("Scale.Maximum"=w1165) -> ()  [unwired: 2 in, 2 out]
                n658 = property on="WestPosition" class="DigNum (strict)"("Maximum"=w1165) -> ()  [unwired: 2 in, 2 out]
                n659 = property on="EastPosition" class="DigNum (strict)"("Maximum"=w1165) -> ()  [unwired: 2 in, 2 out]
              }
            }
          }
          event Menu Selection (User) {
            w1168 = "NTR\\NUTRITION"  # NTR Proce Name
            n660 = event-data() -> ("ItemTag"=w1171:string)  [unwired: 1 in]
            n661 = case shown="\"Nutrition:Terminate\"" w1171 {
              selector: w1171 -> [_ _ _ _ _ _ _ w1302 _ _]
              tunnel: w1170 -> [_ _ _ _ w1255 w1261 w1266 _ w1317 _]
              tunnel: [w1172 w1199 w1230 _ w1252 w1258 w1264 _ w1316 _] -> w1169
              tunnel: w1168 -> [_ _ _ _ w1251 w1257 w1265 _ _ _]
              frame "ConfigAux" {
                n662 = vi-ref "config-AUXI.vi"() -> (w1175:refnum<vi>)
                n663 = property class="VI"(reference=w1175) -> (reference out=w1174:refnum<vi>, error out=w1177:errorcluster, "Name"=w1176:string, "Exec.State"=w1173:T80)  [unwired: 1 in]
                n664 = case shown="\"Idle\"" w1173 {
                  tunnel: w1177 -> [w1192 _]
                  tunnel: w1176 -> [w1191 _]
                  tunnel: w1174 -> [_ w1198]
                  tunnel: [w1184 w1195] -> w1172
                  frame "Idle" {
                    n665 = call "variantCtrlIo.vi"("menu (Get Param)"=enumVarCtrlIO."IO List Configs") -> ("IO Configs List"=w1179:T42[])  [unwired: 6 in, 4 out]
                    n666 = call "io-find-by-type.vi"("Mode(Any)"=enum.io.mode."Mode", "Type"=enum.io.type."DO" ("type"), "IOConfigs in"=w1179) -> ("Search Results"=w1183:T42[])  [unwired: 8 in]
                    n667 = for {
                      tunnel: w1183 -> [w1194] mode=indexing
                      tunnel: [w1193] -> w1181 mode=indexing
                      workers-P: _ -> [_]
                      n668 = Unbundle By Name(w1194) -> ("Label"=w1193:string)
                    }
                    n669 = Open VI Reference(type specifier VI Refnum (for type only)=refnum<vi> refnum, vi path=w1191, options=128 ("call and forget"), error in (no error)=w1192) -> (vi reference=w1187:refnum<vi>, error out=w1188:errorcluster)  [unwired: 2 in]
                    n670 = call-by-ref "Start Asynchronous Call"(reference=w1187, error in=w1188, "DO List"=w1181) -> (reference out=w1190:refnum<vi>, error out=w1189:errorcluster)  [unwired: 11 in]
                    n671 = Close Reference(reference=w1190, error in (no error)=w1189) -> (error out=w1184:errorcluster)
                  }
                  frame Default {
                    n672 = invoke class="VI" method="FP.Open"(reference=w1198, "Activate"=TRUE ("Activate?"), "State"=T57."Standard") -> (error out=w1195:errorcluster)  [unwired: 2 in, 4 out]
                  }
                }
              }
              frame "ConfigController" {
                n673 = vi-ref "config-ICC.vi"() -> (w1202:refnum<vi>)
                n674 = property class="VI"(reference=w1202) -> (reference out=w1201:refnum<vi>, error out=w1204:errorcluster, "Name"=w1203:string, "Exec.State"=w1200:T80)  [unwired: 1 in]
                n675 = case shown="\"Idle\"" w1200 {
                  tunnel: w1204 -> [w1222 w1226]
                  tunnel: w1203 -> [w1221 _]
                  tunnel: w1201 -> [_ w1229]
                  tunnel: [w1209 w1225] -> w1199
                  frame "Idle" {
                    w1207 = enum.io.mode."Mode" ("Mode(Any)")
                    n676 = call "variantCtrlIo.vi"("menu (Get Param)"=enumVarCtrlIO."IO List Configs") -> ("IO Configs List"=w1205:T42[])  [unwired: 6 in, 4 out]
                    n677 = call "io-find-by-type.vi"("Mode(Any)"=w1207, "Type"=enum.io.type."DI" ("type"), "IOConfigs in"=w1205) -> ("Search Results"=w1210:T42[])  [unwired: 8 in]
                    n678 = call "io-find-by-type.vi"("Mode(Any)"=w1207, "Type"=enum.io.type."AI" ("type"), "IOConfigs in"=w1205) -> ("Search Results"=w1214:T42[])  [unwired: 8 in]
                    n679 = Build Array (concatenate)(w1214, w1210) -> (w1211:T42[])
                    n680 = for {
                      tunnel: w1211 -> [w1224] mode=indexing
                      tunnel: [w1223] -> w1208 mode=indexing
                      workers-P: _ -> [_]
                      n681 = Unbundle By Name(w1224) -> ("Label"=w1223:string)
                    }
                    n682 = Open VI Reference(type specifier VI Refnum (for type only)=refnum<vi> refnum, vi path=w1221, options=128 ("call and forget"), error in (no error)=w1222) -> (vi reference=w1217:refnum<vi>, error out=w1218:errorcluster)  [unwired: 2 in]
                    n683 = Sort 1D Array(array=w1208) -> ()  [unwired: 1 out]
                    n684 = call-by-ref "Start Asynchronous Call"(reference=w1217, error in=w1218) -> (reference out=w1220:refnum<vi>, error out=w1219:errorcluster)  [unwired: 12 in]
                    n685 = Close Reference(reference=w1220, error in (no error)=w1219) -> (error out=w1209:errorcluster)
                  }
                  frame Default {
                    n686 = invoke class="VI" method="FP.Open"(reference=w1229, error in=w1226, "Activate"=TRUE ("Activate?"), "State"=T57."Standard") -> (error out=w1225:errorcluster)  [unwired: 1 in, 4 out]
                  }
                }
              }
              frame "ConfigNutrition" {
                n687 = disable-structure shown="Disabled" {
                  frame Disabled {
                    n688 = call "config-NTR.vi"() -> ()  [unwired: 12 in]
                  }
                  frame Enabled {
                  }
                }
                n689 = vi-ref "config-NTR.vi"() -> (w1233:refnum<vi>)
                n690 = property class="VI"(reference=w1233) -> (reference out=w1232:refnum<vi>, error out=w1235:errorcluster, "Name"=w1234:string, "Exec.State"=w1231:T80)  [unwired: 1 in]
                n691 = case shown="\"Idle\"" w1231 {
                  tunnel: w1235 -> [w1244 w1246]
                  tunnel: w1234 -> [w1243 _]
                  tunnel: w1232 -> [_ w1249]
                  tunnel: [w1236 w1245] -> w1230
                  frame "Idle" {
                    n692 = Open VI Reference(type specifier VI Refnum (for type only)=refnum<vi> refnum, vi path=w1243, options=128 ("call and forget"), error in (no error)=w1244) -> (vi reference=w1239:refnum<vi>, error out=w1240:errorcluster)  [unwired: 2 in]
                    n693 = call-by-ref "Start Asynchronous Call"(reference=w1239, error in=w1240) -> (reference out=w1242:refnum<vi>, error out=w1241:errorcluster)  [unwired: 12 in]
                    n694 = Close Reference(reference=w1242, error in (no error)=w1241) -> (error out=w1236:errorcluster)
                  }
                  frame Default {
                    n695 = invoke class="VI" method="FP.Open"(reference=w1249, error in=w1246, "Activate"=TRUE ("Activate?"), "State"=T57."Standard") -> (error out=w1245:errorcluster)  [unwired: 1 in, 4 out]
                  }
                }
              }
              frame "IO_Configuration" {
                n696 = disable-structure shown="Disabled" {
                  frame Disabled {
                  }
                  frame Enabled {
                  }
                }
              }
              frame "Nutrition:Pause" {
                n697 = Bundle By Name(cluster=cluster{"cmd":T5, "data":variant} {"cmd"=enum."ENG.PROC.STOP", "data"=variant} ("typedefElement"), "data"=w1251) -> (w1253:cluster{"cmd":T5, "data":variant})
                n698 = Enqueue Element(queue=w1255, element=w1253) -> (error out=w1252:errorcluster)  [unwired: 2 in, 2 out]
                n699 = local write "NTR Status"("Paused" ("ntr.flow-status")) -> ()
              }
              frame "Nutrition:Start" {
                n700 = Bundle By Name(cluster=cluster{"cmd":T5, "data":variant} {"cmd"=enum."ENG.PROC.START", "data"=variant} ("typedefElement"), "data"=w1257) -> (w1259:cluster{"cmd":T5, "data":variant})
                n701 = Enqueue Element(queue=w1261, element=w1259) -> (error out=w1258:errorcluster)  [unwired: 2 in, 2 out]
                n702 = local write "NTR Status"("Starting..." ("ntr.flow-status")) -> ()
              }
              frame "Nutrition:Terminate" {
                n703 = Two Button Dialog(message="Terminate Nutrition Procedure?") -> (T button?=w1262:bool)  [unwired: 2 in]
                n704 = case shown="True" w1262 {
                  tunnel: w1266 -> [_ w1270]
                  tunnel: w1265 -> [_ w1271]
                  tunnel: [_ w1267] -> w1264
                  frame False {
                  }
                  frame True {
                    n705 = stacked-sequence {
                      tunnel: [w1278 _ _ _ _] -> w1275
                      tunnel: w1270 -> [w1277 _ w1284 w1288 w1297]
                      tunnel: [_ w1281 _ _ _] -> w1273
                      tunnel: [_ _ w1285 _ _] -> w1272
                      tunnel: w1271 -> [w1276 _ w1283 w1290 _]
                      tunnel: [_ _ _ w1289 _] -> w1269
                      tunnel: [_ _ _ _ w1296] -> w1268
                      frame #0 {
                        n706 = Bundle By Name(cluster=cluster{"cmd":T5, "data":variant} {"cmd"=enum."ENG.PROC.STOP", "data"=variant} ("typedefElement"), "data"=w1276) -> (w1279:cluster{"cmd":T5, "data":variant})
                        n707 = Enqueue Element(queue=w1277, element=w1279) -> (error out=w1278:errorcluster)  [unwired: 2 in, 2 out]
                      }
                      frame #1 {
                        n708 = global read "globals-engine.vi" "NutritionConfiguration"() -> (w1282:T64[])
                        n709 = call "ntr-init-io.vi"("NutritionConfiguration"=w1282) -> ("error out"=w1281:errorcluster)  [unwired: 10 in]
                      }
                      frame #2 {
                        n710 = Bundle By Name(cluster=cluster{"cmd":T5, "data":variant} {"cmd"=enum."ENG.PROC.RELOAD-BY-NAME", "data"=variant} ("typedefElement"), "data"=w1283) -> (w1287:cluster{"cmd":T5, "data":variant})
                        n711 = Enqueue Element(queue=w1284, element=w1287) -> (error out=w1285:errorcluster)  [unwired: 2 in, 2 out]
                      }
                      frame #3 {
                        n712 = Bundle By Name(cluster=cluster{"cmd":T5, "data":variant} {"cmd"=enum."ENG.PROC.STOP", "data"=variant} ("typedefElement"), "data"=w1290) -> (w1292:cluster{"cmd":T5, "data":variant})
                        n713 = Enqueue Element(queue=w1288, element=w1292) -> (error out=w1289:errorcluster)  [unwired: 2 in, 2 out]
                      }
                      frame #4 {
                        n714 = global read "globals-engine.vi" "Q-Log"() -> (w1294:refnum<queue>)
                        n715 = Bundle("Q-Log"=w1294, "procQ"=cluster{"data":variant, "Enum":T56} {"data"=variant, "Enum"=enum."LOG.INIT.NTR-FLOW"}) -> (w1293:T81)  [unwired: 1 in]
                        n716 = Bundle By Name(cluster=cluster{"cmd":T5, "data":variant} {"cmd"=enum."ENG.EXTERNAL-CALL", "data"=variant} ("typedefElement"), "data"=w1293) -> (w1299:cluster{"cmd":T5, "data":variant})
                        n717 = Enqueue Element(queue=w1297, element=w1299) -> (error out=w1296:errorcluster)  [unwired: 2 in, 2 out]
                      }
                    }
                    n718 = Merge Errors(w1275, w1273, w1272, w1269, w1268) -> (w1267:errorcluster)
                    n719 = local write "NTR Status"("Terminated" ("ntr.flow-status")) -> ()
                  }
                }
              }
              frame "PageAdmin", "PageIO", "PageMain" {
                n720 = case shown="\"PageAdmin\"" w1302 {
                  tunnel: ["MAIN" "I/O" "ADMIN"] -> w1301
                  frame "PageMain", Default {
                  }
                  frame "PageIO" {
                  }
                  frame "PageAdmin" {
                  }
                }
                n721 = property on="Tab Main" class="TabCtl (strict)"() -> ("Pages"=w1303:refnum<vi>[])  [unwired: 2 in, 2 out]
                n722 = for {
                  tunnel: w1303 -> [w1308] mode=indexing
                  tunnel: w1301 -> [w1306]
                  tunnel: [w1305] -> w1300
                  i -> [w1305]
                  stop <- w1304 stop-if-true
                  n723 = property class="Page"(reference=w1308) -> ("PageLabel"=w1307:string)  [unwired: 1 in, 2 out]
                  n724 = Equal?(x=w1307, y=w1306) -> (x = y?=w1304:bool)
                }
                n725 = local write "Tab Main"(w1300) -> ()
              }
              frame "Exit" {
                n726 = global read "globals-engine.vi" "NutritionConfiguration"() -> (w1312:T64[])
                n727 = property on="Stop" class="Bool (strict)"("Val(Sgnl)"=TRUE ("Value (Signaling)")) -> ()  [unwired: 2 in, 2 out]
                n728 = call "ntr-init-io.vi"("NutritionConfiguration"=w1312) -> ("error out"=w1313:errorcluster)  [unwired: 10 in]
                n729 = Enqueue Element(queue=w1317, element=cluster{"cmd":T5, "data":variant} {"cmd"=enum."ENG.EXIT", "data"=variant} ("typedefElement"), error in (no error)=w1313) -> (error out=w1316:errorcluster)  [unwired: 1 in, 2 out]
              }
              frame Default {
              }
            }
          }
          event Timeout; "Timer Reset?": Value Change {
            n730 = event-data() -> ()  [unwired: 1 in, 1 out]
            n731 = stacked-sequence {
              tunnel: [w1320 _ _ _] -> w1319
              tunnel: w1318 -> [_ _ w1377 w1403]
              frame #0 {
                n732 = expression code="x*1000"("TimerSec") -> (w1324:dbl)
                n733 = call "util-timer-inline.vi"("Reset?"="Timer Reset?", "Target[ms]"=w1324) -> ("done?"=w1329:bool, "downcount[sec]"=→"downcount[sec]":dbl)  [unwired: 6 in, 2 out]
                n734 = local read "Tab Main"() -> (w1328:enum32{"MAIN", "I/O", "ADMIN"})
                n735 = local write "Timer Reset?"(w1329) -> ()
                n736 = local read "Tab IO"() -> (w1327:enum32{"Map", "Editor", "Calibration"})
                n737 = call "util-ui-view.vi"("Page2"=w1327, "Page1"=w1328) -> ("Page1:Page2"=w1325:string)  [unwired: 7 in, 2 out]
                n738 = case shown="True" w1329 {
                  tunnel: [_ w1336] -> w1323
                  tunnel: w1325 -> [_ w1338]
                  tunnel: "IO Map Snapshot Enable" -> [_ w1337]
                  tunnel: [_ w1335] -> w1322
                  frame False {
                  }
                  frame True {
                    n739 = stacked-sequence {
                      tunnel: w1338 -> [w1341 _ _ _]
                      tunnel: w1337 -> [w1340 _ w1366 _]
                      tunnel: [w1339 _ _ _] -> w1336
                      tunnel: [_ w1356 _ _] -> w1335
                      frame #0 {
                        n740 = case shown="Default" w1341 {
                          tunnel: [_ w1343 w1346 w1355] -> w1339
                          tunnel: w1340 -> [_ w1342 _ _]
                          frame Default {
                          }
                          frame "I/O:Map" {
                            n741 = case shown="True" w1342 {
                              tunnel: [_ w1344] -> w1343
                              frame False {
                              }
                              frame True {
                                n742 = property on="IO Map Take Snapshot" class="Bool (strict)"("Val(Sgnl)"=TRUE ("Value (Signaling)")) -> (error out=w1344:errorcluster)  [unwired: 2 in, 1 out]
                              }
                            }
                          }
                          frame "I/O:Snapshot" {
                            n743 = disable-structure shown="Disabled" {
                              disable-tunnel: [w1352 _] -> w1346
                              frame Disabled {
                                w1350 = cluster{"cmd":T5, "data":variant} {"cmd"=enum."ENG.RIO.SNAPSHOT", "data"=variant}  # snapshot all
                                n744 = local read item#-1() -> (w1348)
                                n745 = Build Array(w1348) -> (w1347:void[])
                                n746 = global read "globals-engine.vi" "Q-Eng"() -> (w1351:refnum<queue>)
                                n747 = Bundle By Name(cluster=w1350, "data"=w1347) -> (w1349:cluster{"cmd":T5, "data":variant})
                                n748 = Enqueue Element(queue=w1351, element=w1349) -> (error out=w1352:errorcluster)  [unwired: 2 in, 2 out]
                              }
                              frame Enabled {
                              }
                            }
                          }
                          frame "I/O:Calibration" {
                            n749 = global read "globals-engine.vi" "Q-Eng"() -> (w1354:refnum<queue>)
                            n750 = Enqueue Element(queue=w1354, element=cluster{"cmd":T5, "data":variant} {"cmd"=enum."ENG.RIO.AIN-SNAPSHOT-CALIB", "data"=variant} ("typedefElement")) -> (error out=w1355:errorcluster)  [unwired: 2 in, 2 out]
                          }
                        }
                      }
                      frame #1 {
                        n751 = global read "globals-engine.vi" "Q-Com"() -> (w1359:refnum<queue>)
                        n752 = Get Queue Status(queue=w1359) -> (error out=w1357:errorcluster, # elements in queue=→"COM FIFO":i32)  [unwired: 2 in, 6 out]
                        n753 = global read "globals-engine.vi" "Q-Log"() -> (w1364:refnum<queue>)
                        n754 = global read "globals-engine.vi" "Q-Eng"() -> (w1362:refnum<queue>)
                        n755 = Get Queue Status(queue=w1364) -> (error out=w1361:errorcluster, # elements in queue=→"LOG FIFO 2":i32)  [unwired: 2 in, 6 out]
                        n756 = Get Queue Status(queue=w1362) -> (error out=w1360:errorcluster, # elements in queue=→"ENG FIFO 2":i32)  [unwired: 2 in, 6 out]
                        n757 = Merge Errors(w1357, w1361, w1360) -> (w1356:errorcluster)
                      }
                      frame #2 {
                        n758 = case shown="False" w1366 {
                          frame False {
                          }
                          frame True {
                            n759 = property on="IO Map Take Snapshot" class="Bool (strict)"("Val(Sgnl)"=TRUE ("Value (Signaling)")) -> ()  [unwired: 2 in, 2 out]
                          }
                        }
                      }
                      frame #3 {
                        n760 = global read "globals-engine.vi" "Q-Log"() -> (w1370:refnum<queue>)
                        n761 = Enqueue Element(queue=w1370, element=cluster{"data":variant, "Enum":T56} {"data"=variant, "Enum"=enum."LOG.UPDATE.IRR"} ("procQ")) -> (error out=w1369:errorcluster)  [unwired: 2 in, 2 out]
                        n762 = call <vilib>:"Clear Errors.vi"("error in (no error)"=w1369) -> ()  [unwired: 5 in, 2 out]
                      }
                    }
                  }
                }
                n763 = Merge Errors(w1323, w1322) -> (w1321:errorcluster)
                n764 = flat-sequence {
                  tunnel: [w1333] -> w1320
                  tunnel: w1321 -> [w1333]
                  frame #0 {
                    n765 = property on="Timer Reset?" class="Bool (strict)"("Value"=FALSE ("Timer Reset?")) -> ()  [unwired: 2 in, 2 out]
                  }
                }
              }
              frame #1 {
                n766 = case shown="False" FALSE {
                  frame False {
                  }
                  frame True {
                    n767 = Unbundle By Name("VISA REPORT") -> ("VISA Report En"=w1373:bool)
                    n768 = case shown="True" w1373 {
                      tunnel: "VISA REPORT" -> [_ w1374]
                      frame False {
                      }
                      frame True {
                        n769 = call "helper-log-visa.vi"("VISA REPORT"=w1374) -> ("array type (2D Dbl)"=w1375:string[][])  [unwired: 9 in, 1 out]
                        n770 = property on="visa report" class="Tbl (strict)"("Value"=w1375) -> ()  [unwired: 2 in, 2 out]
                      }
                    }
                  }
                }
              }
              frame #2 {
                w1378 = "%d/%m/%y" ("time format string (%c)")
                # "PBR"
                n771 = local read "last"() -> (w1380:T17)
                n772 = Format Date/Time String(time format string (%c)=w1378, seconds (now)=w1380) -> (date/time string=w1379:string)  [unwired: 1 in]
                n773 = Format Date/Time String(time format string (%c)=w1378, seconds (now)=w1377) -> (date/time string=w1381:string)  [unwired: 1 in]
                n774 = Not Equal?(x=w1379, y=w1381) -> (x != y?=w1376:bool)
                n775 = First Call?() -> (First Call?: T/F=w1382:bool)
                n776 = feedback #3(TRUE ("Found?")) -> (w1385:bool)
                n777 = Select(t=FALSE ("Found?"), s=w1376, f=w1385) -> (s? t:f=w1386:bool)
                n778 = Or(x=w1386, y=w1382) -> (x .or. y?=w1383:bool)
                n779 = case shown="False" w1383 {
                  selector: w1383 -> [_ w1401]
                  tunnel: [w1391 w1401] -> w1384
                  tunnel: w1377 -> [w1390 _]
                  frame False {
                    n780 = Add(x="start", y=60.0) -> (x+y=w1396:T17)
                    n781 = Bundle By Name(cluster=cluster{"start":T17, "stop":T17} {"start"=timestamp(0 s since 1904-01-01), "stop"=timestamp(0 s since 1904-01-01)} ("sched-pairs"), "start"="start", "stop"=w1396) -> (w1397:cluster{"start":T17, "stop":T17})
                    n782 = Build Array(w1397) -> (w1398:cluster{"start":T17, "stop":T17}[])
                    n783 = call "sched-check-compare.vi"("sched-mode"=enum16{"Hourly", "Daily", "Weekly", "Date"}."Daily", "sched-pairs"=w1398, "time stamp"=w1390) -> ("Time"=w1389:timestamp, "Found?"=w1391:bool)  [unwired: 5 in, 2 out]
                    n784 = case shown="False" w1391 {
                      selector: w1391 -> [_ w1399]
                      tunnel: w1389 -> [_ _]
                      frame False {
                      }
                      frame True {
                        n785 = disable-structure shown="Disabled" {
                          disable-tunnel: w1399 -> [_ _]
                          frame Disabled {
                            n786 = call-poly <vilib>:"Write Delimited Spreadsheet.vi"("append to file? (new file:F)"=TRUE) -> ()  [unwired: 13 in, 2 out]
                          }
                          frame Enabled {
                          }
                        }
                        n787 = property on="Harvest" class="Bool (strict)"("Val(Sgnl)"=w1399) -> ()  [unwired: 2 in, 2 out]
                      }
                    }
                  }
                  frame True {
                  }
                }
                n788 = feedback-in #3(w1384) -> ()
              }
              frame #3 {
                # "sun/moon indicator"
                n789 = call "irr-sunrise-calc.vi"("Time Stamp"=w1403) -> ("(T) Day (F) Night"=→"DayNight":bool)  [unwired: 7 in, 3 out]
              }
            }
          }
          event "UVAccHistoryDays", "UvAccRefresh": Value Change {
            n790 = event-data() -> ()  [unwired: 1 in, 1 out]
            n791 = call "helper-build-graph.vi"("Row(2)"=1, "Module (OCS)"="IRR\\db", "filename.*"="_UV_ACC_*.rec", "lastDays"="UVAccHistoryDays") -> ("error out"=w1406:errorcluster, "Multiple Plots (X Array and Y Array)"=→"UV_ACC":cluster{"X":dbl[], "Y":dbl[]})  [unwired: 5 in, 1 out]
            n792 = call <vilib>:"Clear Errors.vi"("error in (no error)"=w1406) -> ("error out"=w1404:errorcluster)  [unwired: 5 in, 1 out]
          }
          event "RFS SetX1": Value Change {
            n793 = event-data() -> ()  [unwired: 1 in, 1 out]
            n794 = global read "globals-engine.vi" "Q-Eng"() -> (w1412:refnum<queue>)
            n795 = Enqueue Element(queue=w1412, element=cluster{"cmd":T5, "data":variant} {"cmd"=enum."ENG.RIO.RFS-DELAY-SET-X1", "data"=variant} ("typedefElement")) -> (error out=w1411:errorcluster)  [unwired: 2 in, 2 out]
          }
          event "RFS SetX8": Value Change {
            n796 = event-data() -> ()  [unwired: 1 in, 1 out]
            n797 = global read "globals-engine.vi" "Q-Eng"() -> (w1415:refnum<queue>)
            n798 = Enqueue Element(queue=w1415, element=cluster{"cmd":T5, "data":variant} {"cmd"=enum."ENG.RIO.RFS-DELAY-SET-X8", "data"=variant} ("typedefElement")) -> (error out=w1414:errorcluster)  [unwired: 2 in, 2 out]
          }
          event "RFS Cycles Set": Value Change {
            n799 = event-data() -> ()  [unwired: 1 in, 1 out]
            n800 = global read "globals-engine.vi" "Q-Eng"() -> (w1418:refnum<queue>)
            n801 = Enqueue Element(queue=w1418, element=cluster{"cmd":T5, "data":variant} {"cmd"=enum."ENG.RIO.RFS-CYCLES-SET", "data"=variant} ("typedefElement")) -> (error out=w1417:errorcluster)  [unwired: 2 in, 2 out]
          }
          event "RFS Cycles Get": Value Change {
            n802 = event-data() -> ()  [unwired: 1 in, 1 out]
            n803 = global read "globals-engine.vi" "Q-Eng"() -> (w1421:refnum<queue>)
            n804 = Enqueue Element(queue=w1421, element=cluster{"cmd":T5, "data":variant} {"cmd"=enum."ENG.RIO.RFS-CYCLES-GET", "data"=variant} ("typedefElement")) -> (error out=w1420:errorcluster)  [unwired: 2 in, 2 out]
          }
          event "RFS Enable Table": Value Change {
            n805 = event-data() -> ()  [unwired: 1 in, 1 out]
            n806 = global read "globals-engine.vi" "Q-Eng"() -> (w1424:refnum<queue>)
            n807 = Enqueue Element(queue=w1424, element=cluster{"cmd":T5, "data":variant} {"cmd"=enum."ENG.RIO.RFS-ENABLE", "data"=variant} ("typedefElement")) -> (error out=w1423:errorcluster)  [unwired: 2 in, 2 out]
          }
          event "EngLogClear": Value Change {
            n808 = event-data() -> ()  [unwired: 1 in, 1 out]
            n809 = call "reg-eng-calls.vi"("Operation(Read)"=enum.report-filter."ClearAll") -> ("error out"=w1426:errorcluster, "Collected Reports"=w1427:string)  [unwired: 9 in]
            n810 = local write "Collected Reports"(w1427) -> ()
          }
        }
        n811 = case shown="\"\"" w126 {
          selector: w126 -> [_ w132]
          frame "" {
            # "skip empty statuts"
          }
          frame Default {
            # "status register"
            n812 = call "reg-status.vi"("Operation(Read)"=enum.report-filter."Collect", "Reports to Collect"=w132) -> ("Collected Reports"=w134:string)  [unwired: 8 in, 1 out]
            n813 = local write "User messages"(w134) -> ()
          }
        }
        n814 = call <vilib>:"Simple Error Handler.vi"("type of dialog (OK msg:1)"=w127, "error in (no error)"=w130) -> ()  [unwired: 3 in, 5 out]
        "Event" <- w128
      }
    }
  }
  n815 = while "GUI MONITOR" {
    tunnel: w21 -> [w1435]
    tunnel: w24 -> [w1437]
    tunnel: w25 -> [w1436]
    shift-right: [w1430] -> _
    shift-left: errorcluster[] [] ("Array out") -> [w1431]
    i -> [w1432]
    stop <- w1441 stop-if-true
    # "TODO make a general \nerror message \nvi eng vs log"
    n816 = Get Date/Time In Seconds() -> (seconds since 1Jan1904=w1433:timestamp)
    n817 = Dequeue Element(queue=w1435, timeout in ms (-1)=-1, error in (no error)=w1437) -> (queue out=w1440:refnum<queue>, element=w1442:cluster{"data":variant, "Enum":T56}, timed out?=w1439:bool, error out=w1443:errorcluster)
    n818 = case shown="No Error" w1443 {
      selector: w1443 -> [_ w1745]
      tunnel: w1442 -> [w1452 _]
      tunnel: [w1449 _] -> w1441
      tunnel: w1440 -> [w1453 _]
      tunnel: w1439 -> [w1451 _]
      tunnel: [w1450 w1745] -> w1429
      tunnel: w1436 -> [w1448 _]
      tunnel: [w1447 _] -> w1434
      tunnel: w1433 -> [_ _]
      frame No Error {
        n819 = case shown="False" w1451 {
          tunnel: w1453 -> [_ w1462]
          tunnel: w1452 -> [_ w1460]
          tunnel: [_ w1456] -> w1450
          tunnel: [_ w1461] -> w1449
          tunnel: w1448 -> [_ w1458]
          tunnel: [_ w1457] -> w1447
          frame True {
            # "Queue Timeout"
          }
          frame False {
            # "Command Handler"
            n820 = Unbundle(w1460) -> ("data"=w1459:variant, "Enum"=w1454:T56)
            n821 = case shown="\"LOG.CATCH\"" w1454 {
              tunnel: w1462 -> [_ w1539 _ _ _ _ _ _ _ _]
              tunnel: [w1472 w1537 _ w1544 _ _ w1626 w1643 w1671 _] -> w1456
              tunnel: [_ TRUE _ _ _ _ _ _ _ _] -> w1461
              tunnel: w1459 -> [w1475 _ _ _ _ w1554 w1627 w1644 _ _]
              tunnel: w1458 -> [_ _ _ _ _ _ _ _ _ _]
              tunnel: [_ _ _ _ _ _ _ _ "Update Irrigation parameters" _] -> w1457
              frame "LOG.CATCH" {
                n822 = Variant To Data(type=T82 {"Procedure(post)"=[], "Procedure(pre)"=[], "Next State "={"CMD"=enum."NEXT", "data"=variant}, "IsRunning"=FALSE, "error in"={"status"=FALSE, "code"=0, "source"=""}} ("cluster"), Variant=w1475) -> (data=w1473:T82)  [unwired: 1 in, 1 out]
                n823 = Unbundle By Name(w1473) -> ("Procedure(post)"=w1471:variant[], "Procedure(pre)"=w1470:variant[], "Next State"=w1469:cluster{"CMD":T83, "data":variant}, "IsRunning"=w1468:bool, "error in"=w1463:errorcluster)
                n824 = call "engine.logger.vi"("isRunning"=w1468, "Proc Error"=w1463, "Next State in"=w1469, "Procedure(pre)"=w1470, "Procedure(post) in"=w1471) -> ("error IO"=w1467:errorcluster, "output cluster"=w1466:T84)  [unwired: 4 in, 1 out]
                n825 = stacked-sequence {
                  tunnel: w1466 -> [w1480 w1493]
                  tunnel: [w1478 _] -> w1465
                  tunnel: [_ w1492] -> w1464
                  frame #0 {
                    # "Catch ANY log"
                    n826 = local read "Admin Panel"() -> (w1476:bool)
                    n827 = call "reg-log-general.vi"("Operation(Read)"=enum.report-filter."Collect", "filter by proc name"="Proc Name", "Reports to Collect"=w1480) -> ("error out"=w1479:errorcluster)  [unwired: 6 in, 2 out]
                    n828 = case shown="True" w1476 {
                      tunnel: w1479 -> [_ w1487]
                      tunnel: [_ w1486] -> w1478
                      tunnel: "Proc Name" -> [_ w1484]
                      frame False {
                      }
                      frame True {
                        n829 = call "reg-log-general.vi"("Operation(Read)"=enum.report-filter."Read ALL", "error in"=w1487, "filter by proc name"=w1484) -> ("error out"=w1486:errorcluster, "compact report"=w1483:T77[])  [unwired: 6 in, 1 out]
                        n830 = case shown="True" "Enable Report" {
                          tunnel: w1483 -> [_ w1488]
                          frame False {
                          }
                          frame True {
                            "Report General" <- w1488
                          }
                        }
                      }
                    }
                  }
                  frame #1 {
                    # "Catch APP log (AUXI, IRR, NTR ... )"
                    n831 = Unbundle By Name(w1493) -> ("Proc Module"=w1491:string, "Step Function"=w1489:T6)
                    n832 = case "Catch by module name (OCS,AUXI,IRR,NTR,...)" shown="\"IRR\"" w1491 {
                      selector: w1491 -> [_ _ w1504 _ _]
                      tunnel: w1493 -> [_ w1498 w1506 w1517 w1525]
                      tunnel: [_ _ w1505 _ _] -> w1492
                      tunnel: "LOG.PARSE." -> [_ _ w1503 _ _]
                      tunnel: w1489 -> [_ _ w1502 _ _]
                      frame Default {
                      }
                      frame "AUXI" {
                        n833 = local read "Tab Main"() -> (w1497:enum32{"MAIN", "I/O", "ADMIN"})
                        n834 = local read "Tab Auxi"() -> (w1496:T30)
                        n835 = Format Into String(format string="%s_%s", w1497, w1496) -> (resulting string=w1495:string)  [unwired: 2 in, 1 out]
                        n836 = case shown="\"MAIN_Auxiliary\"" w1495 {
                          tunnel: w1498 -> [_ w1499]
                          frame Default {
                          }
                          frame "MAIN_Auxiliary" {
                            n837 = local read "AuxiliaryList"() -> (w1500:T33)
                            n838 = call "helper-log-parse-auxi.vi"("log cluster"=w1499, "AuxiliaryList in"=w1500) -> ("AuxiliaryList out"=w1501:T33)  [unwired: 9 in]
                            n839 = local write "AuxiliaryList"(w1501) -> ()
                          }
                        }
                      }
                      frame "OCS" {
                        n840 = case shown="\"_OCS_CHECK\", \"_OCS_RECORD\"" w1502 {
                          tunnel: w1506 -> [_ w1514]
                          tunnel: [_ w1513] -> w1505
                          tunnel: w1504 -> [_ w1512]
                          tunnel: w1503 -> [_ w1510]
                          frame Default {
                          }
                          frame "_OCS_CHECK", "_OCS_RECORD" {
                            n841 = Concatenate Strings(w1510, w1512) -> (w1509:string)
                            n842 = Scan From String(input string=w1509, default 1=state-logger."LOG.NO_OP" ("Enum")) -> (output 1=w1508:T56)  [unwired: 3 in, 3 out]
                            n843 = global read "globals-engine.vi" "Q-Log"() -> (w1515:refnum<queue>)
                            n844 = Bundle By Name(cluster=cluster{"data":variant, "Enum":T56} {"data"=variant, "Enum"=enum."LOG.NO_OP"} ("procQ"), "Enum"=w1508, "data"=w1514) -> (w1516:cluster{"data":variant, "Enum":T56})
                            n845 = Enqueue Element(queue=w1515, element=w1516) -> (error out=w1513:errorcluster)  [unwired: 2 in, 2 out]
                          }
                        }
                      }
                      frame "IRR" {
                        n846 = call "helper-log-parse-irr.vi"("output cluster"=w1517) -> ("Cluster"=w1519:cluster{"sample":dbl, "UV Limit":dbl}, "update chart?"=w1518:bool)  [unwired: 9 in]
                        n847 = case shown="True" w1518 {
                          tunnel: w1519 -> [_ w1524]
                          frame False {
                          }
                          frame True {
                            n848 = global read "globals-engine.vi" "IRR Params"() -> (w1520:T31)
                            n849 = Unbundle By Name(w1524) -> ("sample"=→"UV Acc.":dbl)
                            n850 = Unbundle By Name(w1520) -> ("Last Iteration"=w1521:timestamp, "UV Reduction Status"=w1522:bool)
                            n851 = property on="UV Reduction Status" class="Bool (strict)"("Value"=w1522) -> ()  [unwired: 2 in, 2 out]
                            n852 = property on="Last Iteration" class="AbsTime (strict)"("Value"=w1521) -> ()  [unwired: 2 in, 2 out]
                            "Waveform Chart 2" <- w1524
                          }
                        }
                      }
                      frame "NTR" {
                        n853 = stacked-sequence {
                          tunnel: w1525 -> [w1527 w1533]
                          frame #0 {
                            n854 = property on="NTR Flowchart" class="Clust (strict)"() -> ("Controls[]"=w1526:refnum<vi>[])  [unwired: 2 in, 2 out]
                            n855 = call "ntr.flow-panel.update.vi"("log cluster"=w1527, "Controls[]"=w1526) -> ()  [unwired: 10 in]
                            n856 = call "helper-log-parse-ntr.vi"("output cluster"=w1527) -> ("NTR Status"=w1529:string, "update?"=w1528:bool)  [unwired: 9 in]
                            n857 = case shown="True" w1528 {
                              tunnel: w1529 -> [_ w1530]
                              frame False {
                              }
                              frame True {
                                "NTR Status" <- w1530
                              }
                            }
                          }
                          frame #1 {
                            n858 = Unbundle By Name(w1533) -> ("Step Function"=w1532:T6)
                            n859 = control-ref of="ntr.status-table"() -> (w1531:refnum<vi>)
                            n860 = case shown="\"UNIT_SAMPLE\"" w1532 {
                              tunnel: w1531 -> [_ w1536]
                              tunnel: w1533 -> [_ w1535]
                              frame Default {
                              }
                              frame "UNIT_SAMPLE" {
                                n861 = call "ntr.log-parse.unit-sample.vi"("log"=w1535, "status-table-REF"=w1536) -> ("ntr.status-table"=→"ntr.status-table":string[][])  [unwired: 9 in]
                              }
                            }
                          }
                        }
                      }
                    }
                  }
                }
                n862 = Merge Errors(w1467, w1465, w1464) -> (w1472:errorcluster)
              }
              frame "LOG.EXIT" {
                # "\"ENG.EXIT\""
                n863 = Release Queue(queue=w1539) -> (error out=w1538:errorcluster)  [unwired: 2 in, 2 out]
                n864 = Merge Errors(w1538) -> (w1537:errorcluster)
              }
              frame "LOG.INIT" {
                # "\"LOG.INIT\"\nSET GUI INDICATORS TO INITIAL STATE"
                n865 = invoke on="MenuRuntime" class="Clust (strict)" method="Reinit To Default"() -> ()  [unwired: 3 in, 3 out]
                n866 = property on="Waveform Chart" class="WFChart (strict)"("History Data"=u32[] []) -> ()  [unwired: 2 in, 2 out]
                n867 = property on="NTR Flowchart" class="Clust (strict)"() -> ("Controls[]"=w1543:refnum<vi>[])  [unwired: 2 in, 2 out]
                n868 = call "ntr.flow-panel.init.vi"("Controls in"=w1543) -> ()  [unwired: 8 in, 3 out]
                n869 = local write "NTR Status"("Initial" ("NTR Status")) -> ()
              }
              frame "LOG.INIT.NTR-FLOW" {
                n870 = property on="NTR Flowchart" class="Clust (strict)"() -> ("Controls[]"=w1546:refnum<vi>[])  [unwired: 2 in, 2 out]
                n871 = local write "NTR Status"("Initial" ("NTR Status")) -> ()
                n872 = call "ntr.flow-panel.init.vi"("Controls in"=w1546) -> ("error in (no error)"=w1544:errorcluster)  [unwired: 8 in, 2 out]
              }
              frame "LOG.NO_OP", Default {
              }
              frame "LOG.PARSE.OCS" {
                # "\"LOG.PARSE.OCS\" \nPARSE Outdoor Climate Sampling module LOG"
                n873 = Variant To Data(type=T84 {"Proc Name"="", "ProcPath"="", "Step Name"="", "Step Function"=enum."__NO-OP", "Step Index"=0, "Report"="", "clk"=0.0, "error in"={"status"=FALSE, "code"=0, "source"=""}, "Log Message"="", "Proc Module"=""} ("output cluster"), Variant=w1554) -> (data=w1552:T84)  [unwired: 1 in, 1 out]
                n874 = Unbundle By Name(w1552) -> ("Proc Name"=w1548:string, "Step Function"=w1551:T6, "Report"=w1550:string)
                n875 = Search and Replace String(input string=w1548, search string="OCS\\") -> (result string=w1547:string)  [unwired: 6 in, 3 out]
                n876 = case "Switch(Proc Name)" shown="\"OCS\"" w1547 {
                  tunnel: w1551 -> [_ w1556 w1562 w1569 w1577 w1621]
                  tunnel: w1550 -> [_ w1555 w1561 w1568 w1576 w1620]
                  frame Default {
                  }
                  frame "GET-UV" {
                    n877 = case shown="\"_IO_READ\"" w1556 {
                      tunnel: w1555 -> [w1559 _]
                      frame "_IO_READ" {
                        n878 = Match Pattern(string=w1559, regular expression="=") -> (after substring=w1557:string)  [unwired: 1 in, 3 out]
                        n879 = Fract/Exp String To Number(string=w1557) -> ()  [unwired: 3 in, 2 out]
                      }
                      frame Default {
                      }
                    }
                  }
                  frame "GET-WD" {
                    n880 = call "util.DelimitedStringToArray.vi"("delimitaed string"=w1561) -> ("array out"=w1560:string[])  [unwired: 10 in]
                    n881 = case shown="\"_GET_WD\"" w1562 {
                      tunnel: w1561 -> [w1565 _]
                      tunnel: w1560 -> [_ _]
                      frame "_GET_WD" {
                        n882 = call "util.DelimitedStringToArray.vi"("delimitaed string"=w1565) -> ("array out"=w1564:string[])  [unwired: 10 in]
                        n883 = Index Array(array=w1564) -> (element=w1563:string)  [unwired: 1 in]
                        n884 = Match Pattern(string=w1563, regular expression="=") -> ()  [unwired: 1 in, 4 out]
                      }
                      frame Default {
                      }
                    }
                  }
                  frame "GET-WS" {
                    n885 = call "util.DelimitedStringToArray.vi"("delimitaed string"=w1568) -> ("array out"=w1567:string[])  [unwired: 10 in]
                    n886 = case shown="\"_GET_WS\"" w1569 {
                      tunnel: w1568 -> [w1573 _]
                      tunnel: w1567 -> [_ _]
                      frame "_GET_WS" {
                        n887 = call "util.DelimitedStringToArray.vi"("delimitaed string"=w1573) -> ("array out"=w1572:string[])  [unwired: 10 in]
                        n888 = Index Array(array=w1572) -> (element=w1571:string)  [unwired: 1 in]
                        n889 = Match Pattern(string=w1571, regular expression="=") -> (after substring=w1570:string)  [unwired: 1 in, 3 out]
                        n890 = Fract/Exp String To Number(string=w1570) -> ()  [unwired: 3 in, 2 out]
                      }
                      frame Default {
                      }
                    }
                  }
                  frame "OCS" {
                    n891 = call "util.DelimitedStringToArray.vi"("delimitaed string"=w1576) -> ("array out"=w1575:string[])  [unwired: 10 in]
                    n892 = case "Switch (Step Name)" shown="\"_OCS_CHECK\"" w1577 {
                      tunnel: w1576 -> [_ _]
                      tunnel: w1575 -> [w1578 _]
                      frame "_OCS_CHECK" {
                        n893 = stacked-sequence {
                          tunnel: w1578 -> [w1580 w1605]
                          frame #0 {
                            # "parse outdoor sensors (TDRY, TWET ...)"
                            n894 = for {
                              tunnel: w1580 -> [w1593] mode=indexing
                              tunnel: [w1581] -> w1579 mode=indexing
                              n895 = Match Pattern(string=w1593, regular expression="=") -> (before substring=w1588:string, after substring=w1590:string)  [unwired: 1 in, 2 out]
                              n896 = Concatenate Strings(w1588, "_BUF" ("string")) -> (w1583:string)
                              n897 = Decimal String To Number(string=w1590) -> (number=w1591:i32)  [unwired: 2 in, 1 out]
                              n898 = call "variantCtrlIo.vi"("menu (Get Param)"=enumVarCtrlIO."IO Get By Key", "Key (use IOnode Label if empty )"=w1583) -> ("error out"=w1584:errorcluster, "IOnode out"=w1585:T42)  [unwired: 5 in, 3 out]
                              n899 = Number To Decimal String(number=w1591) -> (decimal integer string=w1589:string)  [unwired: 1 in]
                              n900 = call <vilib>:"Clear Errors.vi"("error in (no error)"=w1584) -> ()  [unwired: 5 in, 2 out]
                              n901 = Unbundle By Name(w1585) -> ("Value"=w1582:string)
                              n902 = case shown="\"_H0_RH\"" w1588 {
                                tunnel: w1593 -> [_ _ _ _ _ _ _]
                                tunnel: w1589 -> [_ w1594 w1595 w1596 w1597 w1598 w1599]
                                tunnel: w1582 -> [_ _ _ _ _ _ _]
                                frame Default {
                                }
                                frame "H0_TDRY" {
                                n903 = property on="Tdry" class="Str"("Value"=w1594) -> ()  [unwired: 2 in, 2 out]
                                }
                                frame "H0_TWET" {
                                n904 = property on="Twet" class="Str"("Value"=w1595) -> ()  [unwired: 2 in, 2 out]
                                }
                                frame "_H0_RH" {
                                n905 = property on="Humidity" class="Str"("Value"=w1596) -> ()  [unwired: 2 in, 2 out]
                                }
                                frame "H0_UV" {
                                n906 = property on="UV" class="Str"("Value"=w1597) -> ()  [unwired: 2 in, 2 out]
                                }
                                frame "H0_WSPD" {
                                n907 = property on="Wind Speed" class="Str"("Value"=w1598) -> ()  [unwired: 2 in, 2 out]
                                n908 = property on="Wind Speed" class="Str"("Value"=w1598) -> ()  [unwired: 2 in, 2 out]
                                }
                                frame "H0_WDIR" {
                                n909 = Decimal String To Number(string=w1599) -> (number=w1603:i32)  [unwired: 2 in, 1 out]
                                n910 = call "wind-dir-calc.vi"("Analog Direction"=w1603) -> ("Ndir"=w1600:T86, "Wind Dir View"=→"Wind Dir Panel":T29)  [unwired: 9 in]
                                n911 = call "helper-wind-status.vi"("Ndir"=w1600) -> ("Value"=w1601:string)  [unwired: 10 in]
                                n912 = property on="Wind Direction" class="Str"("Value"=w1599) -> ()  [unwired: 2 in, 2 out]
                                n913 = property on="Wind Direction" class="Str"("Value"=w1601) -> ()  [unwired: 2 in, 2 out]
                                }
                              }
                              n914 = Bundle(w1583, "Value"=w1582) -> (w1581:cluster{string, "Value":string})  [unwired: 1 in]
                            }
                            "Array 2" <- w1579
                          }
                          frame #1 {
                            # "parse indoor sensors (H1_TDRY, H1_TWET ...)"
                            n915 = local read "Section"() -> (w1604:string)
                            n916 = for {
                              tunnel: w1605 -> [w1612] mode=indexing
                              tunnel: w1604 -> [w1615]
                              n917 = Format Into String(format string="%s_" ("_H1_"), w1615) -> (resulting string=w1610:string)  [unwired: 2 in, 1 out]
                              n918 = Match Pattern(string=w1612, regular expression="=") -> (before substring=w1611:string, after substring=w1607:string)  [unwired: 1 in, 2 out]
                              n919 = Match Pattern(string=w1611, regular expression=w1610) -> (after substring=w1609:string)  [unwired: 1 in, 3 out]
                              n920 = Decimal String To Number(string=w1607) -> (number=w1608:i32)  [unwired: 2 in, 1 out]
                              n921 = Number To Decimal String(number=w1608) -> (decimal integer string=w1606:string)  [unwired: 1 in]
                              n922 = case shown="\"TDRY\"" w1609 {
                                tunnel: w1606 -> [_ w1616 w1617 w1618]
                                frame Default {
                                }
                                frame "TDRY" {
                                n923 = property on="Tdry" class="Str"("Value"=w1616) -> ()  [unwired: 2 in, 2 out]
                                }
                                frame "TWET" {
                                n924 = property on="Twet" class="Str"("Value"=w1617) -> ()  [unwired: 2 in, 2 out]
                                }
                                frame "RH" {
                                n925 = property on="Humidity" class="Str"("Value"=w1618) -> ()  [unwired: 2 in, 2 out]
                                }
                              }
                            }
                          }
                        }
                      }
                      frame Default {
                      }
                    }
                  }
                  frame "OCS_RECORD" {
                    n926 = call "util.DelimitedStringToArray.vi"("delimitaed string"=w1620) -> ("array out"=w1619:string[])  [unwired: 10 in]
                    n927 = case "Switch (Step Name)" shown="\"_OCS_RECORD\"" w1621 {
                      tunnel: w1620 -> [_ _]
                      tunnel: w1619 -> [_ _]
                      frame Default {
                      }
                      frame "_OCS_RECORD" {
                        n928 = property on="refresh" class="Bool (strict)"("Val(Sgnl)"=TRUE ("Value (Signaling)")) -> ()  [unwired: 2 in, 2 out]
                      }
                    }
                  }
                }
              }
              frame "LOG.SNAPSHOT" {
                # "\"LOG.UPDATE.SNAPSHOT\" (Snapshot)"
                n929 = local read "Tab Main"() -> (w1625:enum32{"MAIN", "I/O", "ADMIN"})
                n930 = local read "Tab IO"() -> (w1624:enum32{"Map", "Editor", "Calibration"})
                n931 = call "util-ui-view.vi"("Page2"=w1624, "Page1"=w1625) -> ("Page1:Page2"=w1623:string)  [unwired: 7 in, 2 out]
                n932 = case shown="\"I/O:Map\"" w1623 {
                  tunnel: w1627 -> [_ w1640]
                  tunnel: [_ w1639] -> w1626
                  frame "False", Default {
                  }
                  frame "I/O:Map" {
                    n933 = Variant To Data(type=T13[] [{"Address"=0, "DI"=[], "status"={"status"=TRUE, "code"=-1073807339, "source"="Failed to read IO: "}, "AI"=[0.0], "Dports"=0, "AI RAW"=[]}, {"Address"=1, "DI"=[], "status"={"status"=TRUE, "code"=-1073807339, "source"="Failed to read IO: "}, "AI"=[0.0], "Dports"=0, "AI RAW"=[]}, {"Address"=2, "DI"=[FALSE, FALSE, FALSE, FALSE, FALSE, FALSE, FALSE, TRUE, FALSE, FALSE, FALSE, FALSE, FALSE, FALSE, FALSE, FALSE, FALSE, FALSE, TRUE, FALSE, FALSE, FALSE, FALSE, FALSE, FALSE, TRUE, FALSE, FALSE, FALSE, FALSE, FALSE, FALSE, TRUE, TRUE, TRUE, TRUE, TRUE, TRUE, FALSE, TRUE], "status"={"status"=FALSE, "code"=0, "source"=""}, "AI"=[-39.53601953601954, 0.0, 0.0, 0.0, 0.0, -8.815628815628816], "Dports"=0, "AI RAW"=[]}, {"Address"=3, "DI"=[], "status"={"status"=TRUE, "code"=-1073807339, "source"="Failed to read IO: "}, "AI"=[0.0], "Dports"=0, "AI RAW"=[]}, {"Address"=4, "DI"=[], "status"={"status"=TRUE, "code"=-1073807339, "source"="Failed to read IO: "}, "AI"=[0.0], "Dports"=0, "AI RAW"=[]}, {"Address"=5, "DI"=[], "status"={"status"=TRUE, "code"=-1073807339, "source"="Failed to read IO: "}, "AI"=[0.0], "Dports"=0, "AI RAW"=[]}] ("Dout List"), Variant=w1640) -> (data=w1637:T13[], error out=w1639:errorcluster)  [unwired: 1 in]
                    n934 = local read "IO Map DO"() -> (w1636:T37[])
                    n935 = local read "IO Map AI"() -> (w1635:T39[])
                    n936 = local read "IO Map DI"() -> (w1633:T40[])
                    n937 = call "helper-snapshot-update.vi"("Snapshot"=w1637, "IO Map DI in"=w1633, "IO Map AI in"=w1635, "IO Map DO in"=w1636) -> ("IO Map DI out"=w1634:T40[], "IO Map AI out"=w1642:T39[], "IO Map DO out"=w1641:T37[], "AI RAW"=w1630:dbl[][], "AI"=w1631:dbl[][])  [unwired: 3 in]
                    n938 = property on="State" class="Bool (strict)"("DisabledEnum"=T71."Enabled" ("Disabled")) -> ()  [unwired: 2 in, 2 out]
                    n939 = local write "IO Map DO"(w1641) -> ()
                    n940 = local write "IO Map DI"(w1634) -> ()
                    n941 = local write "IO Map AI"(w1642) -> ()
                    n942 = Select(t=w1631, s="Calib?", f=w1630) -> (s? t:f=→"AI":dbl[][])
                  }
                }
              }
              frame "LOG.SNAPSHOT.PROC" {
                # "\"LOG.UPDATE.STATUS\" (PROCS) - \nget ENG STATS of procs and IO conf"
                n943 = disable-structure shown="Enabled" {
                  disable-tunnel: w1644 -> [w1651 w1664]
                  disable-tunnel: [_ w1663] -> w1643
                  frame Disabled {
                    w1650 = cluster{"Procedure":variant[]}[] []  # Clustered Proces
                    # "\"LOG.UPDATE.STATUS\" (PROCS)\nUPDATE RUNTIME LIST AND CLEAR LOG BUFFERS (MUST BE CALLED FROM ENG)"
                    n944 = Variant To Data(type=w1650, Variant=w1651) -> (data=w1648:cluster{"Procedure":variant[]}[])  [unwired: 1 in, 1 out]
                    n945 = for {
                      tunnel: w1648 -> [w1657] mode=indexing
                      tunnel: [w1652] -> _ mode=indexing
                      n946 = Unbundle(w1657) -> ("Procedure"=w1654:variant[])
                      n947 = Index Array(array=w1654) -> (element=w1653:variant)  [unwired: 1 in]
                      n948 = call "proc.util.enumToStrProcVar.vi"("Proc var"=typeProcVarientName."procNameID" ("proc var")) -> ("String"=w1656:string)  [unwired: 10 in]
                      n949 = call-poly "variantCtrl.polymorphic.vi"("name in"=w1656, "Step in"=w1653) -> ("String Value"=w1652:string)  [unwired: 6 in, 3 out]
                    }
                    n950 = call "reg-log-ntr.vi"("Operation(Read)"=enum.report-filter."ClearAll" ("Operation(Collect)")) -> ("compact report"=w1645:T77[])  [unwired: 8 in, 2 out]
                    n951 = call "reg-log-irr.vi"("Operation(Read)"=enum.report-filter."ClearAll") -> ("compact report"=w1646:T77[])  [unwired: 8 in, 2 out]
                    n952 = local write item#-1(w1645) -> ()
                    n953 = local write item#-1(w1646) -> ()
                    n954 = local write item#-1(w1646) -> ()
                  }
                  frame Enabled {
                    w1665 = cluster{"Procedure":variant[]}[] []  # Clustered Proces
                    n955 = Variant To Data(type=w1665, Variant=w1664) -> (data=w1662:cluster{"Procedure":variant[]}[], error out=w1663:errorcluster)  [unwired: 1 in]
                    n956 = local read "Proc Select 2"() -> (w1658:string)
                    n957 = call "util.procs.find-by-name.vi"("ProcName in"=w1658, "Procs in"=w1662) -> ("Found Proc"=w1661:cluster{"Procedure":variant[]})  [unwired: 4 in, 5 out]
                    n958 = Unbundle By Name(w1661) -> ("Procedure"=w1660:variant[])
                    n959 = call "build.proc.parse.vi"("Array in"=w1660) -> ("Flow Steps"=→"UiBuildSteps 2":T49[])  [unwired: 8 in, 2 out]
                  }
                }
              }
              frame "LOG.UPDATE.IRR" {
                n960 = control-ref of="Solar Elevation Graph"() -> (w1680:refnum<vi>)
                n961 = global read "globals-engine.vi" "IRR Params"() -> (w1670:T31)
                n962 = call "nrs.sunrise-time-table.vi"() -> ("Irrigation Timing"=w1674:T87, "Sunrise Timing"=w1679:cluster{"Sunset":timestamp, "Sunrise":timestamp}, "Solar Elevation Graph"=→"Solar Elevation Graph":waveform(dbl))  [unwired: 9 in]
                n963 = Unbundle By Name(w1670) -> ("timeLimits.Irrigation"=w1669:dbl, "timeLimits.Nut./Water"=w1668:dbl)
                n964 = property on="Day Time" class="Clust (strict)"("Value"=w1679) -> ()  [unwired: 2 in, 2 out]
                n965 = property on="Calculated Timing" class="Clust (strict)"("Value"=w1674) -> ()  [unwired: 2 in, 2 out]
                n966 = Unbundle By Name(w1674) -> ("Irrigation Timeout"=w1672:timestamp, "Fertiliztion Timeout"=w1673:timestamp)
                n967 = Unbundle By Name(w1679) -> ("Sunset"=w1678:timestamp, "Sunrise"=w1676:timestamp)
                n968 = Absolute Value(x=w1669) -> (abs(x)=w1667:dbl)
                n969 = Absolute Value(x=w1668) -> (abs(x)=w1666:dbl)
                n970 = To Double Precision Float(number=w1678) -> (double precision float=w1677:dbl)
                n971 = To Double Precision Float(number=w1676) -> (double precision float=w1675:dbl)
                n972 = To Double Precision Float(number=w1673) -> ()  [unwired: 1 out]
                n973 = To Double Precision Float(number=w1672) -> ()  [unwired: 1 out]
                n974 = call "Add Cursors To Graph.vi"("Sunset Time"=w1677, "Sunrise Time"=w1675, "Solar Elevation Graph Ref"=w1680, "Postpone Time"=w1667, "Fresh Water Time"=w1666) -> ("error out"=w1671:errorcluster)  [unwired: 10 in]
              }
              frame "LOG.UPDATE.SELECTORS" {
                # "\"LOG.UPDATE.STATUS\" (PROCS) - \nget ENG STATS of procs and IO conf"
                n975 = disable-structure shown="Enabled" {
                  frame Disabled {
                    w1688 = cluster{"Procedure":variant[]}[] []  # Clustered Proces
                    # "\"LOG.UPDATE.STATUS\" (PROCS)\nUPDATE RUNTIME LIST AND CLEAR LOG BUFFERS (MUST BE CALLED FROM ENG)"
                    n976 = Variant To Data(type=w1688) -> (Variant=w1689:cluster{"Procedure":variant[]}[], data=w1686:cluster{"Procedure":variant[]}[])  [unwired: 1 in, 1 out]
                    n977 = for {
                      tunnel: w1686 -> [w1695] mode=indexing
                      tunnel: [w1690] -> _ mode=indexing
                      n978 = Unbundle(w1695) -> ("Procedure"=w1692:variant[])
                      n979 = Index Array(array=w1692) -> (element=w1691:variant)  [unwired: 1 in]
                      n980 = call "proc.util.enumToStrProcVar.vi"("Proc var"=typeProcVarientName."procNameID" ("proc var")) -> ("String"=w1694:string)  [unwired: 10 in]
                      n981 = call-poly "variantCtrl.polymorphic.vi"("name in"=w1694, "Step in"=w1691) -> ("String Value"=w1690:string)  [unwired: 6 in, 3 out]
                    }
                    n982 = call "reg-log-ntr.vi"("Operation(Read)"=enum.report-filter."ClearAll" ("Operation(Collect)")) -> ("compact report"=w1683:T77[])  [unwired: 8 in, 2 out]
                    n983 = call "reg-log-irr.vi"("Operation(Read)"=enum.report-filter."ClearAll") -> ("compact report"=w1684:T77[])  [unwired: 8 in, 2 out]
                    n984 = local write item#-1(w1683) -> ()
                    n985 = local write item#-1(w1684) -> ()
                    n986 = local write item#-1(w1684) -> ()
                  }
                  frame Enabled {
                    n987 = call "variantCtrlIo.vi"("menu (Get Param)"=enumVarCtrlIO."IO List Configs") -> ("IO Configs List"=w1696:T42[])  [unwired: 6 in, 4 out]
                    n988 = stacked-sequence {
                      tunnel: w1696 -> [w1698 w1708 w1722 _]
                      frame #0 {
                        # "list all I/O"
                        n989 = disable-structure shown="Disabled" {
                          disable-tunnel: w1698 -> [w1701 _]
                          frame Disabled {
                            w1699 = T3[] [enum."AI", enum."DI", enum."DO"] items=["Type", "DI", "DO", "AI", "AO", "VL", "BUF"] ("Array")
                            n990 = for {
                              tunnel: w1699 -> [w1703] mode=indexing
                              tunnel: w1701 -> [w1707]
                              tunnel: [w1706] -> _ mode=concatenating
                              tunnel: [w1704] -> _ mode=indexing
                              tunnel: enum.io.mode."Mode" ("Mode(Any)") -> [w1702]
                              n991 = call "io-find-by-type.vi"("Mode(Any)"=w1702, "Type"=w1703, "IOConfigs in"=w1707) -> ("Search Results"=w1706:T42[])  [unwired: 8 in]
                              n992 = Array Size(array=w1706) -> (size(s)=w1705:i32)
                              n993 = Bundle("type"=w1703, w1705) -> (w1704:cluster{"type":T3, i32})  [unwired: 1 in]
                            }
                          }
                          frame Enabled {
                          }
                        }
                      }
                      frame #1 {
                        # "update AIN selectors"
                        n994 = call "io-find-by-type.vi"("Mode(Any)"=enum.io.mode."Mode", "Type"=enum.io.type."AI", "IOConfigs in"=w1708) -> ("Search Results"=w1715:T42[])  [unwired: 8 in]
                        n995 = for {
                          tunnel: w1715 -> [w1721] mode=indexing
                          tunnel: [w1718] -> w1714 mode=indexing
                          tunnel: [w1718] -> w1713 mode=indexing if=w1717
                          n996 = Unbundle By Name(w1721) -> ("Label"=w1718:string, "Mode"=w1720:T38)
                          n997 = Equal?(x=w1720, y=enum.io.mode."SIM") -> (x = y?=w1717:bool)
                        }
                        "Simulated" <- w1713
                        n998 = Sort 1D Array(array=w1714) -> (sorted array=w1710:string[])
                        n999 = Index Array(array=w1710) -> (element=w1711:string)  [unwired: 1 in]
                        n1000 = property on="IO calib select" class="CmbBox"("Strings[]"=w1710, "Value"=w1711) -> ()  [unwired: 2 in, 2 out]
                        n1001 = property on="IO Simulat select" class="CmbBox"("Strings[]"=w1710, "Value"="") -> ()  [unwired: 2 in, 2 out]
                      }
                      frame #2 {
                        w1724 = map{string, u8} {}  # Size: 0
                        # "create map:\n{\n  key: deviceAddressStr\n  Value: deviceAddressNum\n}"
                        # "list hardware addresses from I/O confs"
                        n1002 = for {
                          tunnel: w1722 -> [w1737] mode=indexing
                          tunnel: [w1736] -> w1725 mode=indexing
                          workers-P: _ -> [_]
                          n1003 = Unbundle By Name(w1737) -> ("ADDR"=w1736:T8)  [unwired: 2 out]
                        }
                        n1004 = for {
                          shift-right: [w1734] -> w1726
                          shift-left: w1724 -> [w1735]
                          tunnel: w1725 -> [w1732] mode=indexing
                          n1005 = call "util-address-parser.vi"("ADDR 2"=w1732) -> ("Address"=w1731:u8)  [unwired: 9 in, 1 out]
                          n1006 = Number To Decimal String(number=w1731) -> (decimal integer string=w1733:string)  [unwired: 1 in]
                          n1007 = Insert Into Map(map in=w1735, key=w1733, value=w1731) -> (map out=w1734:map{string, u8})  [unwired: 2 out]
                        }
                        n1008 = for {
                          tunnel: w1726 -> [w1730] mode=indexing
                          tunnel: [w1727] -> w1723 mode=indexing
                          workers-P: _ -> [_]
                          # "list map values"
                          n1009 = Unbundle By Name(w1730) -> ("Address"=w1728:u8)
                          n1010 = Bundle("Address"=w1728, "status"=TRUE) -> (w1727:cluster{"Address":u8, "status":bool})  [unwired: 1 in]
                        }
                        "RIO List" <- w1723
                      }
                      frame #3 {
                        # "list ICC folder for proc filenames and update section selector"
                        n1011 = call "util-path.vi"("append path (ie. folder\\filename.*)"="ICC" ("dir name")) -> ("error out"=w1740:errorcluster, "SelectedPath"=w1741:path)  [unwired: 6 in, 3 out]
                        n1012 = List Folder(path=w1741, error in=w1740) -> (folder names=w1743:string[], error out=w1739:errorcluster)  [unwired: 2 in, 2 out]
                        n1013 = Index Array(array=w1743) -> (element=w1742:string)  [unwired: 1 in]
                        n1014 = property on="Section" class="CmbBox"(error in=w1739, "Strings[]"=w1743, "Value"=w1742) -> (error out=w1738:errorcluster)  [unwired: 1 in, 1 out]
                        n1015 = case shown="No Error" w1738 {
                          frame No Error {
                          }
                          frame Error {
                          }
                        }
                      }
                    }
                  }
                }
              }
            }
            n1016 = call "helper-log-log.vi"("error in"=w1456, "Enum"=w1454) -> ("Collected Reports"=→"Collected Reports 2":string)  [unwired: 8 in, 1 out]
          }
        }
      }
      frame Error {
        # "handle error by displaying a continue/stop message dialog."
      }
    }
    n1017 = case shown="\"\"" w1434 {
      selector: w1434 -> [_ w1445]
      frame "" {
        # "skip empty statuts"
      }
      frame Default {
        # "status register"
        n1018 = call "reg-status.vi"("Operation(Read)"=enum.report-filter."Collect", "Reports to Collect"=w1445) -> ("Collected Reports"=w1444:string)  [unwired: 8 in, 1 out]
        n1019 = local write "User messages"(w1444) -> ()
      }
    }
    n1020 = call "util-collect-error.vi"("error in (no error)"=w1429, "Array in"=w1431) -> ("Array out"=w1430:errorcluster[])  [unwired: 9 in]
    "monitor" <- w1430
    "Log" <- w1432
  }
  n1021 = while "LOCAL MEASUREMENT RECORD" {
    tunnel: w10 -> [w1753]
    tunnel: w9 -> [w1754]
    shift-right: [w1750] -> _
    shift-left: _ -> [w1749]
    shift-right: [w1748] -> _
    shift-left: errorcluster[] [] ("Array out") -> [w1747]
    i -> [w1751]
    stop <- w1758 stop-if-true
    n1022 = Get Date/Time In Seconds() -> (seconds since 1Jan1904=w1752:timestamp)
    n1023 = Dequeue Element(queue=w1753, timeout in ms (-1)=250, error in (no error)=w1754) -> (queue out=w1757:refnum<queue>, element=w1759:cluster{"data":variant, "Enum":T54}, timed out?=w1756:bool, error out=w1760:errorcluster)
    n1024 = case shown="No Error" w1760 {
      selector: w1760 -> [_ w1864]
      tunnel: w1759 -> [w1766 _]
      tunnel: [w1763 _] -> w1758
      tunnel: w1757 -> [w1767 _]
      tunnel: w1756 -> [w1765 _]
      tunnel: [w1764 w1864] -> w1746
      tunnel: w1752 -> [_ _]
      tunnel: [w1762 w1863] -> w1750
      tunnel: w1749 -> [w1761 w1863]
      frame No Error {
        n1025 = case shown="False" w1765 {
          tunnel: w1767 -> [_ w1792]
          tunnel: w1766 -> [_ w1790]
          tunnel: [w1769 w1788] -> w1764
          tunnel: [_ w1791] -> w1763
          tunnel: [w1773 w1785] -> w1762
          tunnel: w1761 -> [w1773 w1784]
          frame True {
            # "Queue Timeout"
            n1026 = call "step.util.flag-matching.vi"("include step flags"=FALSE, "$string in"="serial\\serial-$date.*" ("append path (ie. folder\\filename.*)")) -> ("formated string out"=w1778:string)  [unwired: 9 in]
            n1027 = Refnum to Path(1:w1773) -> (0:w1772:path)
            n1028 = call "util-path.vi"("Create Folders?(F)"=TRUE, "Selected Folder (PROCS)"=typePathSelector."DIR_LOG" ("Selected Folder (PROCEDURE_DIR)"), "append path (ie. folder\\filename.*)"=w1778) -> ("error out"=w1768:errorcluster, "SelectedPath"=w1771:path)  [unwired: 4 in, 3 out]
            n1029 = Not Equal?(x=w1772, y=w1771) -> (x != y?=w1770:bool)
            n1030 = case shown="False" w1770 {
              tunnel: [w1779 w1781] -> w1769
              tunnel: w1768 -> [w1779 w1780]
              frame False {
              }
              frame True {
                n1031 = global read "globals-engine.vi" "Q-Com"() -> (w1782:refnum<queue>)
                n1032 = Enqueue Element At Opposite End(queue=w1782, element=cluster{"data":variant, "Enum":T54} {"data"=variant, "Enum"=enum."REC.REOPEN-FILE"} ("procQ"), error in (no error)=w1780) -> (error out=w1781:errorcluster)  [unwired: 1 in, 2 out]
              }
            }
          }
          frame False {
            # "Command Handler"
            n1033 = Unbundle(w1790) -> ("data"=w1789:variant, "Enum"=w1787:T54)
            n1034 = case shown="\"REC.SERIAL\"" w1787 {
              tunnel: w1792 -> [w1797 _ _ w1804 w1822 _ _ w1862]
              tunnel: [w1795 _ _ w1803 w1821 w1837 w1847 w1860] -> w1788
              tunnel: [TRUE _ _ _ _ _ _ _] -> w1791
              tunnel: w1789 -> [_ _ _ w1807 w1825 _ _ _]
              tunnel: T53 {"Caller"="", "IOnode"={"ADDR"=0, "Label"="Name", "Type"=enum."DI", "Mode"=enum."RIO", "Value"="Value", "Tags"="Tags", "calibration"=[]}, "error"={"status"=FALSE, "code"=0, "source"=""}, "dports"=[], "AIN (calib)"=0.0, "AIN (raw)"=0, "Times Stamp"=timestamp(0 s since 1904-01-01), "Record File Path"=path "", "Visa Data"=""} ("input cluster") -> [_ _ _ w1802 w1820 _ w1849 _]
              tunnel: [w1793 w1799 w1800 w1801 w1819 w1845 w1848 w1859] -> w1785
              tunnel: w1784 -> [w1793 w1799 w1800 w1801 w1819 w1845 _ w1859]
              frame "REC.EXIT" {
                n1035 = Close File(refnum=w1793) -> (error out=w1794:errorcluster)  [unwired: 1 in, 1 out]
                n1036 = Release Queue(queue=w1797) -> (error out=w1796:errorcluster)  [unwired: 2 in, 2 out]
                n1037 = Merge Errors(w1796, w1794) -> (w1795:errorcluster)
              }
              frame "REC.INIT" {
              }
              frame "REC.NO_OP", Default {
              }
              frame "REC.SERIAL" {
                # "\"REC.SERIAL\" \nLOGS SERIAL PORT COMMUNICATION"
                n1038 = Variant To Data(type=w1802, Variant=w1807) -> (data=w1805:T53, error out=w1806:errorcluster)  [unwired: 1 in]
                n1039 = stacked-sequence {
                  tunnel: w1806 -> [w1814]
                  tunnel: w1805 -> [w1810]
                  tunnel: w1804 -> [_]
                  tunnel: [w1809] -> w1803
                  tunnel: w1801 -> [w1815]
                  frame #0 {
                    n1040 = disable-structure shown="Enabled" {
                      disable-tunnel: w1810 -> [w1816 _]
                      frame Disabled {
                        n1041 = call "helper-serial-log-to-string.vi"("input cluster"=w1816) -> ("String"=w1818:string)  [unwired: 8 in, 2 out]
                        n1042 = call "reg-visa.vi"("Operation(Read)"=enum.report-filter."Collect", "Reports to Collect"=w1818) -> ()  [unwired: 8 in, 2 out]
                      }
                      frame Enabled {
                      }
                    }
                    n1043 = Write Datalog(4:w1814, 6:w1810, 7:w1815) -> (0:w1812:errorcluster, 3:w1813:refnum<k1>)
                    n1044 = Get Number of Records(4:w1812, 7:w1813) -> (0:w1808:errorcluster, 2:→"COM Size":i64)  [unwired: 1 out]
                    n1045 = Merge Errors(w1808) -> (w1809:errorcluster)
                  }
                }
              }
              frame "REC.IO" {
                # "\"REC.IO\" \nRECORD I/O MEASURMENT FILES."
                n1046 = Variant To Data(type=w1820, Variant=w1825) -> (data=w1823:T53, error out=w1824:errorcluster)  [unwired: 1 in]
                n1047 = stacked-sequence {
                  tunnel: w1824 -> [_]
                  tunnel: w1823 -> [w1828]
                  tunnel: w1822 -> [_]
                  tunnel: [w1826] -> w1821
                  tunnel: w1819 -> [_]
                  frame #0 {
                    n1048 = call "helper-eng-rec.vi"("input cluster"=w1828) -> ("error"=w1827:errorcluster)  [unwired: 10 in]
                    n1049 = Merge Errors(w1827) -> (w1826:errorcluster)
                  }
                }
              }
              frame "REC.FETCH" {
                n1050 = local read "COM Size"() -> (w1834:i64)
                n1051 = In Range and Coerce(upper limit=w1834, x="Snapshot Size", lower limit=i64 0) -> (coerced(x)=w1832:i64)  [unwired: 1 out]
                n1052 = Negate(x=w1832) -> (-x=w1836:i64)
                n1053 = Set Datalog Position(5:enum16{"start", "end", "current"}."end" ("from (0:start)"), 6:w1836, 7:w1845) -> (0:w1844:errorcluster, 3:w1842:refnum<k1>)  [unwired: 1 in]
                n1054 = Read Datalog(4:w1844, 6:w1832, 7:w1842) -> (0:w1838:errorcluster, 2:w1829:T53[], 3:w1840:refnum<k1>)
                "Serial Record(s)" <- w1829
                n1055 = call "helper-serial-log-to-string-2.vi"("Array in"=w1829) -> ("Array out"=w1830:T51[])  [unwired: 10 in]
                n1056 = call <vilib>:"Clear Errors.vi"("error in (no error)"=w1838) -> ("error out"=w1835:errorcluster)  [unwired: 5 in, 1 out]
                n1057 = local write "COM Snapshot"(w1830) -> ()
                n1058 = Set Datalog Position(4:w1835, 5:enum16{"start", "end", "current"}."end" ("from (0:start)"), 6:i64 0 ("offset (in records) (0)"), 7:w1840) -> (0:w1837:errorcluster)  [unwired: 1 out]
              }
              frame "REC.OPEN-FILE" {
                n1059 = call "step.util.flag-matching.vi"("include step flags"=FALSE, "$string in"="serial\\serial-$date.*" ("append path (ie. folder\\filename.*)")) -> ("formated string out"=w1857:string)  [unwired: 9 in]
                n1060 = call "util-path.vi"("Create Folders?(F)"=TRUE, "Selected Folder (PROCS)"=typePathSelector."DIR_LOG" ("Selected Folder (PROCEDURE_DIR)"), "append path (ie. folder\\filename.*)"=w1857) -> ("error out"=w1846:errorcluster, "SelectedPath"=w1851:path)  [unwired: 4 in, 3 out]
                n1061 = Open/Create/Replace Datalog(5:w1849, 8:w1846, 10:T88."open or create" ("operation (0:open)"), 11:w1851) -> (0:w1847:errorcluster, 3:w1848:refnum<k1>)  [unwired: 2 in, 1 out]
                n1062 = Refnum to Path(1:w1848) -> (0:→"SelectedPath":path)
              }
              frame "REC.REOPEN-FILE" {
                n1063 = Close File(refnum=w1859) -> (error out=w1858:errorcluster)  [unwired: 1 in, 1 out]
                n1064 = Enqueue Element At Opposite End(queue=w1862, element=cluster{"data":variant, "Enum":T54} {"data"=variant, "Enum"=enum."REC.OPEN-FILE"} ("procQ"), error in (no error)=w1858) -> (error out=w1860:errorcluster)  [unwired: 1 in, 2 out]
              }
            }
          }
        }
      }
      frame Error {
        # "handle error by displaying a continue/stop message dialog."
      }
    }
    n1065 = call "util-collect-error.vi"("error in (no error)"=w1746, "Array in"=w1747) -> ("Array out"=w1748:errorcluster[])  [unwired: 9 in]
    "record" <- w1748
    "Com" <- w1751
  }
  n1066 = while "EXECUTION CONTROL" {
    tunnel: w20 -> [w1865]
    shift-right: [w1875] -> _
    shift-left: cluster{"Procedure":variant[]}[] [] ("Array 5") -> [w1878]
    shift-right: [w1867] -> w28
    shift-left: errorcluster[] [] ("Array out") -> [w1869]
    i -> [w1876]
    stop <- w1880 stop-if-true
    n1067 = disable-structure shown="Disabled" {
      disable-tunnel: w1865 -> [w1885 _]
      frame Disabled {
        n1068 = Get Queue Status(queue=w1885, return elements? (F)=TRUE) -> (elements=→"elements":cluster{"case":T5, "data":variant}[])  [unwired: 1 in, 7 out]
      }
      frame Enabled {
      }
    }
    n1069 = Dequeue Element(queue=w1865, timeout in ms (-1)="ENG ms") -> (queue out=w1879:refnum<queue>, element=w1881:cluster{"case":T5, "data":variant}, timed out?=w1877:bool, error out=w1882:errorcluster)  [unwired: 1 in]
    n1070 = case shown="No Error" w1882 {
      selector: w1882 -> [_ w2756]
      tunnel: w1881 -> [w1903 _]
      tunnel: [w1898 _] -> w1880
      tunnel: w1879 -> [w1904 _]
      tunnel: w1878 -> [w1902 w2758]
      tunnel: [w1901 w2758] -> w1875
      tunnel: w1877 -> [w1900 _]
      tunnel: [w1899 w2757] -> w1868
      tunnel: [w1891 _] -> w1870
      tunnel: [w1897 w2755] -> w1874
      tunnel: "Time Addition" -> [w1896 _]
      tunnel: "Clk Simulator" -> [w1895 _]
      frame No Error {
        n1071 = call "helper-eng-clock-src.vi"("Clk Simulator"=w1895, "Time Addition"=w1896) -> ("Clk Simulated"=→"Clock Simulation":bool, "CLK"=w1893:dbl)  [unwired: 7 in, 1 out]
        n1072 = Get Date/Time In Seconds() -> (seconds since 1Jan1904=w1892:timestamp)
        n1073 = To Double Precision Float(number=w1892) -> (double precision float=w1891:dbl)
        n1074 = case shown="False" w1900 {
          tunnel: w1904 -> [w1910 w1966]
          tunnel: w1903 -> [_ w1961]
          tunnel: w1902 -> [w1907 w1964]
          tunnel: [w1905 w1963] -> w1901
          tunnel: [w1909 w1957] -> w1899
          tunnel: [_ w1962] -> w1898
          tunnel: [w1906 w1960] -> w1897
          tunnel: w1893 -> [w1908 w1954]
          tunnel: w1891 -> [_ _]
          frame True {
            # "Queue Timeout  (procedure execution)"
            n1075 = disable-structure shown="Disabled" {
              disable-tunnel: w1910 -> [w1913 _ w1943]
              disable-tunnel: [w1912 w1928 w1931] -> w1909
              disable-tunnel: w1908 -> [_ w1921 w1932]
              disable-tunnel: w1907 -> [_ w1930 w1944]
              disable-tunnel: [_ "Engine execution" "Engine execution"] -> w1906
              disable-tunnel: [_ w1919 _] -> w1905
              frame Disabled {
                n1076 = property on="ProcedureRun" class="Bool (strict)"() -> ("Value"=w1911:bool)  [unwired: 2 in, 2 out]
                n1077 = case shown="True" w1911 {
                  tunnel: w1913 -> [w1915 w1918]
                  tunnel: [w1914 w1917] -> w1912
                  frame False {
                    n1078 = call "eng-call-execute.vi"("Queue in"=w1915) -> ("error out"=w1914:errorcluster)  [unwired: 10 in]
                  }
                  frame True {
                    n1079 = property on="ProcedureSelect" class="CmbBox"() -> ("Value"=w1916:string)  [unwired: 2 in, 2 out]
                    n1080 = call "eng-call-execute.vi"("Proc Name to Execute (empty: Execute All)"=w1916, "Queue in"=w1918) -> ("error out"=w1917:errorcluster)  [unwired: 9 in]
                  }
                }
              }
              frame Enabled {
                w1929 = -1  # execute all
                n1081 = To Time Stamp(1:w1921) -> (0:w1926:timestamp)
                n1082 = Get Date/Time String(seconds (now)=w1926, want seconds? (F)=TRUE) -> (date string=w1924:string, time string=w1925:string)  [unwired: 1 in]
                n1083 = Format Into String(format string="%s %s", w1924, w1925) -> (resulting string=→"clock":string)  [unwired: 2 in, 1 out]
                n1084 = call "engine.executor.vi"("Index(-1: All)"=w1929, "clk (NaN)"=w1921, "Procs in"=w1930) -> ("Error"=w1928:errorcluster, "Procs out"=w1919:cluster{"proc out":variant[]}[])  [unwired: 5 in, 2 out]
              }
              frame Disabled {
                w1942 = -1  # execute all
                n1085 = To Time Stamp(1:w1932) -> (0:w1938:timestamp)
                n1086 = Get Date/Time String(seconds (now)=w1938, want seconds? (F)=TRUE) -> (date string=w1936:string, time string=w1937:string)  [unwired: 1 in]
                n1087 = Format Into String(format string="%s %s", w1936, w1937) -> (resulting string=→"clock 3":string)  [unwired: 2 in, 1 out]
                n1088 = call "engine.executor.vi"("Index(-1: All)"=w1942, "clk (NaN)"=w1932, "Procs in"=w1944) -> ("Error"=w1941:errorcluster, "ErrorProcs out"=w1940:T96)  [unwired: 5 in, 2 out]
                n1089 = stacked-sequence {
                  tunnel: w1943 -> [_ w1950]
                  tunnel: w1941 -> [_ w1945]
                  tunnel: w1940 -> [_ _]
                  tunnel: [_ w1946] -> w1931
                  frame #0 {
                  }
                  frame #1 {
                    n1090 = property on="ProcedureStep" class="Bool (strict)"() -> ("Value"=w1947:bool)  [unwired: 2 in, 2 out]
                    n1091 = property on="Step" class="Bool (strict)"() -> ("Value"=w1949:bool)  [unwired: 2 in, 2 out]
                    n1092 = Or(x=w1949, y=w1947) -> (x .or. y?=w1948:bool)
                    n1093 = case shown="True" w1948 {
                      tunnel: w1950 -> [_ _]
                      tunnel: [_ w1953] -> w1946
                      tunnel: w1945 -> [_ w1951]
                      frame False {
                      }
                      frame True {
                        w1952 = FALSE ("flagEngRunStep")
                        n1094 = property on="Step" class="Bool (strict)"("Value"=w1952) -> ()  [unwired: 2 in, 2 out]
                        n1095 = property on="ProcedureStep" class="Bool (strict)"("Value"=w1952) -> ()  [unwired: 2 in, 2 out]
                        n1096 = call "eng-call-start.vi"("error in (no error)"=w1951, "Start(T)/Stop(F)"=w1952) -> ("error out"=w1953:errorcluster)  [unwired: 9 in]
                      }
                    }
                  }
                }
              }
            }
          }
          frame False {
            # "Command Handler"
            n1097 = Unbundle(w1961) -> ("case"=w1958:T5, "data"=w1965:variant)
            "case" <- w1958
            n1098 = case shown="\"ENG.INIT.VARS\"" w1958 {
              tunnel: w1966 -> [w1974 _ _ _ _ _ w2090 w2095 _ _ _ _ _ _ _ w2361 _ _ _ _ w2431 _ _ _ _ _ _ _ _ _ _ _ _ _]
              tunnel: w1965 -> [w1971 _ _ _ w2073 _ _ _ _ _ w2276 _ _ w2336 _ w2358 _ w2371 w2381 w2408 w2432 w2474 w2490 w2500 w2507 _ w2553 w2579 _ _ _ _ _ _]
              tunnel: w1964 -> [w1970 w2027 w2034 w2041 w2075 w2079 w2091 w2096 w2114 w2241 w2281 w2308 _ w2332 _ w2362 _ w2372 w2377 w2382 w2430 w2468 w2488 w2498 w2509 w2528 w2554 w2580 w2591 w2652 w2685 w2724 w2752 w2754]
              tunnel: [w1972 w2027 w2034 w2041 w2075 w2079 w2091 w2096 w2114 w2241 w2281 w2308 w2322 w2331 w2347 w2355 cluster{"Procedure":variant[]}[] [] ("t") w2372 w2380 w2399 w2430 w2469 w2489 w2499 w2509 w2528 w2554 w2580 w2591 w2652 w2685 w2724 w2752 w2754] -> w1963
              tunnel: [w1973 w2024 w2032 w2042 w2068 w2080 w2084 w2094 w2113 w2242 w2272 w2305 w2315 w2339 _ w2359 _ w2370 w2378 w2396 w2429 w2460 w2487 w2497 w2508 _ w2534 w2572 w2590 w2651 w2656 w2703 w2751 errorcluster {"status"=TRUE, "code"=-1, "source"="NO-OP is not a funtion"} ("error out")] -> w1956
              tunnel: [_ _ _ _ _ _ w2089 _ _ _ _ _ _ _ _ _ _ _ _ _ _ _ _ _ _ _ _ _ _ _ _ _ _ _] -> w1962
              tunnel: [w1969 w2023 w2031 _ _ _ _ _ _ _ _ _ _ _ _ _ _ _ _ _ _ _ w2482 w2492 "RIO Snapshot" _ w2531 w2563 _ _ _ _ _ _] -> w1960
              tunnel: [_ _ _ _ _ _ _ _ _ _ _ _ _ _ _ _ _ _ w2373 _ _ w2462 w2481 w2491 _ _ _ _ _ _ _ _ _ _] -> w1955
              tunnel: w1954 -> [w1967 _ _ _ _ _ _ _ _ _ _ _ _ _ _ _ _ _ _ _ _ _ _ _ _ _ _ _ _ _ _ _ _ _]
              frame "ENG.EXECUTE" {
                # "\"ENG.EXECUTE\" \nCall engine execution"
                n1099 = disable-structure shown="Enabled" {
                  disable-tunnel: w1974 -> [w1988 _]
                  disable-tunnel: [w1987 w2022] -> w1972
                  disable-tunnel: w1971 -> [w1985 _]
                  disable-tunnel: w1970 -> [w1983 w2022]
                  disable-tunnel: ["Engine execution" _] -> w1969
                  disable-tunnel: [w1976 _] -> w1968
                  disable-tunnel: w1967 -> [w1975 _]
                  frame Enabled {
                    w1982 = ""  # Proc Name
                    n1100 = Variant To Data(type=w1982, Variant=w1985) -> (data=w1981:string, error out=w1980:errorcluster)  [unwired: 1 in]
                    n1101 = case shown="Default" w1981 {
                      selector: w1981 -> [_ w2001]
                      tunnel: [w1999 w2005] -> w1986
                      tunnel: [w1998 w2004] -> w1984
                      tunnel: w1983 -> [_ w2003]
                      tunnel: w1980 -> [w1998 w2000]
                      frame "" {
                        w1999 = -1  # execute all
                        # "run all if called w/o name"
                      }
                      frame Default {
                        # "run single proc using name"
                        n1102 = call "util.procs.find-by-name.vi"("isRequired(T)"=TRUE ("isRequired"), "error in"=w2000, "ProcName in"=w2001, "Procs in"=w2003) -> ("error out"=w2004:errorcluster, "procIndex"=w2005:i32)  [unwired: 2 in, 4 out]
                      }
                    }
                    n1103 = disable-structure shown="Enabled" {
                      disable-tunnel: [w1995 w1997] -> w1987
                      disable-tunnel: w1986 -> [w1994 _]
                      disable-tunnel: w1984 -> [w1993 w1996]
                      disable-tunnel: w1983 -> [w1992 w1997]
                      disable-tunnel: w1975 -> [w1991 _]
                      disable-tunnel: [w1990 w1996] -> w1979
                      disable-tunnel: [w1989 _] -> w1978
                      frame Enabled {
                        n1104 = call "engine.executor.vi"("error"=w1993, "Index(-1: All)"=w1994, "clk (NaN)"=w1991, "Procs in"=w1992) -> ("Error"=w1990:errorcluster, "Procs out"=w1995:cluster{"proc out":variant[]}[], "ErrorProcs out"=w1989:T96)  [unwired: 4 in, 1 out]
                      }
                      frame Disabled {
                      }
                    }
                    n1105 = stacked-sequence {
                      tunnel: w1988 -> [_ w2018]
                      tunnel: w1979 -> [_ w2013]
                      tunnel: w1978 -> [_ _]
                      tunnel: [_ w2014] -> w1976
                      tunnel: w1975 -> [w2008 _]
                      frame #0 {
                        n1106 = To Time Stamp(1:w2008) -> (0:w2007:timestamp)
                        n1107 = Get Date/Time String(seconds (now)=w2007, want seconds? (F)=TRUE) -> (date string=w2012:string, time string=w2011:string)  [unwired: 1 in]
                        n1108 = Format Into String(format string="%s %s", w2012, w2011) -> (resulting string=w2006:string)  [unwired: 2 in, 1 out]
                        n1109 = local write "clock"(w2006) -> ()
                      }
                      frame #1 {
                        n1110 = property on="ProcedureStep" class="Bool (strict)"() -> ("Value"=w2015:bool)  [unwired: 2 in, 2 out]
                        n1111 = property on="Step" class="Bool (strict)"() -> ("Value"=w2017:bool)  [unwired: 2 in, 2 out]
                        n1112 = Or(x=w2017, y=w2015) -> (x .or. y?=w2016:bool)
                        n1113 = case shown="True" w2016 {
                          tunnel: w2018 -> [_ _]
                          tunnel: [_ w2021] -> w2014
                          tunnel: w2013 -> [_ w2019]
                          frame False {
                          }
                          frame True {
                            w2020 = FALSE ("flagEngRunStep")
                            n1114 = property on="Step" class="Bool (strict)"("Value"=w2020) -> ()  [unwired: 2 in, 2 out]
                            n1115 = property on="ProcedureStep" class="Bool (strict)"("Value"=w2020) -> ()  [unwired: 2 in, 2 out]
                            n1116 = call "eng-call-start.vi"("error in (no error)"=w2019, "Start(T)/Stop(F)"=w2020) -> ("error out"=w2021:errorcluster)  [unwired: 9 in]
                          }
                        }
                      }
                    }
                  }
                  frame Disabled {
                  }
                }
                n1117 = Merge Errors(w1968) -> (w1973:errorcluster)
              }
              frame "ENG.START" {
                w2023 = "Engine Started" ("t")
                # "\"ENG.RUN\" \nStart/stop runtime engine by changing Timeout"
                n1118 = local read "ENG ms ctrl"() -> (w2026:i32)
                n1119 = local write "ENG ms"(w2026) -> ()
                n1120 = local write "clock"(w2023) -> ()
                n1121 = disable-structure shown="Disabled" {
                  frame Enabled {
                    n1122 = property on="clock" class="Str"("Blinking"=FALSE) -> ()  [unwired: 2 in, 2 out]
                  }
                  frame Disabled {
                    n1123 = property on="User messages" class="Str"("Text.TextColor"=u32 0 ("Color Box")) -> ()  [unwired: 2 in, 2 out]
                  }
                }
                n1124 = property on="Run" class="Bool (strict)"("Value"=TRUE) -> (error out=w2024:errorcluster)  [unwired: 2 in, 1 out]
              }
              frame "ENG.STOP" {
                w2030 = -1 items=["ENG_STOP(-1)"=-1] ("UiInterval")
                w2031 = "Engine Paused" ("t")
                # "\"ENG.RUN\" \nStart/stop runtime engine by changing Timeout"
                n1125 = property on="Run" class="Bool (strict)"("Value"=FALSE) -> (error out=w2032:errorcluster)  [unwired: 2 in, 1 out]
                n1126 = disable-structure shown="Enabled" {
                  frame Enabled {
                    n1127 = property on="clock" class="Str"("Blinking"=TRUE) -> ()  [unwired: 2 in, 2 out]
                  }
                  frame Disabled {
                    n1128 = property on="User messages" class="Str"("Text.TextColor"=u32 16711680 ("Color Box")) -> ()  [unwired: 2 in, 2 out]
                  }
                }
                n1129 = local write "clock"(w2031) -> ()
                n1130 = local write "ENG ms"(w2030) -> ()
              }
              frame "ENG.STATUS" {
                # "\"ENG.STATUS\" \n1) create list of proc names (and paths) and update proc selectors\n2) call LOG.STATUS"
                n1131 = for "create list of proc names and set proc selectors" {
                  tunnel: w2041 -> [w2055] mode=indexing
                  tunnel: [w2054] -> w2038 mode=indexing
                  tunnel: [w2053] -> w2039 mode=indexing
                  n1132 = stacked-sequence {
                    tunnel: w2055 -> [w2061 w2067]
                    tunnel: [w2056 _] -> w2054
                    tunnel: [_ w2062] -> w2053
                    frame #0 {
                      n1133 = Unbundle(w2061) -> ("Procedure"=w2058:variant[])
                      n1134 = Index Array(array=w2058) -> (element=w2057:variant)  [unwired: 1 in]
                      n1135 = call "proc.util.enumToStrProcVar.vi"("Proc var"=typeProcVarientName."procNameID" ("proc var")) -> ("String"=w2060:string)  [unwired: 10 in]
                      n1136 = call-poly "variantCtrl.polymorphic.vi"("name in"=w2060, "Step in"=w2057) -> ("String Value"=w2056:string)  [unwired: 6 in, 3 out]
                    }
                    frame #1 {
                      n1137 = Unbundle(w2067) -> ("Procedure"=w2064:variant[])
                      n1138 = Index Array(array=w2064) -> (element=w2063:variant)  [unwired: 1 in]
                      n1139 = call "proc.util.enumToStrProcVar.vi"("Proc var"=typeProcVarientName."procPath" ("proc var")) -> ("String"=w2066:string)  [unwired: 10 in]
                      n1140 = call-poly "variantCtrl.polymorphic.vi"("name in"=w2066, "Step in"=w2063) -> ("String Value"=w2062:string)  [unwired: 6 in, 3 out]
                    }
                  }
                }
                n1141 = local write "Loaded Proc Path"(w2039) -> ()
                n1142 = Index Array(array=w2038) -> (element=w2037:string)  [unwired: 1 in]
                n1143 = property on="Proc Name" class="CmbBox"("Strings[]"=w2038, "Value"="" ("Proc Name")) -> ()  [unwired: 2 in, 2 out]
                n1144 = property on="ProcedureSelect" class="CmbBox"("Strings[]"=w2038, "Value"=w2037) -> ()  [unwired: 2 in, 2 out]
                n1145 = disable-structure shown="Enabled" {
                  disable-tunnel: [w2046 w2051 _] -> w2042
                  disable-tunnel: w2041 -> [w2043 _ _]
                  frame Disabled {
                    n1146 = global read "globals-engine.vi" "Q-Log"() -> (w2047:refnum<queue>)
                    n1147 = Bundle By Name(cluster=cluster{"data":variant, "Enum":T56} {"data"=variant, "Enum"=enum."LOG.UPDATE.SELECTORS"} ("procQ"), "data"=w2043) -> (w2044:cluster{"data":variant, "Enum":T56})
                    n1148 = Enqueue Element(queue=w2047, element=w2044) -> (error out=w2046:errorcluster)  [unwired: 2 in, 2 out]
                  }
                  frame Enabled {
                    n1149 = global read "globals-engine.vi" "Q-Log"() -> (w2052:refnum<queue>)
                    n1150 = Bundle By Name(cluster=cluster{"data":variant, "Enum":T56} {"data"=variant, "Enum"=enum."LOG.UPDATE.SELECTORS"} ("procQ"), "data"=variant) -> (w2049:cluster{"data":variant, "Enum":T56})
                    n1151 = Enqueue Element(queue=w2052, element=w2049) -> (error out=w2051:errorcluster)  [unwired: 2 in, 2 out]
                  }
                  frame Disabled {
                  }
                }
                n1152 = property on="Proc Select 2" class="CmbBox"("Strings[]"=w2038, "Value"=w2037) -> ()  [unwired: 2 in, 2 out]
              }
              frame "ENG.EXTERNAL-CALL" {
                n1153 = Variant To Data(type=T81 {"Q-Log"=refnum, "procQ"={"data"=variant, "Enum"=enum."LOG.NO_OP"}} ("output cluster"), Variant=w2073) -> (data=w2072:T81, error out=w2069:errorcluster)  [unwired: 1 in]
                n1154 = Unbundle By Name(w2072) -> ("Q-Log"=w2071:refnum<queue>, "procQ"=w2070:cluster{"data":variant, "Enum":T56})
                n1155 = Enqueue Element(queue=w2071, element=w2070, error in (no error)=w2069) -> (error out=w2068:errorcluster)  [unwired: 1 in, 2 out]
              }
              frame "ENG.PROC.STATUS" {
                n1156 = global read "globals-engine.vi" "Q-Log"() -> (w2078:refnum<queue>)
                n1157 = Bundle By Name(cluster=cluster{"data":variant, "Enum":T56} {"data"=variant, "Enum"=enum."LOG.SNAPSHOT.PROC"} ("procQ"), "data"=w2079) -> (w2076:cluster{"data":variant, "Enum":T56})
                n1158 = Enqueue Element(queue=w2078, element=w2076) -> (error out=w2080:errorcluster)  [unwired: 2 in, 2 out]
              }
              frame "ENG.EXIT" {
                w2089 = TRUE
                # "\"ENG.EXIT\""
                n1159 = global write "globals-engine.vi" "STOP"(w2089) -> ()
                n1160 = Release Queue(queue=w2090) -> (error out=w2085:errorcluster)  [unwired: 2 in, 2 out]
                n1161 = global read "globals-engine.vi" "Q-Log"() -> (w2087:refnum<queue>)
                n1162 = Enqueue Element At Opposite End(queue=w2087, element=cluster{"data":variant, "Enum":T56} {"data"=variant, "Enum"=enum."LOG.EXIT"} ("procQ")) -> (error out=w2088:errorcluster)  [unwired: 2 in, 2 out]
                n1163 = global read "globals-engine.vi" "Q-Com"() -> (w2083:refnum<queue>)
                n1164 = Enqueue Element At Opposite End(queue=w2083, element=cluster{"data":variant, "Enum":T54} {"data"=variant, "Enum"=enum."REC.EXIT"}) -> (error out=w2081:errorcluster)  [unwired: 2 in, 2 out]
                n1165 = Merge Errors(w2081, w2088, w2085) -> (w2084:errorcluster)
              }
              frame "ENG.INIT" {
                # "initialize engine before loading runtime procedures"
                n1166 = for {
                  tunnel: w2095 -> [w2099]
                  tunnel: [w2098] -> w2093
                  tunnel: cluster{"cmd":T5, "data":variant}[] [{"cmd"=enum."ENG.INIT.SERIAL", "data"=variant}, {"cmd"=enum."ENG.INIT.VARS", "data"=variant}] ("typedefElement") -> [w2097] mode=indexing
                  n1167 = Enqueue Element At Opposite End(queue=w2099, element=w2097) -> (error out=w2098:errorcluster)  [unwired: 2 in, 2 out]
                }
                n1168 = Merge Errors(w2093) -> (w2094:errorcluster)
              }
              frame "ENG.INIT.VARS" {
                # "initialize Globals (nutritionConf)"
                n1169 = stacked-sequence {
                  seq-local: [_ _ _ w2138 _ _ _] -> [_ _ _ _ w2227 _ _]
                  tunnel: [_ w2118 _ _ _ _ _] -> w2112
                  tunnel: [_ _ w2132 _ _ _ _] -> w2111
                  tunnel: [w2116 _ _ _ _ _ _] -> w2110
                  tunnel: [_ _ _ w2138 _ _ _] -> w2103
                  tunnel: [_ _ _ w2143 _ _ _] -> w2109
                  tunnel: [w2115 _ _ _ _ _ _] -> w2108
                  tunnel: [_ w2117 _ _ _ _ _] -> w2107
                  tunnel: [_ _ _ w2141 _ _ _] -> w2106
                  tunnel: [_ _ _ w2140 _ _ _] -> w2105
                  tunnel: [_ _ _ w2139 _ _ _] -> w2104
                  tunnel: [_ _ w2129 _ _ _ _] -> w2102
                  tunnel: [_ _ _ _ _ w2233 _] -> w2101
                  tunnel: [_ _ _ _ _ _ w2234] -> w2100
                  frame #0 {
                    # "load aux list"
                    n1170 = call "aux-conf-loader.vi"() -> ("error out"=w2116:errorcluster, "Array"=w2115:T97[])  [unwired: 10 in]
                  }
                  frame #1 {
                    # "Nutrition GLOBAL"
                    n1171 = call "util.file.vars.vi"("Directory (DIR_PROC)"=typePathSelector."DIR_CONFIG" ("location (PROCEDURE_DIR)"), "Proc Name(open dialog if empty)"="unit-nutrition" ("Filename.*  (opens dialog if empty and allow)")) -> ("error out"=w2120:errorcluster, "Vars[] out"=w2121:variant[])  [unwired: 5 in, 3 out]
                    n1172 = for {
                      tunnel: w2121 -> [w2128] mode=indexing
                      tunnel: [w2127] -> w2117 mode=indexing
                      tunnel: w2120 -> [w2125]
                      tunnel: [w2124] -> w2119
                      n1173 = Variant To Data(error in=w2125, type=T64 {"Main"={"Enable"=FALSE, "WashTimes"={"In"=0.0, "Out"=0.0}, "DailyActivityHours"=[]}, "Water Dosing"={"Water Dose"=0.0, "Water Limit"=0.0}, "EC Ranges"={"H Alarm"=0.0, "L Alarm"=0.0, "Low"=0.0}, "EC Dosing"={"ALFA1 Dose"=0.0, "ALFA1 Limit"=0.0, "BETA1 Dose"=0.0, "BETA1 Limit"=0.0, "ALFA2 Dose"=0.0, "ALFA2 Limit"=0.0, "BETA2 Dose"=0.0, "BETA2 Limit"=0.0}, "PH Ranges"={"H Alarm"=0.0, "L Alarm"=0.0, "High"=0.0, "Low"=0.0}, "PH Dosing"={"ACID Dose"=0.0, "ACID Limit"=0.0, "BASE Dose"=0.0, "BASE Limit"=0.0}, "ORP Ranges"={"H Alarm"=0.0, "L Alarm"=0.0, "Low"=0.0}, "ORP Dosing"={"MIX Dose"=0.0, "MIX Limit"=0.0}} ("Cluster"), Variant=w2128) -> (data=w2127:T64, error out=w2124:errorcluster)
                    }
                    n1174 = Merge Errors(w2119) -> (w2118:errorcluster)
                  }
                  frame #2 {
                    # "irrigation GLOBAL"
                    n1175 = call "util.file.vars.vi"("Directory (DIR_PROC)"=typePathSelector."DIR_CONFIG" ("location (PROCEDURE_DIR)"), "Proc Name(open dialog if empty)"="IRR_CONF" ("Filename.*  (opens dialog if empty and allow)")) -> ("error out"=w2134:errorcluster, "Vars[] out"=w2135:variant[])  [unwired: 5 in, 3 out]
                    n1176 = Index Array(array=w2135) -> (element=w2131:variant)  [unwired: 1 in]
                    n1177 = Variant To Data(error in=w2134, type=T31 {"Day Time"={"Sunset"=timestamp(0 s since 1904-01-01), "Sunrise"=timestamp(0 s since 1904-01-01)}, "timeLimits"={"Irrigation"=0.0, "Nut./Water"=0.0}, "Calculated Timing"={"Irrigation Timeout"=timestamp(0 s since 1904-01-01), "Nutrients Timeout"=timestamp(0 s since 1904-01-01)}, "Irr Dosing Time"={"Nutrients"=250, "Water"=250, "Wash"=250}, "UV Limit "=250.0, "Dose Table"=[{"Enable"=TRUE, "output"="IRR_SEC1"}, {"Enable"=FALSE, "output"="IRR_SEC2"}, {"Enable"=FALSE, "output"="IRR_SEC3"}, {"Enable"=FALSE, "output"="IRR_SEC4"}, {"Enable"=FALSE, "output"="IRR_SEC5"}, {"Enable"=FALSE, "output"="IRR_SEC6"}], "Last Iteration"=timestamp(0 s since 1904-01-01), "UV Reduction Status"=FALSE, "UV Reduction"=99} ("irr panel"), Variant=w2131) -> (data=w2129:T31, error out=w2133:errorcluster)
                    n1178 = Merge Errors(w2133) -> (w2132:errorcluster)
                  }
                  frame #3 {
                    w2142 = 500  # ms default
                    # "INI to GLOBALs"
                    n1179 = call "util-path.vi"("Create Folders?(F)"=FALSE, "Selected Folder (PROCS)"=typePathSelector."DIR_INI" ("Selected Folder (PROCEDURE_DIR)")) -> ("error out"=w2150:errorcluster, "SelectedPath"=w2151:path)  [unwired: 5 in, 3 out]
                    n1180 = call <vilib>:"Open Config Data.vi"("error in (no error)"=w2150, "configuration file path"=w2151) -> ("error out"=w2144:errorcluster, "refnum"=w2147:T63)  [unwired: 7 in, 1 out]
                    n1181 = case shown="No Error" w2144 {
                      selector: w2144 -> [_ w2221]
                      tunnel: [w2171 _] -> w2154
                      tunnel: [w2170 _] -> w2153
                      tunnel: [w2169 _] -> w2152
                      tunnel: w2147 -> [w2168 w2220]
                      tunnel: [w2167 w2220] -> w2146
                      tunnel: [w2165 w2221] -> w2145
                      tunnel: [w2161 _] -> w2141
                      tunnel: [w2159 w2219] -> w2140
                      tunnel: w2142 -> [w2158 w2219]
                      tunnel: [w2156 _] -> w2139
                      frame No Error {
                        n1182 = stacked-sequence {
                          tunnel: [w2175 _ _ _ _ _] -> w2169
                          tunnel: [_ w2182 _ _ _ _] -> w2170
                          tunnel: [_ _ w2188 _ _ _] -> w2171
                          tunnel: [_ w2180 _ _ _ _] -> w2164
                          tunnel: w2168 -> [w2174 w2179 w2186 w2193 w2202 w2215]
                          tunnel: [w2173 _ _ _ _ _] -> w2166
                          tunnel: [w2172 _ _ _ _ _] -> w2167
                          tunnel: [_ _ w2185 _ _ _] -> w2163
                          tunnel: [_ _ _ w2192 _ _] -> w2162
                          tunnel: [_ _ _ w2191 _ _] -> w2161
                          tunnel: [_ _ _ _ w2201 _] -> w2160
                          tunnel: [_ _ _ _ w2200 _] -> w2159
                          tunnel: w2158 -> [_ _ _ _ w2197 _]
                          tunnel: [_ _ _ _ _ w2212] -> w2157
                          tunnel: [_ _ _ _ _ w2206] -> w2156
                          frame #0 {
                            n1183 = call "util-ini-key.vi"("key"=ini-key."INI.LOCAL.LONGITUDE" ("input 1")) -> ("key"=w2178:string, "section"=w2176:string)  [unwired: 9 in]
                            n1184 = call-poly <vilib>:"Read Key.vi"("section"=w2176, "key"=w2178, "refnum"=w2174) -> ("error out"=w2173:errorcluster, "value"=w2175:dbl, "refnum out"=w2172:T63)  [unwired: 5 in, 1 out]
                          }
                          frame #1 {
                            n1185 = call "util-ini-key.vi"("key"=ini-key."INI.LOCAL.LATITUDE" ("input 1")) -> ("key"=w2184:string, "section"=w2181:string)  [unwired: 9 in]
                            n1186 = call-poly <vilib>:"Read Key.vi"("section"=w2181, "key"=w2184, "refnum"=w2179) -> ("error out"=w2180:errorcluster, "value"=w2182:dbl)  [unwired: 5 in, 2 out]
                          }
                          frame #2 {
                            n1187 = call "util-ini-key.vi"("key"=ini-key."INI.LOCAL.TIMEZONE" ("input 1")) -> ("key"=w2190:string, "section"=w2187:string)  [unwired: 9 in]
                            n1188 = call-poly <vilib>:"Read Key.vi"("section"=w2187, "key"=w2190, "refnum"=w2186) -> ("error out"=w2185:errorcluster, "value"=w2188:dbl)  [unwired: 5 in, 2 out]
                          }
                          frame #3 {
                            n1189 = call "util-ini-key.vi"("key"=ini-key."INI.PROJECT_NAME" ("input 1")) -> ("key"=w2196:string, "section"=w2194:string)  [unwired: 9 in]
                            n1190 = call-poly <vilib>:"Read Key.vi"("section"=w2194, "key"=w2196, "refnum"=w2193) -> ("error out"=w2192:errorcluster, "value"=w2191:string)  [unwired: 5 in, 2 out]
                          }
                          frame #4 {
                            n1191 = call "util-ini-key.vi"("key"=ini-key."INI.ENG.INTERVAL_MS" ("input 1")) -> ("key"=w2205:string, "section"=w2203:string)  [unwired: 9 in]
                            n1192 = call-poly <vilib>:"Read Key.vi"("section"=w2203, "key"=w2205, "refnum"=w2202) -> ("error out"=w2201:errorcluster, "value"=w2199:i32, "found?"=w2198:bool)  [unwired: 5 in, 1 out]
                            n1193 = Select(t=w2199, s=w2198, f=w2197) -> (s? t:f=w2200:i32)
                          }
                          frame #5 {
                            w2208 = typeEnv."ENV.PRODUCTION" ("ENV in")
                            n1194 = call "util-ini-key.vi"("key"=ini-key."INI.ENV" ("input 1")) -> ("key"=w2218:string, "section"=w2216:string)  [unwired: 9 in]
                            n1195 = call-poly <vilib>:"Read Key.vi"("section"=w2216, "key"=w2218, "refnum"=w2215) -> ("error out"=w2213:errorcluster, "value"=w2211:string, "found?"=w2210:bool)  [unwired: 5 in, 1 out]
                            n1196 = Scan From String(input string=w2211, default 1=w2208) -> (output 1=w2209:T1)  [unwired: 3 in, 3 out]
                            n1197 = Select(t=w2209, s=w2210, f=w2208) -> (s? t:f=w2207:T1)
                            n1198 = call "util.environment.vi"("error in"=w2213, "Operation (Get)"=enum16{"get", "set"}."set", "ENV in"=w2207) -> ("error out"=w2212:errorcluster, "ENV out"=w2206:T1)  [unwired: 7 in]
                          }
                        }
                        n1199 = Merge Errors(w2166, w2164, w2163, w2162, w2160, w2157) -> (w2165:errorcluster)
                      }
                      frame Error {
                      }
                    }
                    n1200 = global read "globals-engine.vi" "ProjectSettings"() -> (w2155:T12)
                    n1201 = Bundle By Name(cluster=w2155, "Longitude"=w2152, "Latitude"=w2153, "TimeZone"=w2154) -> (w2138:T12)
                    n1202 = call <vilib>:"Close Config Data.vi"("error in (no error)"=w2145, "refnum"=w2146) -> ("error out"=w2143:errorcluster)  [unwired: 8 in, 1 out]
                  }
                  frame #4 {
                    n1203 = Unbundle By Name(w2227) -> ("Latitude"=w2225:dbl, "Longitude"=w2224:dbl, "TimeZone"=w2223:i32)
                    n1204 = local read "UiProjectSettings"() -> (w2226:T19)
                    n1205 = Bundle By Name(cluster=w2226, "Latitude"=w2225, "Longitude"=w2224, "TimeZone"=w2223) -> (w2222:T19)
                    n1206 = local write "UiProjectSettings"(w2222) -> ()
                  }
                  frame #5 {
                    # "INIT PBR PROC SELECTOR"
                    n1207 = call "pbr-get-procs-names.vi"() -> ("error out"=w2233:errorcluster, "Array"=w2232:string[])  [unwired: 10 in]
                    n1208 = local write "PBR Builder"(T23 [] ("PBR Builder")) -> ()
                    n1209 = local write "PBR_PLAY"(cluster{"PLAY":bool, "PAUSE":bool, "STOP":bool} {"PLAY"=FALSE, "PAUSE"=FALSE, "STOP"=FALSE} ("PBR_PLAY")) -> ()
                    n1210 = local write "source"("" ("source")) -> ()
                    n1211 = property on="PBR PROC" class="CmbBox"("Strings[]"=w2232, "Value"="" ("source")) -> ()  [unwired: 2 in, 2 out]
                  }
                  frame #6 {
                    n1212 = global read "globals-engine.vi" "Q-Log"() -> (w2235:refnum<queue>)
                    n1213 = for {
                      tunnel: cluster{"data":variant, "Enum":T56}[] [{"data"=variant, "Enum"=enum."LOG.INIT"}, {"data"=variant, "Enum"=enum."LOG.UPDATE.IRR"}] ("procQ") -> [w2240] mode=indexing
                      shift-right: [w2238] -> w2234
                      shift-left: _ -> [w2237]
                      tunnel: w2235 -> [w2239]
                      n1214 = Enqueue Element(queue=w2239, element=w2240, error in (no error)=w2237) -> (error out=w2238:errorcluster)  [unwired: 1 in, 2 out]
                    }
                  }
                }
                n1215 = local write "ENG ms ctrl"(w2105) -> ()
                n1216 = local write "ENV"(w2104) -> ()
                n1217 = local write "ProjectSettings"(w2103) -> ()
                n1218 = global write "globals-engine.vi" "ProjectSettings"(w2103) -> ()
                n1219 = local write "AuxiliaryList"(w2108) -> ()
                n1220 = global write "globals-engine.vi" "NutritionConfiguration"(w2107) -> ()
                n1221 = local write "IRR Params"(w2102) -> ()
                n1222 = global write "globals-engine.vi" "IRR Params"(w2102) -> ()
                n1223 = local write "projectName"(w2106) -> ()
                n1224 = Merge Errors(w2109, w2112, w2111, w2110, w2101, w2100) -> (w2113:errorcluster)
              }
              frame "ENG.INIT.SERIAL" {
                # "initialize:\nGlobals (nutritionConf)\nSerial port\ncall ENG.IO.LOAD"
                n1225 = disable-structure shown="Enabled" {
                  disable-tunnel: [w2249 _] -> w2242
                  frame Disabled {
                    w2245 = T58[] [enum."INI.ENG.SERIAL"] items=["INI.PROJECT_NAME", "INI.ENV", "INI.ENG.SERIAL", "INI.ENG.INTERVAL_MS", "INI.LOCAL.LONGITUDE", "INI.LOCAL.LATITUDE", "INI.LOCAL.TIMEZONE"] ("keys")
                    n1226 = feedback #4() -> ()  [unwired: 2 in]
                    n1227 = feedback-in #4() -> ()  [unwired: 1 out]
                    n1228 = call "util.file.ini.vi"("Section"="LOCAL" ("element"), "keys"=w2245) -> ("values"=w2246:string[])  [unwired: 7 in, 2 out]
                    n1229 = disable-structure shown="Disabled" {
                      frame Disabled {
                        n1230 = case shown="Error .." {
                          selector: _ -> [w2250 _]
                          tunnel: [w2250 w2251] -> _
                          frame No Error {
                          }
                          frame Error {
                            w2253 = T98 2 items=["Canonical Names Only"=0, "Aliases Only"=2, "Include Matching Aliases"=3, "Include All Aliases"=4] ("Search Mode")
                            # "TODO auto scan serial port"
                            n1231 = VISA Find Resource(10:w2253) -> (3:w2254:string[])  [unwired: 2 in, 2 out]
                            n1232 = Reverse 1D Array(array=w2254) -> (reversed array=w2252:string[])
                            n1233 = for {
                              tunnel: w2252 -> [w2255] mode=indexing
                              tunnel: [w2256] -> w2251
                              shift-right: [w2255] -> _
                              shift-left: _ -> [_]
                              stop <- w2256 continue-if-true
                              n1234 = call "util-serial-init.vi"("NewVal"=w2255) -> ("error out"=w2256:errorcluster)  [unwired: 10 in]
                            }
                          }
                        }
                      }
                      frame Enabled {
                      }
                    }
                    n1235 = Index Array(array=w2246) -> (element=w2248:string)  [unwired: 1 in]
                    n1236 = call "util-serial-init.vi"("NewVal"=w2248, "Port"=w2248) -> ("error out"=w2243:errorcluster)  [unwired: 9 in]
                    n1237 = property on="SerialPort" class="VISAName"(error in=w2243, "Value"=w2248) -> (error out=w2247:errorcluster)  [unwired: 1 in, 1 out]
                    n1238 = Merge Errors(w2247) -> (w2249:errorcluster)
                  }
                  frame Enabled {
                    n1239 = call "util-path.vi"("Create Folders?(F)"=FALSE, "Selected Folder (PROCS)"=typePathSelector."DIR_INI" ("Selected Folder (PROCEDURE_DIR)")) -> ("error out"=w2269:errorcluster, "SelectedPath"=w2267:path)  [unwired: 5 in, 3 out]
                    n1240 = call <vilib>:"Open Config Data.vi"("error in (no error)"=w2269, "configuration file path"=w2267) -> ("error out"=w2268:errorcluster, "refnum"=w2266:T63)  [unwired: 7 in, 1 out]
                    n1241 = call "util-ini-key.vi"("key"=ini-key."INI.ENG.SERIAL" ("input 1")) -> ("key"=w2263:string, "section"=w2262:string)  [unwired: 9 in]
                    n1242 = call-poly <vilib>:"Read Key.vi"("section"=w2262, "error in (no error)"=w2268, "key"=w2263, "refnum"=w2266) -> ("error out"=w2265:errorcluster, "value"=w2258:string, "found?"=w2257:bool, "refnum out"=w2264:T63)  [unwired: 4 in]
                    n1243 = case shown="True" w2257 {
                      tunnel: w2258 -> [_ w2270]
                      frame False {
                      }
                      frame True {
                        n1244 = property on="SerialPort" class="VISAName"("Val(Sgnl)"=w2270) -> ()  [unwired: 2 in, 2 out]
                      }
                    }
                    n1245 = call <vilib>:"Close Config Data.vi"("error in (no error)"=w2265, "refnum"=w2264) -> ()  [unwired: 8 in, 2 out]
                  }
                }
              }
              frame "ENG.IO.LOAD" {
                # "let the LOG.status update IOconf local variable so search can work\nwithout the need to trigger io-reg for the io list"
                # "\"ENG.LOAD\" \n load i/o from filesystem to global variable"
                n1246 = Variant To Data(type=T42[] [] ("IO Conf"), Variant=w2276) -> (data=w2275:T42[], error out=w2274:errorcluster)  [unwired: 1 in]
                n1247 = case shown="Error .." w2274 {
                  tunnel: [w2288 w2293] -> w2280
                  tunnel: [_ w2292] -> w2279
                  tunnel: w2275 -> [w2288 _]
                  frame No Error {
                    # "read from Queue"
                  }
                  frame Error {
                    # "read from fs"
                    n1248 = call "util-path.vi"("Selected Folder (PROCS)"=typePathSelector."DIR_IO_FILE") -> ("error out"=w2289:errorcluster, "SelectedPath"=w2290:path)  [unwired: 6 in, 3 out]
                    n1249 = call "util-io-csv-load.vi"("error in"=w2289, "file path (dialog if empty)"=w2290) -> ("error out"=w2292:errorcluster, "Array"=w2293:T42[])  [unwired: 8 in]
                  }
                }
                n1250 = call "variantCtrlIo.vi"("menu (Get Param)"=enumVarCtrlIO."IO Remove All" ("menu (get)"), "error in"=w2279) -> ("error out"=w2277:errorcluster)  [unwired: 5 in, 4 out]
                n1251 = for {
                  tunnel: w2280 -> [w2294] mode=indexing
                  tunnel: [w2297] -> w2271
                  tunnel: w2277 -> [w2295]
                  stop <- w2297 stop-if-true
                  n1252 = call "variantCtrlIo.vi"("menu (Get Param)"=enumVarCtrlIO."IO Add By Key" ("menu (get)"), "error in"=w2295, "IOnode in"=w2294) -> ("error out"=w2297:errorcluster)  [unwired: 4 in, 4 out]
                }
                n1253 = disable-structure shown="Disabled" {
                  frame Disabled {
                    n1254 = global read "globals-engine.vi" "Q-Log"() -> (w2283:refnum<queue>)
                    n1255 = Enqueue Element(queue=w2283, element=cluster{"data":variant, "Enum":T56} {"data"=variant, "Enum"=enum."LOG.UPDATE.SELECTORS"} ("procQ")) -> ()  [unwired: 2 in, 3 out]
                  }
                  frame Enabled {
                  }
                }
                n1256 = disable-structure shown="Enabled" {
                  disable-tunnel: [w2285 w2287] -> w2272
                  disable-tunnel: w2271 -> [w2284 w2287]
                  frame Disabled {
                    n1257 = call "variantCtrlIo.vi"("menu (Get Param)"=enumVarCtrlIO."IO List Configs", "error in"=w2284) -> ("error out"=w2285:errorcluster)  [unwired: 5 in, 4 out]
                  }
                  frame Enabled {
                  }
                }
              }
              frame "ENG.IO.SAVE" {
                # "TODO add file name or dialog"
                # "\"ENG.LOAD\" \n load i/o from filesystem to global variable"
                n1258 = call "variantCtrlIo.vi"("menu (Get Param)"=enumVarCtrlIO."IO List Configs" ("menu (get)")) -> ("IO Configs List"=w2299:T42[])  [unwired: 6 in, 4 out]
                n1259 = call "util-io-sort.vi"("IO Configs List"=w2299) -> ("Result"=w2303:T42[])  [unwired: 10 in]
                n1260 = Array Size(array=w2303) -> (size(s)=w2302:i32)
                n1261 = call "util-path.vi"("Selected Folder (PROCS)"=typePathSelector."DIR_IO_FILE" ("Selected Folder (PROCEDURE_DIR)")) -> ("error out"=w2306:errorcluster, "SelectedPath"=w2298:path)  [unwired: 6 in, 3 out]
                n1262 = Format Into String(format string="Save %d IO nodes as %s?", w2302, w2298) -> (resulting string=w2301:string)  [unwired: 2 in, 1 out]
                n1263 = Two Button Dialog(message=w2301) -> (T button?=w2300:bool)  [unwired: 2 in]
                n1264 = case shown="True" w2300 {
                  tunnel: w2298 -> [_ w2314]
                  tunnel: w2306 -> [w2310 w2313]
                  tunnel: [w2310 w2312] -> w2305
                  tunnel: w2303 -> [_ w2311]
                  frame False {
                  }
                  frame True {
                    n1265 = call "util-io-csv-save.vi"("error out"=w2313, "file path (dialog if empty)"=w2314, "IO Nodes"=w2311) -> ("error out"=w2312:errorcluster)  [unwired: 8 in]
                  }
                }
              }
              frame "ENG.LOAD" {
                # "\"ENG.LOAD\" \nLoads all procs from filesystem as it should be loaded in production (read all procs from procedure folder)"
                n1266 = call "util-path.vi"() -> ("error out"=w2318:errorcluster, "SelectedPath"=w2319:path)  [unwired: 7 in, 3 out]
                n1267 = call <vilib>:"Recursive File List.vi"("error in (no error)"=w2318, "Folder Path"=w2319) -> ("error out"=w2317:errorcluster, "All Files in Dir"=w2316:path[])  [unwired: 5 in, 3 out]
                n1268 = for {
                  tunnel: [w2329] -> w2320 mode=indexing
                  tunnel: [w2325] -> w2315
                  tunnel: w2316 -> [w2323] mode=indexing
                  tunnel: w2317 -> [w2327]
                  stop <- w2325 stop-if-true
                  n1269 = call "util.file.vars.file-operations.vi"("error in (no error)"=w2327, "selected path"=w2323) -> ("error out"=w2326:errorcluster, "Procedure"=w2324:variant[])  [unwired: 7 in, 1 out]
                  n1270 = call "util.proc.init.vi"("error in"=w2326, "Proc Path"=w2323, "Procedure in"=w2324) -> ("error out"=w2325:errorcluster, "Procedure out"=w2328:variant[])  [unwired: 7 in]
                  n1271 = Bundle("Procedure out"=w2328) -> (w2329:cluster{"Procedure out":variant[]})  [unwired: 1 in]
                }
                n1272 = Select(t=cluster{"Procedure":variant[]}[] [], s=w2315, f=w2320) -> (s? t:f=w2322:cluster{"Procedure out":variant[]}[])
                "Loaded" <- w2322
              }
              frame "ENG.LOAD.MODULE" {
                # "\"ENG.LOAD\" \nLoads all procs from filesystem as it should be loaded in production (read all procs from procedure folder)"
                n1273 = Variant To Data(type=path "" ("procPath"), Variant=w2336) -> (data=w2334:path, error out=w2333:errorcluster)  [unwired: 1 in]
                n1274 = call <vilib>:"Recursive File List.vi"("error in (no error)"=w2333, "Folder Path"=w2334) -> ("error out"=w2338:errorcluster, "All Files in Dir"=w2337:path[])  [unwired: 5 in, 3 out]
                n1275 = for {
                  tunnel: [w2346] -> w2330 mode=indexing
                  tunnel: [w2342] -> w2339
                  tunnel: w2337 -> [w2340] mode=indexing
                  tunnel: w2338 -> [w2344]
                  stop <- w2342 stop-if-true
                  n1276 = call "util.file.vars.file-operations.vi"("error in (no error)"=w2344, "selected path"=w2340) -> ("error out"=w2343:errorcluster, "Procedure"=w2341:variant[])  [unwired: 7 in, 1 out]
                  n1277 = call "util.proc.init.vi"("error in"=w2343, "Proc Path"=w2340, "Procedure in"=w2341) -> ("error out"=w2342:errorcluster, "Procedure out"=w2345:variant[])  [unwired: 7 in]
                  n1278 = Bundle("Procedure out"=w2345) -> (w2346:cluster{"Procedure out":variant[]})  [unwired: 1 in]
                }
                n1279 = Build Array (concatenate)(w2332, w2330) -> (w2331:cluster{"Procedure out":variant[]}[])
              }
              frame "ENG.LOAD.RELOAD" {
                # "\"ENG.LOAD.RELOAD\" \nRELOAD THE LAST RUNTIME REGISTER"
                n1280 = local read "Loaded"() -> (w2347:cluster{"Procedure":variant[]}[])
              }
              frame "ENG.LOAD.SINGLE" {
                # "\"ENG.LOAD.SINGLE\"  (PROCEDURE_PATH)\nADD PROCEDURE TO RUNTIME REGISTER"
                n1281 = Variant To Data(type=path "" ("procPath"), Variant=w2358) -> (data=w2348:path, error out=w2349:errorcluster)  [unwired: 1 in]
                n1282 = call "util.file.vars.file-operations.vi"("error in (no error)"=w2349, "selected path"=w2348) -> ("error out"=w2350:errorcluster, "Procedure"=w2351:variant[])  [unwired: 7 in, 1 out]
                n1283 = call "util.proc.init.vi"("error in"=w2350, "Proc Path"=w2348, "Procedure in"=w2351) -> ("error out"=w2353:errorcluster, "Procedure out"=w2354:variant[])  [unwired: 7 in]
                n1284 = Bundle("Procedure out"=w2354) -> (w2357:cluster{"Procedure out":variant[]})  [unwired: 1 in]
                n1285 = case shown="No Error" w2353 {
                  selector: w2353 -> [_ w2367]
                  tunnel: [w2365 w2366] -> w2355
                  tunnel: w2362 -> [w2364 w2366]
                  tunnel: w2357 -> [w2363 _]
                  tunnel: [_ w2367] -> w2356
                  frame No Error {
                    n1286 = Build Array (concatenate)(w2364, w2363) -> (w2365:cluster{"Procedure out":variant[]}[])
                    n1287 = local write "Loaded"(w2365) -> ()
                  }
                  frame Error {
                  }
                }
                n1288 = Enqueue Element(queue=w2361, element=cluster{"cmd":T5, "data":variant} {"cmd"=enum."ENG.STATUS", "data"=variant} ("typedefElement"), error in (no error)=w2356) -> (error out=w2359:errorcluster)  [unwired: 1 in, 2 out]
              }
              frame "ENG.LOAD.UNLOAD" {
                # "\"ENG.LOAD.UNLOAD\" \n REMOVE ALL PROCEDURES FROM RUNTIME REGISTER"
              }
              frame "ENG.PRINT-USER-MSG" {
                # "No code required. used to release th FIFO if waiting indefinitly (-1)"
                n1289 = Variant To Data(type="" ("Value (Signaling)"), Variant=w2371) -> (error out=w2370:errorcluster)  [unwired: 1 in, 1 out]
              }
              frame "ENG.PROC.INSERT-STEPS" {
                # "\"ENG.PROC.INIT\" \nload selected proc from filesystem"
                n1290 = Variant To Data(type=T89 {"ProcName"="", "instructions"=[]}, Variant=w2381) -> (data=w2376:T89, error out=w2379:errorcluster)  [unwired: 1 in]
                n1291 = Unbundle By Name(w2376) -> ("ProcName"=w2373:string, "instructions"=w2374:variant[])
                n1292 = call "main.eng.proc-insert-instructions.vi"("error in (no error)"=w2379, "instructions in"=w2374, "procedureName"=w2373, "procs in"=w2377) -> ("error out"=w2378:errorcluster, "procs out"=w2380:cluster{"Procedure":variant[]}[])  [unwired: 6 in]
              }
              frame "ENG.PROC.ISRUNNING" {
                w2395 = "%s=%s"  # procLabel=ON/OFF
                # "\"ENG-PROC.ISRUNNING\" check if proc is running"
                n1293 = Variant To Data(type=T90 {"callerProc"="", "procPointer"=""}, Variant=w2408) -> (data=w2407:T90)  [unwired: 1 in, 1 out]
                n1294 = Unbundle By Name(w2407) -> ("callerProc"=w2384:string, "procPointer"=w2383:string)
                n1295 = call "util.procs.find-by-name.vi"("ProcName in"=w2383, "Procs in"=w2382) -> ("error out"=w2389:errorcluster, "Found?"=w2402:bool, "procIndex"=w2403:i32)  [unwired: 4 in, 3 out]
                n1296 = call "proc.util.enumToStrProcVar.vi"("Proc var"=typeProcVarientName."procIsRunning" ("Combo Box")) -> ("String"=w2404:string)  [unwired: 10 in]
                n1297 = case shown="True" w2402 {
                  selector: w2402 -> [w2420 _]
                  tunnel: [w2421 w2428] -> w2385
                  tunnel: w2382 -> [w2421 w2427]
                  tunnel: w2404 -> [_ w2423]
                  tunnel: w2403 -> [_ w2425]
                  tunnel: [w2419 w2426] -> w2388
                  tunnel: [w2420 w2422] -> w2394
                  tunnel: w2389 -> [w2419 w2424]
                  frame False {
                  }
                  frame True {
                    n1298 = call "procs.setByProcIndexBoolean.vi"("procIndex"=w2425, "error in"=w2424, "procAttribute"=w2423, "procs in"=w2427) -> ("error out"=w2426:errorcluster, "Bool out"=w2422:bool, "procs out"=w2428:cluster{"Procedure":variant[]}[])  [unwired: 5 in]
                  }
                }
                n1299 = Select(t="ON" ("format string"), s=w2394, f="OFF" ("format string")) -> (s? t:f=w2391:string)
                n1300 = call "util.procs.find-by-name.vi"("error in"=w2388, "ProcName in"=w2384, "Procs in"=w2385) -> ("error out"=w2387:errorcluster, "Found?"=w2397:bool, "procIndex"=w2398:i32)  [unwired: 3 in, 3 out]
                n1301 = Format Into String(format string=w2395, w2383, w2391) -> (resulting string=w2390:string)  [unwired: 2 in, 1 out]
                n1302 = call "proc.util.enumToStrProcVar.vi"("Proc var"=typeProcVarientName."procRegisterString" ("Combo Box")) -> ("String"=w2401:string)  [unwired: 10 in]
                n1303 = Merge Errors(w2387) -> (w2386:errorcluster)
                n1304 = case shown="True" w2397 {
                  tunnel: [w2410 w2418] -> w2399
                  tunnel: w2385 -> [w2410 w2417]
                  tunnel: w2401 -> [_ w2412]
                  tunnel: w2398 -> [_ w2413]
                  tunnel: [w2409 w2416] -> w2396
                  tunnel: w2386 -> [w2409 w2415]
                  tunnel: w2390 -> [_ w2411]
                  frame False {
                  }
                  frame True {
                    n1305 = call "procs.setByProcIndexString.vi"("menu in (get)"=enum16{"get", "set"}."set", "procIndex"=w2413, "error in"=w2415, "String in"=w2411, "procAttribute"=w2412, "procs in"=w2417) -> ("error out"=w2416:errorcluster, "procs out"=w2418:cluster{"Procedure":variant[]}[])  [unwired: 3 in, 1 out]
                  }
                }
              }
              frame "ENG.PROC.PRESET" {
                # "\"ENG.PROC.PRESET\" copy template as procedure (used to change device modes)"
                n1306 = disable-structure shown="Enabled" {
                  disable-tunnel: w2432 -> [w2448 _]
                  disable-tunnel: w2431 -> [w2446 _]
                  disable-tunnel: [w2441 _] -> w2429
                  frame Disabled {
                    # "procedure can be configured to reset itself every completion or be reset immidiatly"
                    n1307 = local read item#-1() -> (w2444)
                    n1308 = Variant To Data(type=w2444, Variant=w2448) -> (data=w2447, error out=w2439:errorcluster)  [unwired: 1 in]
                    n1309 = Unbundle By Name(w2447) -> ("Immidiate"=w2445, "ProcName"=w2435, "Preset File"=w2438)
                    n1310 = call "util.file.vars.vi"("error in"=w2439, "Directory (DIR_PROC)"=typePathSelector."DIR_TEMPLATE" ("Enum"), "Proc Name(open dialog if empty)"=w2438) -> ("error out"=w2434:errorcluster, "Vars[] out"=w2437:variant[])  [unwired: 4 in, 3 out]
                    n1311 = call "util.proc.set-name.vi"("error in"=w2434, "new Proc Name"=w2435, "Procedure in"=w2437) -> ("error out"=w2433:errorcluster, "Procedure out"=w2436:variant[])  [unwired: 7 in]
                    n1312 = call "util.file.vars.vi"("Operation(Read)"=enum16{"Read File", "Write File"}."Write File", "error in"=w2433, "Proc Name(open dialog if empty)"=w2435, "Vars[] in"=w2436) -> ("error out"=w2440:errorcluster)  [unwired: 3 in, 4 out]
                    n1313 = case shown="True" w2445 {
                      tunnel: w2446 -> [_ w2456]
                      tunnel: w2435 -> [_ w2453]
                      tunnel: [w2449 w2451] -> w2441
                      tunnel: w2440 -> [w2449 w2450]
                      frame False {
                      }
                      frame True {
                        n1314 = To Variant(anything=w2453) -> (Variant=w2452:variant)
                        n1315 = Bundle By Name(cluster=cluster{"cmd":T5, "data":variant} {"cmd"=enum."ENG.PROC.RELOAD-BY-NAME", "data"=variant} ("typedefElement"), "data"=w2452) -> (w2455:cluster{"cmd":T5, "data":variant})
                        n1316 = Enqueue Element At Opposite End(queue=w2456, element=w2455, error in (no error)=w2450) -> (error out=w2451:errorcluster)  [unwired: 1 in, 2 out]
                      }
                    }
                  }
                  frame Enabled {
                  }
                }
              }
              frame "ENG.PROC.RELOAD-BY-NAME" {
                w2473 = ""  # procedureName
                # "(3)"
                # "(2)"
                # "(1)"
                # "\"ENG.PROC.RELOAD-BY-NAME\"  (PROCEDURE_NAME)\n(1) SEARCH PROC BY NAME (IN RUNTIME), GET ITS INDEX AND PATH\n(2) LOAD PROCEDURE FROM STORAGE AND INITIALIZE IT\n(3) REPLACE ORIGINAL PROC"
                n1317 = Variant To Data(type=w2473, Variant=w2474) -> (data=w2462:string, error out=w2458:errorcluster)  [unwired: 1 in]
                n1318 = call "util.procs.find-by-name.vi"("isRequired(T)"=FALSE, "error in"=w2458, "ProcName in"=w2462, "Procs in"=w2468) -> ("error out"=w2457:errorcluster, "Found?"=w2466:bool, "procIndex"=w2467:i32, "Proc Path"=w2463:string)  [unwired: 2 in, 2 out]
                n1319 = String To Path(string=w2463) -> (path=w2464:path)
                n1320 = call "util.file.vars.file-operations.vi"("error in (no error)"=w2457, "selected path"=w2464) -> ("error out"=w2470:errorcluster, "Procedure"=w2471:variant[])  [unwired: 7 in, 1 out]
                n1321 = call "util.proc.init.vi"("error in"=w2470, "Proc Path"=w2464, "Procedure in"=w2471) -> ("error out"=w2461:errorcluster, "Procedure out"=w2472:variant[])  [unwired: 7 in]
                n1322 = Bundle("Procedure out"=w2472) -> (w2465:cluster{"Procedure out":variant[]})  [unwired: 1 in]
                n1323 = case shown="No Error" w2461 {
                  selector: w2461 -> [_ w2480]
                  tunnel: [w2478 w2479] -> w2469
                  tunnel: w2468 -> [w2477 w2479]
                  tunnel: w2467 -> [w2476 _]
                  tunnel: w2465 -> [w2475 _]
                  tunnel: w2466 -> [_ _]
                  tunnel: [_ w2480] -> w2460
                  frame No Error {
                    n1324 = Replace Array Subset(array=w2477, new element=w2475, index=w2476) -> (w2478:cluster{"Procedure":variant[]}[])
                  }
                  frame Error {
                  }
                }
              }
              frame "ENG.PROC.START" {
                # "\"ENG-PROC.START\"  find proc and set its procIsRuning attribute"
                n1325 = Variant To Data(type="" ("procName"), Variant=w2490) -> (data=w2481:string)  [unwired: 1 in, 1 out]
                n1326 = Bundle By Name(cluster=T91 {"operation"=enum."START", "procName"=""}, "procName"=w2481) -> (w2484:T91)
                n1327 = call "main.eng.proc-start.vi"("params in"=w2484, "Procs in"=w2488) -> ("error out"=w2487:errorcluster, "Procs out"=w2489:cluster{"Procedure":variant[]}[])  [unwired: 7 in, 1 out]
                n1328 = Format Into String(format string="Start Procedure %s", w2481) -> (resulting string=w2482:string)  [unwired: 2 in, 1 out]
              }
              frame "ENG.PROC.STOP" {
                # "\"ENG-PROC.START\"  find proc and set its procIsRuning attribute"
                n1329 = Variant To Data(type="" ("procName"), Variant=w2500) -> (data=w2491:string)  [unwired: 1 in, 1 out]
                n1330 = Bundle By Name(cluster=T91 {"operation"=enum."STOP", "procName"=""}, "procName"=w2491) -> (w2494:T91)
                n1331 = call "main.eng.proc-start.vi"("params in"=w2494, "Procs in"=w2498) -> ("error out"=w2497:errorcluster, "Procs out"=w2499:cluster{"Procedure":variant[]}[])  [unwired: 7 in, 1 out]
                n1332 = Format Into String(format string="Stop Procedure %s", w2491) -> (resulting string=w2492:string)  [unwired: 2 in, 1 out]
              }
              frame "ENG.RIO.SNAPSHOT" {
                # "\"ENG.RIO.SNAPSHOT\""
                n1333 = Variant To Data(type=u8[] [], Variant=w2507) -> (error out=w2504:errorcluster)  [unwired: 1 in, 1 out]
                n1334 = call <vilib>:"Clear Errors.vi"("error in (no error)"=w2504) -> ()  [unwired: 5 in, 2 out]
                n1335 = local read "RIO List"() -> (w2502:cluster{"Address":u8, "Connected":bool}[])
                n1336 = call "helper-snapshot.vi"("RIO List"=w2502) -> ("Snapshot"=w2503:T13[])  [unwired: 10 in]
                "RIO Snapshots" <- w2503
                n1337 = for {
                  tunnel: w2503 -> [w2514] mode=indexing
                  tunnel: w2502 -> [w2513] mode=indexing
                  tunnel: [w2512] -> w2501 mode=indexing
                  workers-P: _ -> [_]
                  n1338 = Unbundle By Name(w2514) -> ("status.status"=w2511:bool)
                  n1339 = Not(x=w2511) -> (.not. x?=w2510:bool)
                  n1340 = in-place {
                    in-place-border: w2510 -> [w2515]
                    n1341 = in-place-cluster #5(w2513) -> ()  [unwired: 1 out]
                    n1342 = in-place-cluster #5("Connected"=w2515) -> (w2512:cluster{"Address":u8, "Connected":bool})
                  }
                }
                n1343 = disable-structure shown="Enabled" {
                  disable-tunnel: w2503 -> [w2517 _]
                  disable-tunnel: [w2516 _] -> w2508
                  frame Enabled {
                    n1344 = global read "globals-engine.vi" "Q-Log"() -> (w2518:refnum<queue>)
                    n1345 = Bundle By Name(cluster=cluster{"data":variant, "Enum":T56} {"data"=variant, "Enum"=enum."LOG.SNAPSHOT"} ("procQ"), "data"=w2517) -> (w2520:cluster{"data":variant, "Enum":T56})
                    n1346 = Enqueue Element(queue=w2518, element=w2520) -> (error out=w2519:errorcluster)  [unwired: 2 in, 2 out]
                    n1347 = call <vilib>:"Clear Errors.vi"("error in (no error)"=w2519) -> ("error out"=w2516:errorcluster)  [unwired: 5 in, 1 out]
                  }
                  frame Disabled {
                  }
                }
                n1348 = local write "RIO List"(w2501) -> ()
              }
              frame "ENG.RIO.AIN-SNAPSHOT-CALIB" {
                # "\"ENG.RIO.READ-AIN\"  (RIO_ADDRESS)\nREAD ALL ANALOG INPUTS OF A RIO"
                n1349 = local read "IO calib select"() -> (w2527:string)
                n1350 = call "io.interface.vi"("Caller"="ENG.RIO.AIN-SNAPSHOT-CALIB", "IO Name in"=w2527) -> ("error out"=→"error":errorcluster, "unCalibrated"=w2524:u16, "Value out"=w2523:dbl)  [unwired: 4 in, 3 out]
                "Raw (X)" <- w2524
                "Value (Y)" <- w2523
                n1351 = Bundle("unCalibrated"=w2524, "Value out"=w2523) -> (→"Chart":cluster{"unCalibrated":u16, "Value out":dbl})  [unwired: 1 in]
              }
              frame "ENG.RIO.DOUT-BY-ADDR" {
                # "\"ENG.RIO.READ-AIN\"  (RIO_ADDRESS)\nREAD ALL ANALOG INPUTS OF A RIO"
                n1352 = Variant To Data(type=cluster{"State":bool, "ADDR":T8, "Timeout":u8} {"State"=FALSE, "ADDR"=8, "Timeout"=8} ("digitalPort"), Variant=w2553) -> (data=w2545:cluster{"State":bool, "ADDR":T8, "Timeout":u8})  [unwired: 1 in, 1 out]
                n1353 = Unbundle By Name(w2545) -> ("ADDR"=w2532:T8, "State"=w2533:bool, "Timeout"=w2549:u8)
                n1354 = Bundle By Name(cluster=cluster{"state":bool, "timeoutSeconds":u16} {"state"=FALSE, "timeoutSeconds"=0} ("output cluster"), "state"=w2533, "timeoutSeconds"=w2549) -> (w2550:cluster{"state":bool, "timeoutSeconds":u16})
                n1355 = Bundle By Name(cluster=T42 {"ADDR"=2, "Label"="", "Type"=enum."DO", "Mode"=enum."RIO", "Value"="1:1", "Tags"="", "calibration"=[]} ("IoConf in 2"), "Type"=enum.io.type."DO" ("type"), "ADDR"=w2532) -> (w2548:T42)
                n1356 = To Variant(anything=w2550) -> (Variant=w2546:variant)
                n1357 = call "io.interface.serial.vi"("IoConf in"=w2548, "Caller"="ENG.RIO.DOUT-BY-ADDR", "Output State"=w2546) -> ("error out"=w2543:errorcluster)  [unwired: 7 in, 5 out]
                n1358 = disable-structure shown="Enabled" {
                  disable-tunnel: w2543 -> [w2556 w2559]
                  disable-tunnel: [w2555 w2559] -> w2534
                  frame Disabled {
                    n1359 = global read "globals-engine.vi" "Q-Eng"() -> (w2558:refnum<queue>)
                    n1360 = Enqueue Element(queue=w2558, element=cluster{"case":T5, "data":variant} {"case"=enum."ENG.RIO.SNAPSHOT", "data"=variant}, error in (no error)=w2556) -> (error out=w2555:errorcluster)  [unwired: 1 in, 2 out]
                  }
                  frame Enabled {
                  }
                }
                n1361 = Select(t="Set DO " ("format string"), s=w2533, f="Clear DO " ("format string")) -> (s? t:f=w2535:string)
                n1362 = property on="Timer Reset?" class="Bool (strict)"("Val(Sgnl)"=TRUE ("Value (Signaling)")) -> ()  [unwired: 2 in, 2 out]
                n1363 = Format Into String(format string=" %04d", w2532) -> (resulting string=w2536:string)  [unwired: 2 in, 1 out]
                n1364 = Select(t="Error " ("format string"), s=w2534, f="" ("format string")) -> (s? t:f=w2539:string)
                n1365 = Concatenate Strings(w2539, w2535, w2536) -> (w2531:string)
              }
              frame "ENG.RIO.DOUT-BY-NAME" {
                # "\"ENG.RIO.READ-AIN\"  (RIO_ADDRESS)\nREAD ALL ANALOG INPUTS OF A RIO"
                n1366 = Variant To Data(type=T92 {"State"=FALSE, "Timeout"=0, "Name"=""} ("Cluster"), Variant=w2579) -> (data=w2576:T92)  [unwired: 1 in, 1 out]
                n1367 = Unbundle By Name(w2576) -> ("Name"=w2562:string, "State"=w2565:bool, "Timeout"=w2575:u16)
                n1368 = Select(t="Set DO " ("format string"), s=w2565, f="Clear DO " ("format string")) -> (s? t:f=w2564:string)
                n1369 = Bundle By Name(cluster=cluster{"state":bool, "timeoutSeconds":u16} {"state"=FALSE, "timeoutSeconds"=0} ("output cluster"), "state"=w2565, "timeoutSeconds"=w2575) -> (w2574:cluster{"state":bool, "timeoutSeconds":u16})
                n1370 = To Variant(anything=w2574) -> (Variant=w2578:variant)
                n1371 = call "io.interface.vi"("Caller"="ENG.RIO.DOUT-BY-NAME", "IO Value"=w2578, "IO Name in"=w2562) -> ("error out"=w2569:errorcluster)  [unwired: 3 in, 5 out]
                n1372 = Select(t="Error " ("format string"), s=w2569, f="" ("format string")) -> (s? t:f=w2568:string)
                n1373 = disable-structure shown="Enabled" {
                  disable-tunnel: w2569 -> [w2582 w2586]
                  disable-tunnel: [w2581 w2585] -> w2572
                  frame Disabled {
                    n1374 = global read "globals-engine.vi" "Q-Eng"() -> (w2584:refnum<queue>)
                    n1375 = Enqueue Element(queue=w2584, element=cluster{"case":T5, "data":variant} {"case"=enum."ENG.RIO.SNAPSHOT", "data"=variant}, error in (no error)=w2582) -> (error out=w2581:errorcluster)  [unwired: 1 in, 2 out]
                  }
                  frame Enabled {
                    n1376 = call <vilib>:"Clear Errors.vi"("error in (no error)"=w2586) -> ("error out"=w2585:errorcluster)  [unwired: 5 in, 1 out]
                  }
                }
                n1377 = Concatenate Strings(w2568, w2564, w2562) -> (w2563:string)
                n1378 = property on="Timer Reset?" class="Bool (strict)"("Val(Sgnl)"=TRUE ("Value (Signaling)")) -> ()  [unwired: 2 in, 2 out]
              }
              frame "ENG.RIO.RFS-DELAY-SET-X8" {
                n1379 = local read "RFS Delays"() -> (w2588:T35)
                n1380 = for {
                  N: 8 -> [_]
                  tunnel: [w2594] -> w2590
                  tunnel: w2588 -> [w2593]
                  tunnel: "RFS Address" -> [w2592]
                  i -> [w2595]
                  stop <- w2594 stop-if-true
                  w2602 = u8 5  # Datasize
                  w2603 = u8 96  # Command
                  w2613 = "%s RIO[%d] %s %s"  # TIME RIO[i] OPERATION STATUS
                  w2616 = T42 {"ADDR"=0, "Label"="", "Type"=enum."Type", "Mode"=enum."RIO", "Value"="", "Tags"="", "calibration"=[]}  # IoConf in 2
                  n1381 = Unbundle By Name(w2593) -> ("Delay Y"=w2604:u8, "Delay X1"=w2605:u8, "Delay X2"=w2606:u8, "Delay CT"=w2607:u8)
                  n1382 = Bundle(cluster=T93 {"DataSize"=0, "Address"=0, "CMD"=0, "Table Index"=0, "Delay Y"=0, "Delay X1"=0, "Delay X2"=0, "Delay CT"=0}, "DataSize"=w2602, "Address"=w2592, "CMD"=w2603, "Table Index"=w2595, "Delay Y"=w2604, "Delay X1"=w2605, "Delay X2"=w2606, "Delay CT"=w2607) -> (w2601:T93)
                  n1383 = Flatten To String(anything=w2601) -> (data string=w2600:string, error out=w2599:errorcluster)  [unwired: 3 in, 1 out]
                  n1384 = Format Into String(format string="Set Delays for Table[%d]", w2595) -> (resulting string=w2596:string)  [unwired: 2 in, 1 out]
                  n1385 = call "io.frame.vi"("error in"=w2599, "Frameless Command"=w2600) -> ("error out"=w2620:errorcluster, "Framed Command"=w2621:string)  [unwired: 8 in]
                  n1386 = call "io.visa.vi"("operation in (wr-rd)"=enum.io-interface."IO_VISA_WR-RD" ("operation"), "preReadMsDelay"=u32 150, "error in (no error)"=w2620, "write buffer"=w2621) -> ("error out"=w2619:errorcluster, "read buffer"=w2617:string)  [unwired: 4 in, 2 out]
                  n1387 = call "io.responseValidator.vi"("error in"=w2619, "ResponsToValidate in"=w2617, "IoConf in 2"=w2616) -> ("error out"=w2594:errorcluster)  [unwired: 7 in, 1 out]
                  n1388 = Select(t="Failed", s=w2594, f="Succeeded ") -> (s? t:f=w2598:string)
                  n1389 = Get Date/Time String(want seconds? (F)=TRUE) -> (time string=w2612:string)  [unwired: 2 in, 1 out]
                  n1390 = Format Into String(format string=w2613, w2612, w2592, w2596, w2598) -> (resulting string=w2609:string)  [unwired: 2 in, 1 out]
                  n1391 = local write "RFS Status"(w2609) -> ()
                }
              }
              frame "ENG.RIO.RFS-DELAY-SET-X1" {
                w2632 = u8 5  # Datasize
                w2633 = u8 96  # Command
                w2642 = "%s RIO[%d] %s %s"  # TIME RIO[i] OPERATION STATUS
                w2645 = T42 {"ADDR"=0, "Label"="", "Type"=enum."Type", "Mode"=enum."RIO", "Value"="", "Tags"="", "calibration"=[]}  # IoConf in 2
                n1392 = local read "RFS Address"() -> (w2628:u8)
                n1393 = local read "TableIndex"() -> (w2624:u8)
                n1394 = Unbundle By Name("RFS Delays") -> ("Delay Y"=w2634:u8, "Delay X1"=w2635:u8, "Delay X2"=w2636:u8, "Delay CT"=w2637:u8)
                n1395 = Bundle(cluster=T93 {"DataSize"=0, "Address"=0, "CMD"=0, "Table Index"=0, "Delay Y"=0, "Delay X1"=0, "Delay X2"=0, "Delay CT"=0}, "DataSize"=w2632, "Address"=w2628, "CMD"=w2633, "Table Index"=w2624, "Delay Y"=w2634, "Delay X1"=w2635, "Delay X2"=w2636, "Delay CT"=w2637) -> (w2631:T93)
                n1396 = Flatten To String(anything=w2631) -> (data string=w2630:string, error out=w2629:errorcluster)  [unwired: 3 in, 1 out]
                n1397 = Format Into String(format string="Set Delays for Table[%d]", w2624) -> (resulting string=w2625:string)  [unwired: 2 in, 1 out]
                n1398 = call "io.frame.vi"("error in"=w2629, "Frameless Command"=w2630) -> ("error out"=w2649:errorcluster, "Framed Command"=w2650:string)  [unwired: 8 in]
                n1399 = call "io.visa.vi"("operation in (wr-rd)"=enum.io-interface."IO_VISA_WR-RD" ("operation"), "preReadMsDelay"=u32 150, "error in (no error)"=w2649, "write buffer"=w2650) -> ("error out"=w2648:errorcluster, "read buffer"=w2646:string)  [unwired: 4 in, 2 out]
                n1400 = call "io.responseValidator.vi"("error in"=w2648, "ResponsToValidate in"=w2646, "IoConf in 2"=w2645) -> ("error out"=w2651:errorcluster)  [unwired: 7 in, 1 out]
                n1401 = Select(t="Failed", s=w2651, f="Succeeded ") -> (s? t:f=w2627:string)
                n1402 = Get Date/Time String(want seconds? (F)=TRUE) -> (time string=w2641:string)  [unwired: 2 in, 1 out]
                n1403 = Format Into String(format string=w2642, w2641, w2628, w2625, w2627) -> (resulting string=→"RFS Status":string)  [unwired: 2 in, 1 out]
              }
              frame "ENG.RIO.RFS-CYCLES-GET" {
                w2659 = u16 0  # u16
                w2669 = u8 0  # Datasize
                w2670 = u8 97  # Command
                w2676 = "%s RIO[%d] %s %s"  # TIME RIO[i] OPERATION STATUS
                n1404 = local read "RFS Address"() -> (w2665:u8)
                n1405 = Bundle(cluster=cluster{"DataSize":u8, "Address":u8, "CMD":u8} {"DataSize"=0, "Address"=0, "CMD"=0}, "DataSize"=w2669, "Address"=w2665, "CMD"=w2670) -> (w2668:cluster{"DataSize":u8, "Address":u8, "CMD":u8})
                n1406 = Flatten To String(anything=w2668) -> (data string=w2667:string, error out=w2666:errorcluster)  [unwired: 3 in, 1 out]
                n1407 = call "io.frame.vi"("error in"=w2666, "Frameless Command"=w2667) -> ("error out"=w2683:errorcluster, "Framed Command"=w2684:string)  [unwired: 8 in]
                n1408 = call "io.visa.vi"("operation in (wr-rd)"=enum.io-interface."IO_VISA_WR-RD" ("operation"), "preReadMsDelay"=u32 150, "error in (no error)"=w2683, "write buffer"=w2684) -> ("error out"=w2682:errorcluster, "read buffer"=w2680:string)  [unwired: 4 in, 2 out]
                n1409 = call "io.responseValidator.vi"("error in"=w2682, "ResponsToValidate in"=w2680, "IoConf in 2"=T42 {"ADDR"=0, "Label"="", "Type"=enum."Type", "Mode"=enum."RIO", "Value"="", "Tags"="", "calibration"=[]}) -> ("error out"=w2656:errorcluster, "Data out"=w2658:string)  [unwired: 7 in]
                n1410 = Unflatten From String(type=w2659, binary string=w2658, data includes array or string size? (T)=FALSE, error in (no error)=w2656) -> (rest of the binary string=w2660:string, value=→"RFS Cycles":u16, error out=w2661:errorcluster)  [unwired: 1 in]
                n1411 = Select(t="Failed", s=w2656, f="Succeeded ") -> (s? t:f=w2664:string)
                n1412 = for {
                  N: 8 -> [_]
                  shift-right: [w2690] -> _
                  shift-left: w2660 -> [w2692]
                  shift-right: [w2687] -> _
                  shift-left: w2661 -> [w2688]
                  tunnel: [w2686] -> w2655 mode=indexing
                  n1413 = Unflatten From String(type=u16 0, binary string=w2692, data includes array or string size? (T)=FALSE, error in (no error)=w2688) -> (rest of the binary string=w2690:string, value=w2686:u16, error out=w2687:errorcluster)  [unwired: 1 in]
                }
                n1414 = Get Date/Time String(want seconds? (F)=TRUE) -> (time string=w2675:string)  [unwired: 2 in, 1 out]
                n1415 = Format Into String(format string=w2676, w2675, w2665, "Get Cycles" ("format string"), w2664) -> (resulting string=w2672:string)  [unwired: 2 in, 1 out]
                n1416 = Array To Cluster(array=w2655) -> (cluster=→"RFS Cycles Table":T36)
                n1417 = local write "RFS Status"(w2672) -> ()
              }
              frame "ENG.RIO.RFS-ENABLE" {
                (unwired) FALSE ("data includes array or string size? (T)")
                w2708 = u8 1  # Datasize
                w2709 = u8 99  # Command
                w2715 = "%s RIO[%d] %s %s"  # TIME RIO[i] OPERATION STATUS
                (unwired) 8
                n1418 = local read "RFS Address"() -> (w2699:u8)
                n1419 = Cluster To Array(cluster="RFS Enable Table") -> (array=w2698:bool[])
                n1420 = Boolean Array To Number(Boolean array=w2698) -> (number=w2701:u32)
                n1421 = for {
                  tunnel: w2698 -> [w2725] mode=indexing
                  tunnel: [w2726] -> w2697 mode=indexing if=w2725
                  i -> [w2726]
                }
                n1422 = To Unsigned Byte Integer(number=w2701) -> (unsigned 8bit integer=w2700:u8)
                n1423 = Bundle(cluster=T94 {"DataSize"=0, "Address"=0, "CMD"=0, "Enable"=0}, "DataSize"=w2708, "Address"=w2699, "CMD"=w2709, "Enable"=w2700) -> (w2707:T94)
                n1424 = Number To Decimal String(number=w2697) -> (decimal integer string=w2696:string[])  [unwired: 1 in]
                n1425 = call "util.DelimitedStringFromArray.vi"("params array in"=w2696) -> ("delimited string out"=w2693:string)  [unwired: 10 in]
                n1426 = Flatten To String(anything=w2707) -> (data string=w2706:string, error out=w2705:errorcluster)  [unwired: 3 in, 1 out]
                n1427 = call "io.frame.vi"("error in"=w2705, "Frameless Command"=w2706) -> ("error out"=w2722:errorcluster, "Framed Command"=w2723:string)  [unwired: 8 in]
                n1428 = call "io.visa.vi"("operation in (wr-rd)"=enum.io-interface."IO_VISA_WR-RD" ("operation"), "preReadMsDelay"=u32 150, "error in (no error)"=w2722, "write buffer"=w2723) -> ("error out"=w2721:errorcluster, "read buffer"=w2719:string)  [unwired: 4 in, 2 out]
                n1429 = Format Into String(format string="Enable Tables[%s]", w2693) -> (resulting string=w2694:string)  [unwired: 2 in, 1 out]
                n1430 = call "io.responseValidator.vi"("error in"=w2721, "ResponsToValidate in"=w2719, "IoConf in 2"=T42 {"ADDR"=0, "Label"="", "Type"=enum."Type", "Mode"=enum."RIO", "Value"="", "Tags"="", "calibration"=[]}) -> ("error out"=w2703:errorcluster)  [unwired: 7 in, 1 out]
                n1431 = Select(t="Failed", s=w2703, f="Succeeded ") -> (s? t:f=w2704:string)
                n1432 = Get Date/Time String(want seconds? (F)=TRUE) -> (time string=w2714:string)  [unwired: 2 in, 1 out]
                n1433 = Format Into String(format string=w2715, w2714, w2699, w2694, w2704) -> (resulting string=w2711:string)  [unwired: 2 in, 1 out]
                n1434 = local write "RFS Status"(w2711) -> ()
              }
              frame "ENG.RIO.RFS-CYCLES-SET" {
                w2735 = u8 2  # Datasize
                w2736 = u8 98  # Command
                w2742 = "%s RIO[%d] %s %s"  # TIME RIO[i] OPERATION STATUS
                w2745 = T42 {"ADDR"=0, "Label"="", "Type"=enum."Type", "Mode"=enum."RIO", "Value"="", "Tags"="", "calibration"=[]}  # IoConf in 2
                (unwired) 8
                n1435 = local read "RFS Cycles"() -> (w2727:u16)
                n1436 = local read "RFS Address"() -> (w2731:u8)
                n1437 = Bundle(cluster=T95 {"DataSize"=0, "Address"=0, "CMD"=0, "Cycles"=0}, "DataSize"=w2735, "Address"=w2731, "CMD"=w2736, "Cycles"=w2727) -> (w2734:T95)
                n1438 = Flatten To String(anything=w2734) -> (data string=w2733:string, error out=w2732:errorcluster)  [unwired: 3 in, 1 out]
                n1439 = Format Into String(format string="Limit Cycles to %d", w2727) -> (resulting string=w2728:string)  [unwired: 2 in, 1 out]
                n1440 = call "io.frame.vi"("error in"=w2732, "Frameless Command"=w2733) -> ("error out"=w2749:errorcluster, "Framed Command"=w2750:string)  [unwired: 8 in]
                n1441 = call "io.visa.vi"("operation in (wr-rd)"=enum.io-interface."IO_VISA_WR-RD" ("operation"), "preReadMsDelay"=u32 150, "error in (no error)"=w2749, "write buffer"=w2750) -> ("error out"=w2748:errorcluster, "read buffer"=w2746:string)  [unwired: 4 in, 2 out]
                n1442 = call "io.responseValidator.vi"("error in"=w2748, "ResponsToValidate in"=w2746, "IoConf in 2"=w2745) -> ("error out"=w2751:errorcluster)  [unwired: 7 in, 1 out]
                n1443 = Select(t="Failed", s=w2751, f="Succeeded ") -> (s? t:f=w2730:string)
                n1444 = Get Date/Time String(want seconds? (F)=TRUE) -> (time string=w2741:string)  [unwired: 2 in, 1 out]
                n1445 = Format Into String(format string=w2742, w2741, w2731, w2728, w2730) -> (resulting string=w2738:string)  [unwired: 2 in, 1 out]
                n1446 = local write "RFS Status"(w2738) -> ()
              }
              frame "ENG.NO-OP", Default {
              }
            }
            n1447 = call "helper-log-eng.vi"("error in"=w1956, "ARGS"=w1955, "case"=w1958) -> ("error out"=w1957:errorcluster, "Collected Reports"=→"Collected Reports":string)  [unwired: 7 in]
          }
        }
      }
      frame Error {
        # "handle error by displaying a continue/stop message dialog."
        n1448 = call <vilib>:"Clear Errors.vi"("error in (no error)"=w2756) -> ("error out"=w2757:errorcluster)  [unwired: 5 in, 1 out]
        n1449 = Unbundle By Name(w2756) -> ("source"=w2755:string)
      }
    }
    n1450 = case shown="\"\"" w1874 {
      selector: w1874 -> [_ w1889]
      frame "" {
        # "skip empty statuts"
      }
      frame Default {
        # "status register"
        n1451 = call "reg-status.vi"("Operation(Read)"=enum.report-filter."Collect", "Reports to Collect"=w1889) -> ("Collected Reports"=→"User messages":string)  [unwired: 8 in, 1 out]
      }
    }
    n1452 = call "util-collect-error.vi"("error in (no error)"=w1868, "Array in"=w1869) -> ("Array out"=w1867:errorcluster[])  [unwired: 9 in]
    "control" <- w1867
    n1453 = disable-structure shown="Enabled" {
      disable-tunnel: w1870 -> [w1887 _]
      disable-tunnel: [w1886 _] -> w1866
      frame Enabled {
        n1454 = call "eng-error-handler.vi"("Numeric"=w1887) -> ("delta t"=w1886:dbl)  [unwired: 9 in, 1 out]
      }
      frame Disabled {
      }
    }
    n1455 = property on="Waveform Chart" class="WFChart (strict)"("Value"=w1866) -> ()  [unwired: 2 in, 2 out]
    "Eng" <- w1876
  }
  n1456 = Merge Errors(w28) -> (w6:errorcluster)
  n1457 = call <vilib>:"Clear Errors.vi"("error in (no error)"=w6) -> ("error out"=w27:errorcluster)  [unwired: 5 in, 1 out]
  n1458 = call "io.visa.vi"("operation in (wr-rd)"=enum.io-interface."IO_VISA_CLOSE", "error in (no error)"=w27) -> ("error out"=w26:errorcluster)  [unwired: 6 in, 3 out]
  n1459 = disable-structure shown="Enabled" {
    frame Disabled {
      n1460 = feedback #6() -> (w2759)  [unwired: 1 in]
      n1461 = feedback-in #6() -> (w2763)
      n1462 = local write "IO Map AI"(w2763) -> ()
      n1463 = Not Equal?(x=w2763, y=w2759) -> (x != y?=w2764:bool)
      n1464 = Array Max & Min(array=w2764) -> (max index (indices)=w2761:i32, min index (indices)=w2760:i32)  [unwired: 2 out]
      n1465 = Not Equal?(x=w2761, y=w2760) -> (x != y?=w2762:bool)
      n1466 = case shown="True" w2762 {
        tunnel: w2763 -> [_ w2765]
        frame False {
        }
        frame True {
          n1467 = local write "IO Map AI"(w2765) -> ()
        }
      }
    }
    frame Enabled {
    }
  }
  n1468 = call <vilib>:"Clear Errors.vi"("error in (no error)"=w26) -> ("error out"=w16:errorcluster)  [unwired: 5 in, 1 out]
  n1469 = property on="Splitter" class="Splitter"(error in=w16, "Locked"=FALSE ("Splitter Position Locked")) -> ()  [unwired: 1 in, 2 out]
